vi "Tracker_Data_Analysis_tool.vi"(8 "error in (no error)":errorcluster, 11 "Settings file path":path=path "D:/Users/Dmitriy/CData/CloudStation/Tracker_repository/SubVi's/Tracker_settings.tcf") -> (0 "error out":errorcluster)   [LabVIEW 2016]
uses:
  <vilib>/Utility/config.llb/Config Data RefNum.ctl
  <vilib>/Utility/miscctls.llb/LVPoint32TypeDef.ctl
  <vilib>/Utility/miscctls.llb/LVPointTypeDef.ctl
  <vilib>/Utility/miscctls.llb/LVOffsetAndMultiplierTypeDef.ctl
  <vilib>/Utility/miscctls.llb/LVRangeTypeDef.ctl
  <vilib>/Platform/TimedLoop/XDataNode/timing_clust.ctl
  <vilib>/Platform/TimedLoop/XDataNode/nitl_modes.ctl
  <vilib>/Platform/TimedLoop/XDataNode/wakeup.ctl
  <vilib>/Utility/miscctls.llb/LVBoundsTypeDef.ctl
  <vilib>/Utility/miscctls.llb/LVStringsAndValuesArrayTypeDef_U16.ctl
  <vilib>/Instr/_visa.llb/VISA Flush IO Buffer Mask.ctl
  <extravilib>/ChannelInstances/Lossy Stream-a[.,.](str)/Write With Abort.vi
  <extravilib>/ChannelInstances/Lossy Stream-a[.,.](str)/Read With Abort.vi
  <extravilib>/ChannelInstances/Lossy Stream-a[.,.](str)/Endpoint.vi
  SubVi's/SW_Globals.vi
  <vilib>/Platform/TimedLoop/scheduler/LVUserAPI/_suppVIs/Create_1kHz_TSource.vi
  <extravilib>/ChannelInstances/Lossy Stream-a[.,.](str)/Instantiate.vi
  <vilib>/Utility/file.llb/Write Delimited Spreadsheet (string).vi
  <vilib>/Utility/file.llb/Read Delimited Spreadsheet (string).vi
  <extravilib>/ChannelInstances/Lossy Stream-a[.,.](str)/)Channel.vi
  <resource>/ChannelSupport/_ChannelSupport/WaitIfNeeded.vi
  <vilib>/platform/TimedLoop/XDataNode/XDataNode.xnode
  <vilib>/Utility/config.llb/NI_LVConfig.lvlib
  <extravilib>/ChannelInstances/Lossy Stream-a[.,.](str).lvlib
  <vilib>/Platform/TimedLoop/XDataNode/XDNodeRunTimeDep.lvlib
  <vilib>/Analysis/NI_AALBase.lvlib
panel:
  in  "Pause, s":sgl min=0 max=10000 step=0.1 format="%#_3g"
  in  "Stim., s":sgl min=0 max=10000 step=0.1
  in  "Running, s":sgl min=0 max=10000 step=0.1 format="%#_3g"
  in  "Save files First Call":bool=TRUE
  in  "Record start First Call":bool=TRUE
  out "mean 3":dbl format="%0.2f"
  out "standard deviation 3":dbl format="%0.2f"
  out "Save iteration duration":i64
  out "standard deviation":dbl format="%0.2f"
  out "mean":dbl format="%0.2f"
  in  "Type of histogram":u8
  out "TTL 4 counter":u32
  out "TTL 3 counter":u32
  out "TTL 2 counter":u32
  out "TTL 1 counter":u32
  out "Full track plotting":u32
  out "Full track preparation":u32
  out "Main queue":refnum<queue>
  out "Data flow controls":T1
  in  "Map index (analysis)":i32
  in  "Full trace color":u32(colorbox)=16711680
  out "Current TTL status":u8
  out "TTL inputs":u8[](array[numeric])
  out "TTL outputs":u8[](array[numeric])
  out "Start/Stop in config":u32
  out "Start/Stop out pulses config":u32
  out "Changed IO":bool
  out "Sync capability":u8
  in  "IO parameters string":string
  out "Reset STIM":bool
  out "Reset REG":bool
  out "Init plot":bool=TRUE
  out "Zones preference array (loaded)":dbl[][](array[numeric])
  out "Current zone":dbl[](array[numeric])
  out "Absolute timestamp (rec)":dbl[](array[numeric])
  in  "Colors for Stim. setup":T2(array[cluster])=[{"Not Selected"=1143775, "Not Selected"=1143775}, {"Not Selected"=14517504, "Not Selected"=14517504}, {"Not Selected"=1976113, "Not Selected"=1976113}, {"Not Selected"=2575993, "Not Selected"=2575993}]
  out "Record":bool
  out "Stopped":bool
  out "Reset starting pulse":bool
  out "TTL is long enough":bool
  out "Started":bool
  out "Coords":T3={"Horizontal"=316, "Vertical"=127}
  out "Button":u16=1
  out "Settings file path":path
  out "Track path":path
  out "Index of the last recorded timepoint":i32
  out "ceil(x): smallest int >= x":dbl
  out "Application Directory":path
  out "Path to the settings file":path=path "D:/Users/Dmitriy/CData/CloudStation/Tracker_repository/Tracker_settings.tcf"
  out "Eff. save interval":sgl=7.981
  out "Relative timestamp (rec)":dbl[](array[numeric])
  out "alpha rot. angle":dbl[](array[numeric])
  out "Y coord":dbl[](array[numeric])
  out "X coord":dbl[](array[numeric])
  out "Data column names":string[](array[string])
  out "Zones allocation array":i32[](array[numeric])
  out "Zones presence array":bool[](array[boolean])
  in  "Stop Button":bool
  out "Path to the latest saved temp file":path
  out "Temp file ready":bool
  out "Pixels per mm":dbl=1.1663076923076923
  out "Settings file refnum out":T4
  out "Current User":string="Researcher"
  in  "Main tab control":enum32{"Settings", "Recording", "Analysis"}(tab)
  in  "Set advanced stimulus":bool
  in  "Load zones":bool
  in  "Load stimuli":bool
  in  "Load settings":bool
  out "IO status indicator":T5
  in  "Set IO config":bool
  in  "Jump to Analysis":bool
  in  "Reset stimuli":bool
  in  "Stimulus presets":T6(array[cluster]) {"TTL out" items=["1"=1, "2"=2, "1 + 2"=3]; "Stimulus, s" min=0 max=10000 step=0.1; "Time, s" min=0 max=10000 step=0.1; "Event type" items=["Time spent in zone", "Future options"]}
  in  "Zone-based stimulus setup":T7(radio)=enum."Zone 13"
  out "Ready":bool=TRUE
  in  "Re-check HW connection":bool
  in  "Reset regions":bool
  in  "Start Tracking button":bool
  in  "Starting angle BORDER":i16
  in  "N segments BORDER":u8=5 max=8
  in  "N segments MIDFIELD":u8=3 min=1 max=4
  in  "Starting angle MIDFIELD":i16=30
  in  "Radius, mm MIDFIELD":u16=110
  in  "Radius, mm CENTER":u16=50 min=5 step=1
  out "Board size":string="Large"
  in  "Cage diameter, mm":u16(ring)=333 items=["180 mm"=180, "325 mm"=325, "327 mm"=327, "333 mm"=333]
  out "Segments diagram":picture
  out "HW info":string
  out "Port":string="Large"
  out "Run times distrib. indicator":bool
  out "IO pulses count":string
  in  "Bridge swap":bool
  in  "Reset barplot":bool
  out "Mouse speed digi":dbl=0.28949046360238656 caption="Mouse speed" format="%05.1f"
  out "Histograms (normalized)":dbl[](graph)=[0.0, 0.0, 0.0, 0.0, 0.0, 0.0, 1.0, 0.0, 0.0, 0.0, 0.0] caption="Run times dist. hist. (norm.)"
  in  "Multiplyer of chart RX":u8(slide)=1 min=1 max=10 step=1 scale=1.0..6.0
  in  "Zones presence indicator":T8={"01"=TRUE, "02"=TRUE, "03"=TRUE, "04"=TRUE, "05"=TRUE, "06"=TRUE, "07"=TRUE, "08"=TRUE, "09"=TRUE, "10"=TRUE, "11"=TRUE, "12"=TRUE, "13"=TRUE}
  in  "Zones":bool=TRUE
  in  "Record/Stop":bool
  out "Diagram at recording":picture caption="Mouse track"
  in  "Trace, s":u16(slide)=5 max=30 step=1 scale=0.0..30.0
  in  "Data filtering":u16(ring)=5 items=["None"=0, "Kalman 1/3"=2, "Kalman 1/8"=3, "SG 3/5"=4, "SG 3/11"=5, "SG 3/31"=6]
  out "Record timestamp":dbl format="%<%H:%M:%S%3u>t"
  out "Current Time":timestamp=timestamp(3610093053.229 s since 1904-01-01) format="%<%H:%M:%S %d.%m.%Y>T"
  in  "Exit (recording)":bool
  out "Mouse speed":waveform(dbl)(graph)={"t0"=timestamp(3610093053.229 s since 1904-01-01), "dt"=1.0, "Y"=[0.28949046360238656]}
  in  "Vertical offset":sgl caption="Bridge offset" min=-60 max=60 step=0.1 format="%#.1g"
  out "TTL IO 1 (recording)":bool caption="IO 1"
  out "TTL IO 2 (recording)":bool caption="IO 2"
  out "TTL IO 3 (recording)":bool caption="IO 3"
  out "TTL IO 4 (recording)":bool caption="IO 4"
  out "TTL REC":bool
  out "Mouse running, perc. of time":dbl=0.28949046360238656 caption="Run, %" format="%05.2f"
  out "Zones presense indicator":bool
  out "Speed distrib. indicator":bool
  out "Run lengts distrib. indicator":bool
  in  "Back to Settings":bool
  out "Data loading progress":dbl(slide) scale=0.0..100.0
  in  "Speed":u16(ring)=3 items=["25"=75, "10"=30, "6"=18, "4"=12, "2"=6, "1"=3, "2/3"=2, "1/3"=1]
  in  "Timeline":dbl(slide) min=0.0 step=1.0 scale=0.0..2699.993 scale format="%<%H:%M:%S>t"
  in  "Multiplyer of chart RX 2":u8(slide)=1 min=1 max=10 step=1 scale=1.0..6.0
  out "Diagram at analysis":picture caption="Mouse track"
  in  "Play/Pause":bool
  out "Recorded at time":timestamp format="%<%H:%M:%S %d.%m.%Y>T"
  out "Recorded timestamp":dbl format="%<%H:%M:%S%3u>t"
  in  "Zones (analysis)":bool=TRUE caption="Zones"
  out "Mouse speed 2":waveform(dbl)(graph) caption="Mouse speed"
  out "Mouse speed digi 2":dbl format="%05.1f"
  out "Zones allocation (normalized) in analysis":dbl[](graph) caption="Zone preference (normalized)"
  out "Recorded by":string
  in  "Trace in analysis, s":u16(slide)=2 caption="Trace, s" max=30 step=1 scale=0.0..30.0
  in  "Open File":bool
  out "Mouse snout orientation swap (analysis)":bool caption="Swapped"
  in  "Show heatmap (analysis)":bool caption="Heat map"
  in  "Show full track (analysis)":bool caption="Full track"
  out "Vertical offset (analysis)":sgl caption="Br. offset" min=-60 max=60 step=0.1 format="%#.1g"
  out "TTL IO 2 (analysis)":bool
  out "TTL IO 1 (analysis)":bool
  out "TTL IO 3 (analysis)":bool
  out "TTL IO 4 (analysis)":bool
  # "v.2.1.5"
  # "Cage segmentation"
  # "BORDER"
  # "CENTER"
  # "MIDFIELD"
  # "v.2.1.5"
  # "v.2.1.5"
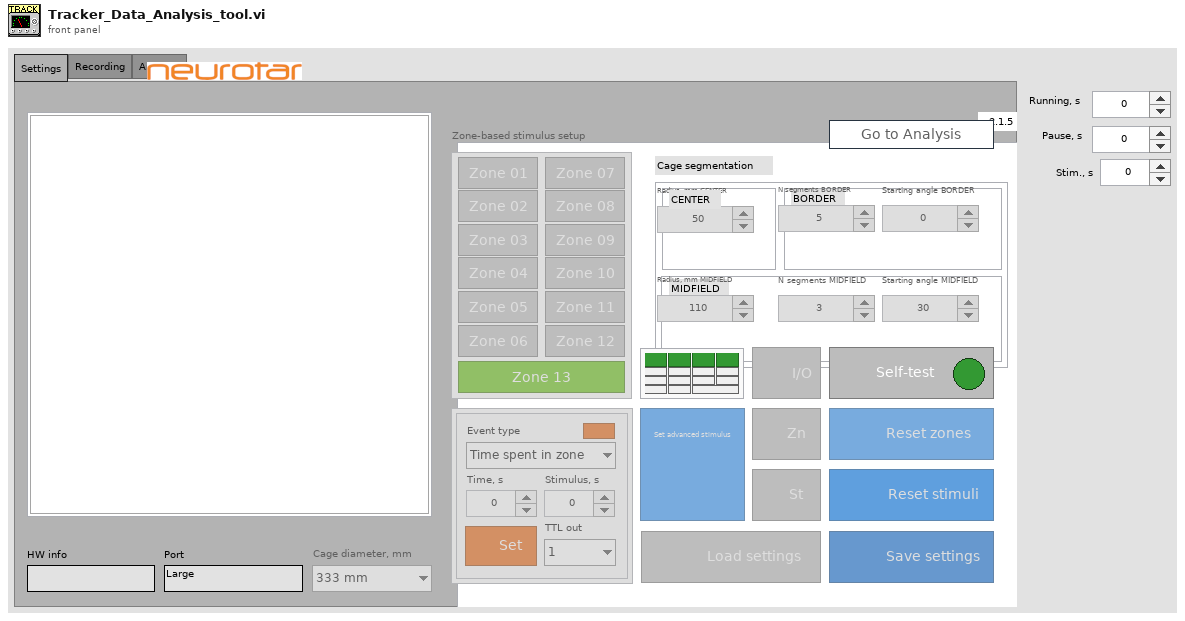
[diagram p1: front panel]
types:
  T1 = cluster{"Data acquisition status":refnum<notifier>, "Play/Pause status":refnum<notifier>, "Complete stop":refnum<notifier>, "Temp file ready for processing":refnum<notifier>, "Has been recorded":refnum<notifier>, "Recording now":refnum<notifier>, "Path to the latest complete temp file":refnum<notifier>, "Final CSV saved":refnum<notifier>, "Data loaded":refnum<notifier>}
  T2 = cluster{"Not Selected":u32, "Not Selected":u32}[]
  T3 = typedef "LVPoint32TypeDef.ctl" = cluster{"Horizontal":i32, "Vertical":i32}
  T4 = typedef "NI_LVConfig.lvlib/Config Data RefNum.ctl" = refnum<k1>
  T5 = cluster{"IO1":bool, "IO2":bool, "IO3":bool, "IO4":bool, "Z1":bool, "Z2":bool, "Z3":bool, "Z4":bool, "St1":bool, "St2":bool, "St3":bool, "St4":bool, "Syn1":bool, "Syn2":bool, "RS-232 ext. activated":bool}
  T6 = cluster{"Event type":u16, "Time, s":sgl, "Stimulus, s":sgl, "Set/Clear":bool, "TTL out":u16, "Stim. has been set":bool}[]
  T7 = enum32{"No Selection", "Zone 01", "Zone 02", "Zone 03", "Zone 04", "Zone 05", "Zone 06", "Zone 07", "Zone 08", "Zone 09", "Zone 10", "Zone 11", "Zone 12", "Zone 13"}
  T8 = cluster{"01":bool, "02":bool, "03":bool, "04":bool, "05":bool, "06":bool, "07":bool, "08":bool, "09":bool, "10":bool, "11":bool, "12":bool, "13":bool}
  T9 = cluster{"Numeric Control":u32, "Numeric Control":u32}[]
  T10 = enum8{"Enabled", "Disabled", "Disabled and Grayed Out"}
  T11 = typedef "XDNodeRunTimeDep.lvlib/timing_clust.ctl" = cluster{"Expected End [f-1]":u64, "Actual End [f-1]":u64, "Finished Late? [f-1]":bool, "Expected End [i-1]":u64, "Actual End [i-1]":u64, "Finished Late? [i-1]":bool, "Expected Start [i]":u64, "Actual Start [i]":u64, "Expected Start [f]":u64, "Actual Start [f]":u64, "Source Name":string, "Structure Name":string, "Period":i64, "Deadline":i64, "Offset":i64, "Start":i64, "Priority":i32, "Timeout":i32, "Mode":T12, "Wakeup Reason":T13, "Error":errorcluster, "Source Type":string, "Secondary Source Type":string, "Global End Time":u64, "Global Start Time":u64, "Frame Duration":u64, "Iteration Duration":u64, "Assigned CPU":i32, "I/O Scan Engine Mode":u32}
  T12 = typedef "XDNodeRunTimeDep.lvlib/nitl_modes.ctl" = enum32{"No Change", "Process missed periods, maintain original phase", "Discard missed periods, maintain original phase", "Process missed periods, ignore original phase", "Discard missed periods, ignore original phase"}
  T13 = typedef "XDNodeRunTimeDep.lvlib/wakeup.ctl" = enum32{"Normal", "Aborted", "Asynchronous wakeup", "Timing source error", "Timed loop error", "Timeout"}
  T14 = cluster{"Read buffer":string, "Timestamp":timestamp}
  T15 = typedef "VISA Flush IO Buffer Mask.ctl" = u16
  T16 = typedef "LVBoundsTypeDef.ctl" = cluster{"Width":u32, "Height":u32}
  T17 = cluster{"Amount of border segments":u8, "Border segments starting angle":i16, "Amount of midfield segments":u8, "Midfield segments starting angle":i16, "Midfield segments outer radius, mm":u16, "Amount of central segments":u8, "Center segment outer radius, mm":u16, "Diameter of the cage, mm":u16, "R-gap between segments, mm":u8}
  T18 = typedef "LVRangeTypeDef.ctl" = cluster{"Minimum":dbl, "Maximum":dbl, "Increment":dbl, "Minor Increment":dbl, "Start":dbl}
  T19 = cluster{"Temporary file output path":path, "Temporary csv output path":path, "Recording settings output path":path, "Final csv output path":path, "Background picture output path":path, "Path to the settings file":path, "Path to TDMS file":path, "TDMS file reference":refnum<k34>}
  T20 = cluster{"Zones preference array (loaded)":dbl[][], "TTL inputs":u8[], "TTL outputs":u8[], "Stimulus presets array (loaded)":cluster{"Event type":u16, "Time, s":sgl, "Stimulus, s":sgl, "Set/Clear":bool, "TTL out":u16, "Stim. has been set":bool}[], "Absolute timestamp":dbl[], "Relative timestamp":dbl[], "X coord":dbl[], "Y coord":dbl[], "alpha rot. angle":dbl[], "Current zone":dbl[], "Acquisition settings cluster out":cluster{"Researcher name":string, "Amount of midfield segments":u32, "Amount of border segments":u32, "Center segment outer radius, mm":u32, "Midfield segments outer radius, mm":u32, "Midfield segments starting angle":i32, "Border segments starting angle":i32, "Cage diameter, mm":u32, "Mouse snout orientation swap?":bool, "Vertical offset":dbl, "Settings loaded OK":bool}, "Data column names":string[]}
  T21 = cluster{"Researcher name":string, "Amount of midfield segments":u32, "Amount of border segments":u32, "Center segment outer radius, mm":u32, "Midfield segments outer radius, mm":u32, "Midfield segments starting angle":i32, "Border segments starting angle":i32, "Cage diameter, mm":u32, "Mouse snout orientation swap?":bool, "Vertical offset":dbl, "Settings loaded OK":bool}
  T22 = cluster{"Fonts scale factor":dbl, "Pixels per mm":dbl, "Radius of displayed outer segments, pix":dbl, "Radius of displayed midfield segments, pix":dbl, "Radius of displayed central segment, pix":dbl}
  T23 = typedef "imagedata.ctl" = cluster{"image type":i32, "image depth":i32, "image":u8[], "mask":u8[], "colors":u32[], "Rectangle":cluster{"left":i16, "top":i16, "right":i16, "bottom":i16}}
  T24 = cluster{"Width":u16, "Style":enum32{"Solid", "Dash", "Dot", "DashDot", "DashDotDot"}}
  T25 = cluster{"N segments BORDER":u8, "Starting angle BORDER":i16, "N segments MIDFIELD":u8, "Starting angle MIDFIELD":i16, "Radius, mm MIDFIELD":u16, "Amount of central segments":u8, "Radius, mm CENTER":u16}
  T26 = typedef "LVOffsetAndMultiplierTypeDef.ctl" = cluster{"Offset":dbl, "Multiplier":dbl}
  T27 = enum32{"No Selection", "Zone 01", "Zone 02", "Zone 03", "Zone 04", "Zone 05", "Zone 06", "Zone 07", "Zone 08", "Zone 09", "Zone 10", "Zone 11", "Zone 12", "Zone 13", "Zone 14"}
  T28 = enum32{"Page Enabled", "Page Disabled", "Page Disabled & Grayed"}
  T29 = typedef "LVPointTypeDef.ctl" = cluster{"Horizontal":i16, "Vertical":i16}
  T30 = enum32{"invalid app kind", "Development System", "Run Time System", "Student Edition", "Embedded LabVIEW", "Evaluation", "Custom"}
  T31 = cluster{"Event type":u16, "Dur., s":sgl, "Stim., s":sgl, "Set/Clear":bool, "TTL out N":u16, "Stim. has been set":bool}[]
  T32 = cluster{"SYNC configuration":u16, "IO 1 configuration":u16, "IO 2 configuration":u16, "IO 3 configuration":u16, "IO 4 configuration":u16, "Activate ext. RS-232":u16, "IO inversion config.":u16}
  T33 = typedef "Lossy Stream-a[.,.](str).lvlib/)Channel.ctl" = refnum<queue>
  T34 = cluster{"Read buffer":string, "Timestamp":timestamp}[]
  T35 = cluster{"Event type":u16, "Cond., s":sgl, "Stim., s":sgl, "Set/Clear":bool, "TTL out N":u16, "Stim. has been set":bool}
  T36 = cluster{"SYNC configuration":bool, "IO 1 configuration":bool, "IO 2 configuration":bool, "IO 3 configuration":bool, "IO 4 configuration":bool, "Activate ext. RS-232":bool, "IO inversion config.":bool}
  T37 = cluster{"Event type":u16, "Time, s":sgl, "Stimulus, s":sgl, "Set/Clear":bool, "TTL out":u16, "Stim. has been set":bool}
  T38 = typedef "LVStringsAndValuesArrayTypeDef_U16.ctl" = cluster{"String":string, "Value":u16}[]
  T39 = cluster{"N segments BORDER":u8, "Starting angle BORDER":i16, "N segments MIDFIELD":u8, "Starting angle MIDFIELD":i16, "Radius, mm MIDFIELD":u16, u8, "Radius, mm CENTER":u16, "Cage diameter, mm":u16, i32}
  T40 = cluster{"N segments BORDER":u8, "Starting angle BORDER":i16, "N segments MIDFIELD":u8, "Starting angle MIDFIELD":i16, "Radius, mm MIDFIELD":u16, "N segments CENTER":u8, "Radius, mm CENTER":u16, "Cage diameter, mm":u16, "R-gap":i32}
  T41 = cluster{"Zone[1]":bool, "Zone[2]":bool, "Zone[3]":bool, "Zone[4]":bool, "Zone[5]":bool, "Zone[6]":bool, "Zone[7]":bool, "Zone[8]":bool, "Zone[9]":bool, "Zone[10]":bool, "Zone[11]":bool, "Zone[12]":bool, "Zone[13]":bool}
  T42 = cluster{"Event type":u16, "Cond., s":sgl, "Stim., s":sgl, "Set/Clear":bool, "TTL out N":u16, "Stim. has been set":bool}[]
  T43 = cluster{"Temporary file output path":path, "Temporary csv output path":path, "Recording settings output path":path, "Final output path":path, "Background picture output path":path, "Path to the settings file":path, "Path to TDMS file":path, "TDMS file reference":refnum<k34>}
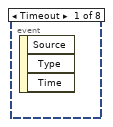
[diagram p5: hidden frame]
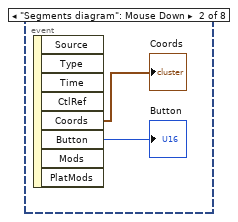
[diagram p6: hidden frame]
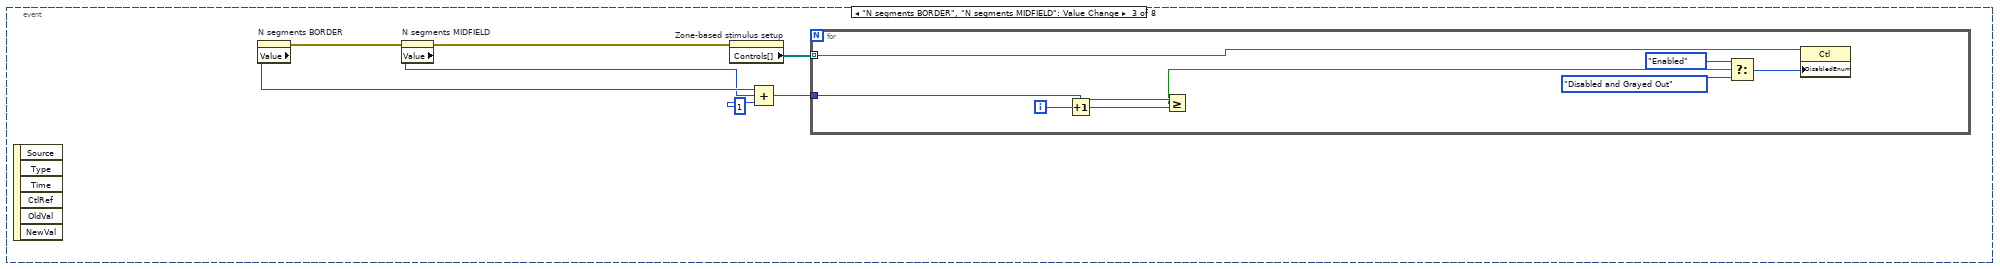
[diagram p7: hidden frame]
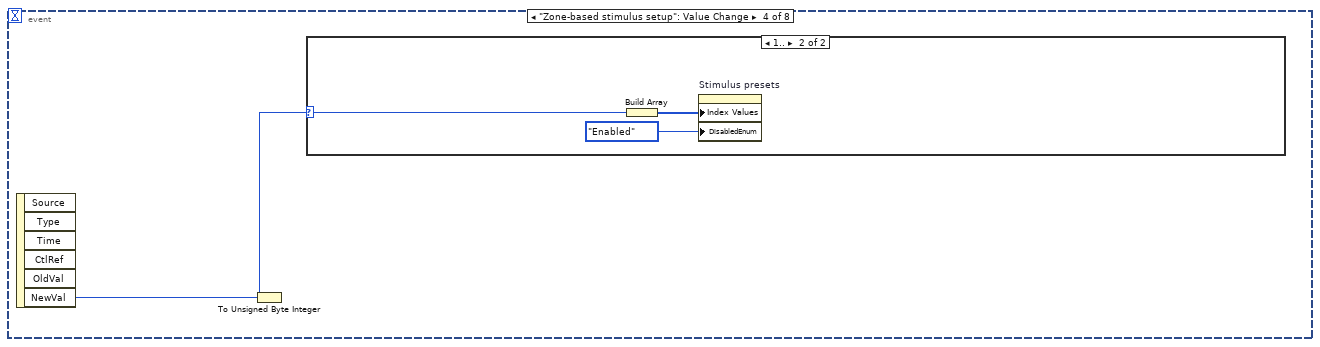
[diagram p8: hidden frame]
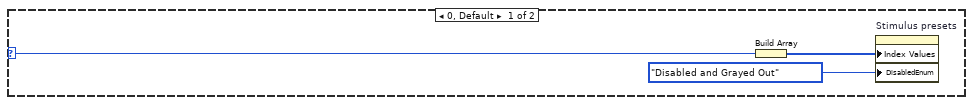
[diagram p9: hidden frame]
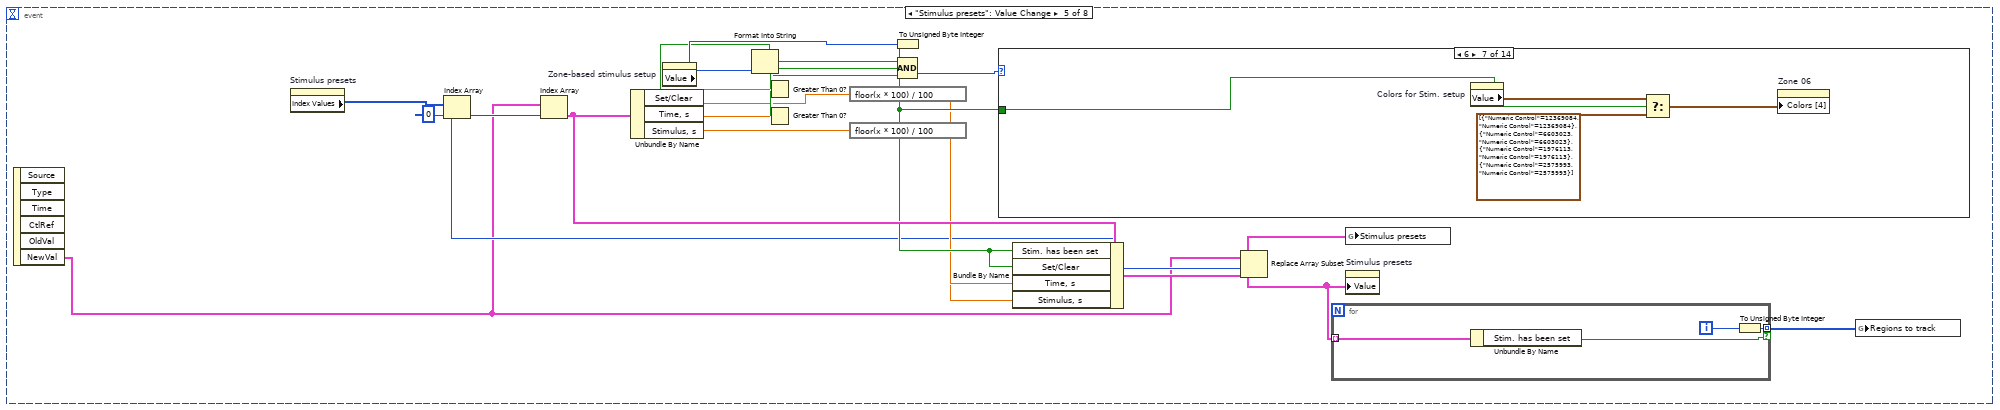
[diagram p10: hidden frame]
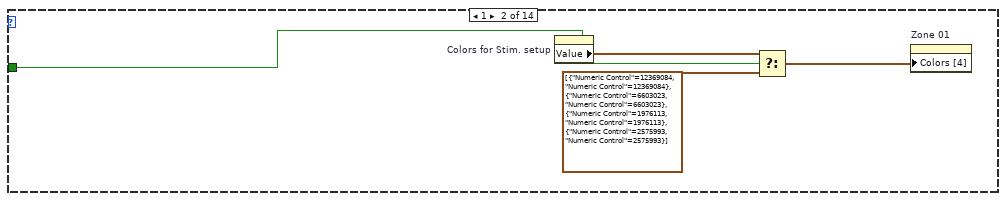
[diagram p12: hidden frame]
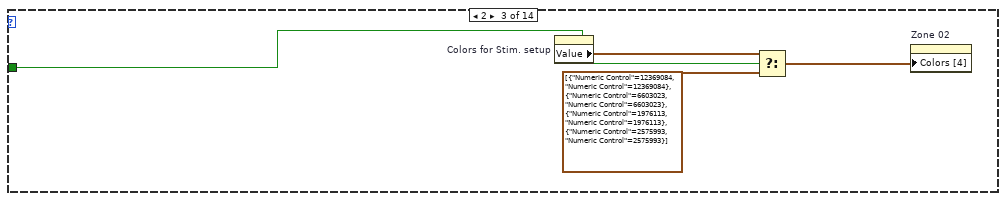
[diagram p13: hidden frame]
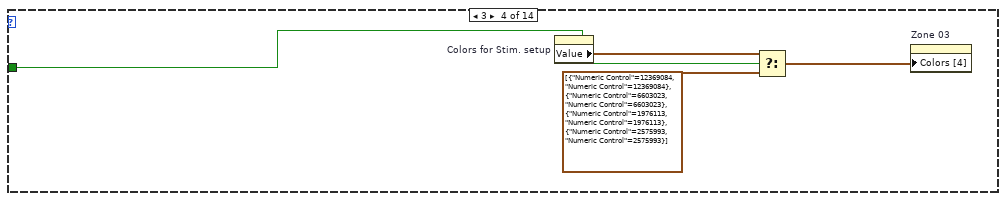
[diagram p14: hidden frame]
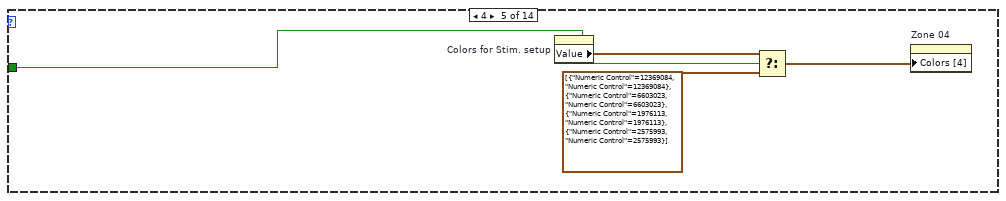
[diagram p15: hidden frame]
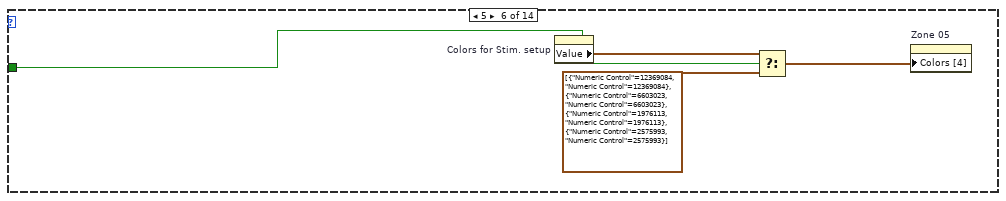
[diagram p16: hidden frame]
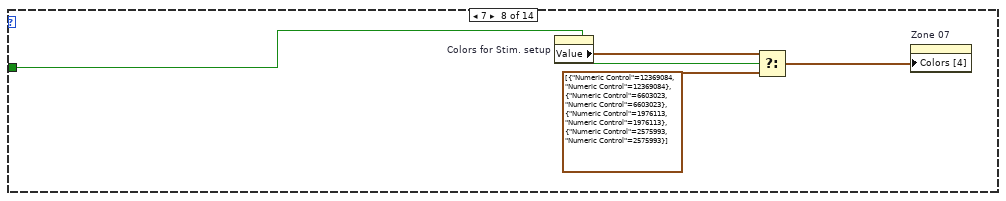
[diagram p17: hidden frame]
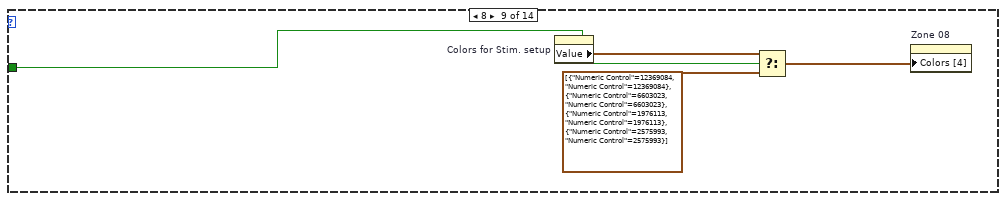
[diagram p18: hidden frame]
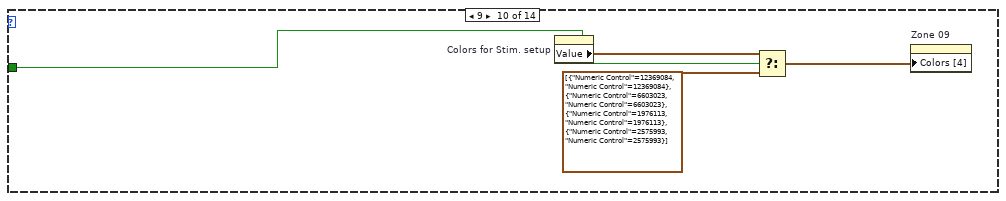
[diagram p19: hidden frame]
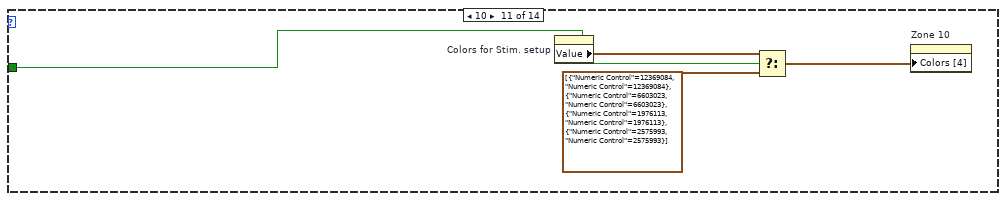
[diagram p20: hidden frame]
diagram:
  w10 = i64 37 ("Period")
  w23 = i64 23 ("Period")
  n1 = node-c288(w3, i64 1 ("Period"), 65000 ("Priority")) -> (w32:T11)
  n2 = disable-structure shown="Default" {
    disable-tunnel: [w45] -> w7
    frame Enabled {
      w44 = T10."Disabled and Grayed Out" ("Disabled")
      n3 = property on="Cage diameter, mm" class="Ring (strict)"("DisabledEnum"=w44) -> ()  [unwired: 2 in, 2 out]
      n4 = property on="Set IO config" class="Bool"("DisabledEnum"=w44) -> ()  [unwired: 2 in, 2 out]
      n5 = property on="Starting angle MIDFIELD" class="DigNum (strict)"("DisabledEnum"=w44) -> ()  [unwired: 2 in, 2 out]
      n6 = property on="N segments MIDFIELD" class="DigNum (strict)"("DisabledEnum"=w44) -> ()  [unwired: 2 in, 2 out]
      n7 = property on="Radius, mm MIDFIELD" class="DigNum (strict)"("DisabledEnum"=w44) -> ()  [unwired: 2 in, 2 out]
      n8 = property on="Starting angle BORDER" class="DigNum (strict)"("DisabledEnum"=w44) -> ()  [unwired: 2 in, 2 out]
      n9 = property on="N segments BORDER" class="DigNum (strict)"("DisabledEnum"=w44) -> ()  [unwired: 2 in, 2 out]
      n10 = property on="Radius, mm CENTER" class="DigNum (strict)"("DisabledEnum"=w44) -> ()  [unwired: 2 in, 2 out]
      n11 = property on="Start Tracking button" class="Bool"("DisabledEnum"=w44) -> ()  [unwired: 2 in, 2 out]
      n12 = property on="Reset stimuli" class="Bool (strict)"("DisabledEnum"=w44) -> ()  [unwired: 2 in, 2 out]
      n13 = property on="Reset regions" class="Bool (strict)"("DisabledEnum"=w44) -> (error out=w45:errorcluster)  [unwired: 2 in, 1 out]
      n14 = property on="Zone-based stimulus setup" class="RadioBtnsControl (strict)"("DisabledEnum"=w44) -> ()  [unwired: 2 in, 2 out]
      n15 = property on="Set advanced stimulus" class="Bool (strict)"("DisabledEnum"=w44) -> ()  [unwired: 2 in, 2 out]
    }
  }
  n16 = property on="Re-check HW connection" class="Bool"(error in=w7, "DisabledEnum"=T10."Disabled and Grayed Out" ("Disabled")) -> (error out=w37:errorcluster)  [unwired: 1 in, 1 out]
  n17 = property on="Ready" class="Bool (strict)"(error in=w37, "Value"=FALSE ("Ready"), "Colors [4]"=T9 [{"Numeric Control"=16749459, "Numeric Control"=16749459}, {"Numeric Control"=1988894, "Numeric Control"=3381555}, {"Numeric Control"=4934475, "Numeric Control"=7895160}, {"Numeric Control"=994319, "Numeric Control"=1657881}]) -> (error out=w2:errorcluster)  [unwired: 1 in, 1 out]
  n18 = node-c288(w3, i64 1201 ("Period"), 50 ("Priority")) -> (w21:T11)
  n19 = timed-loop {
    tunnel: w43 -> [w65]
    tunnel: [w48] -> w8
    tunnel: [w64] -> w5
    tunnel: [w49] -> w39
    tunnel: [w63] -> w6
    tunnel: w2 -> [w59]
    tunnel: [w52] -> w33
    timing: w21 -> [_]
    timing-out: [_] -> w20
    stop <- w47 stop-if-true
    n20 = node-c288() -> ()  [unwired: 1 in, 1 out]
    n21 = property on="Re-check HW connection" class="Bool"(error in=w59, "DisabledEnum"=T10."Enabled" ("Disabled")) -> (error out=w58:errorcluster)  [unwired: 1 in, 1 out]
    n22 = First Call?() -> (First Call?: T/F=w50:bool)
    n23 = property on="Ready" class="Bool (strict)"(error in=w58) -> (error out=w62:errorcluster, "Value"=w61:bool)  [unwired: 1 in, 1 out]
    n24 = Or(x=w50, y="Re-check HW connection") -> (x .or. y?=w51:bool)
    n25 = Not(x=w61) -> (.not. x?=w57:bool)
    n26 = And(x=w57, y=w51) -> (x .and. y?=w56:bool)
    n27 = case shown="True" w56 {
      tunnel: w65 -> [w71 w98]
      tunnel: [w68 w97] -> w64
      tunnel: [w71 w96] -> w49
      tunnel: [w69 w95] -> w63
      tunnel: [w72 w81] -> w53
      tunnel: [FALSE ("Instrument OK?") w85] -> w48
      tunnel: w62 -> [w72 w83]
      frame False {
        n28 = local read "Data flow controls"() -> (w69:T1)
        n29 = local read "Main queue"() -> (w68:refnum<queue>)
      }
      frame True {
        w94 = T14 {"Read buffer"="", "Timestamp"=timestamp(3605695211.9516535 s since 1904-01-01)}  # Data frame example
        n30 = property on="Ready" class="Bool (strict)"(error in=w83, "Colors [4]"=T9 [{"Numeric Control"=16749459, "Numeric Control"=16176658}, {"Numeric Control"=1988894, "Numeric Control"=3381555}, {"Numeric Control"=4934475, "Numeric Control"=7895160}, {"Numeric Control"=994319, "Numeric Control"=1657881}]) -> (error out=w82:errorcluster)  [unwired: 1 in, 1 out]
        n31 = Obtain Queue(name (unnamed)="Data flow", element data type=w94, error in (no error)=w82) -> (queue out=w97:refnum<queue>, error out=w92:errorcluster)  [unwired: 2 in, 1 out]
        "Main queue" <- w97
        n32 = call "HW_Setup.vi"("VISA resource name in"=w98, "Traget FPS"=80, "error in"=w92) -> ("error out"=w81:errorcluster, "Sensor board size"=w73:string, "VISA resource name out"=w96:refnum<visa-resource-name>, "Data flow controls"=w95:T1, "Version information"=w80:string, "Instrument OK?"=w85:bool)  [unwired: 1 in, 1 out]
        "Ready" <- w85
        "Board size" <- w73
        "Data flow controls" <- w95
        n33 = String Length(string=w80) -> (length=w89:i32)
        n34 = Equal?(x=w80, y="1.1.4") -> (x = y?=w77:bool)
        n35 = Greater Than 0?(x=w89) -> (x > 0?=w88:bool)
        n36 = Concatenate Strings(w73, ", FW: " ("string"), w80) -> (w87:string)
        n37 = Select(t=u8 0, s=w77, f=u8 1) -> (s? t:f=→"Sync capability":u8)
        n38 = Select(t=w87, s=w88, f="Not connected") -> (s? t:f=→"HW info":string)
      }
    }
    n39 = property on="Jump to Analysis" class="Bool (strict)"() -> ("Value"=w46:bool)  [unwired: 2 in, 2 out]
    n40 = Or(x=w48, y=w46) -> (x .or. y?=w47:bool)
    n41 = global write "SW_Globals.vi" "VISA resource name"(w49) -> ()
    n42 = property on="Ready" class="Bool (strict)"(error in=w53, "Colors [4]"=T9 [{"Numeric Control"=16749459, "Numeric Control"=16749459}, {"Numeric Control"=1988894, "Numeric Control"=3381555}, {"Numeric Control"=4934475, "Numeric Control"=7895160}, {"Numeric Control"=994319, "Numeric Control"=1657881}]) -> (error out=w52:errorcluster)  [unwired: 1 in, 1 out]
    n43 = node-c288() -> ()  [unwired: 1 in, 1 out]
  }
  n44 = node-c288(w20) -> ()  [unwired: 1 out]
  n45 = property on="Re-check HW connection" class="Bool"(error in=w33, "DisabledEnum"=T10."Disabled and Grayed Out" ("Disabled")) -> (error out=w1:errorcluster)  [unwired: 1 in, 1 out]
  n46 = timed-loop "In this loop raw data from the device is obtained and TTLs are fired" {
    tunnel: w39 -> [w121]
    tunnel: w1 -> [w120]
    tunnel: w6 -> [w101]
    tunnel: w5 -> [w125]
    timing: w32 -> [_]
    timing-out: [_] -> w31
    stop <- w102 stop-if-true
    # "In this loop raw data from the device is obtained and TTLs are fired"
    n47 = node-c288() -> (w119:i64)  [unwired: 1 in]
    n48 = Unbundle By Name(w101) -> ("Complete stop"=w109:refnum<notifier>, "Recording now"=w108:refnum<notifier>, "Has been recorded"=w107:refnum<notifier>)
    n49 = disable-structure shown="Disabled" {
      disable-tunnel: w119 -> [w152 _]
      frame Disabled {
        n50 = Build Array(w152) -> (w150:i64[])
        n51 = call "FL_Last_N_Samples_1D.vi"("BufferLengthSamples"=u32 500, "Input Array of strings"=w150) -> ("Output Array of strings"=w151:dbl[])
        n52 = call <vilib>:"Std Deviation and Variance.vi"("X"=w151) -> ("mean"=→"mean":dbl, "standard deviation"=→"standard deviation":dbl)  [unwired: 1 in, 1 out]
      }
      frame Enabled {
      }
    }
    n53 = property on="Start/Stop out pulses config" class="DigNum (strict)"() -> ("Value"=w122:u32)  [unwired: 2 in, 2 out]
    n54 = Get Notifier Status(notifier=w107) -> (current notification=w106:bool)  [unwired: 1 in, 4 out]
    n55 = Get Notifier Status(notifier=w109) -> (current notification=w102:bool)  [unwired: 1 in, 4 out]
    n56 = Get Notifier Status(notifier=w108) -> (current notification=w104:bool)  [unwired: 1 in, 4 out]
    n57 = Not(x=w104) -> (.not. x?=w103:bool)
    n58 = Greater Than 0?(x=w122) -> (x > 0?=w123:bool)
    n59 = And(x=w103, y=w106) -> (x .and. y?=w105:bool)
    n60 = Or(x=w105, y=w102) -> (x .or. y?=w129:bool)
    n61 = case "Inside this case structure TTL can be fired at the start of the recording" shown="True" w104 {
      tunnel: w123 -> [_ w165]
      tunnel: w120 -> [w155 w164]
      tunnel: [w155 w163] -> w126
      tunnel: w121 -> [w156 w162]
      tunnel: [w156 w161] -> w128
      tunnel: [w154 w160] -> w127
      tunnel: w125 -> [w154 w159]
      tunnel: w122 -> [_ w158]
      frame False {
        n62 = First Call?() -> (First Call?: T/F=w153:bool)
        n63 = case shown="True" w153 {
          frame False {
          }
          frame True {
            n64 = Get Date/Time In Seconds() -> (seconds since 1Jan1904=w157:timestamp)
            n65 = global write "SW_Globals.vi" "Recording start timestamp"(w157) -> ()
          }
        }
      }
      frame True {
        n66 = First Call?() -> (First Call?: T/F=w166:bool)
        n67 = case shown="True" w166 {
          tunnel: w165 -> [_ w185]
          tunnel: w164 -> [w169 w184]
          tunnel: [w169 w179] -> w163
          tunnel: w162 -> [w168 w183]
          tunnel: [w168 w182] -> w161
          tunnel: [w167 w180] -> w160
          tunnel: w159 -> [w167 w181]
          tunnel: w158 -> [_ w171]
          tunnel: w158 -> [_ w170]
          frame False {
          }
          frame True {
            n68 = flat-sequence {
              tunnel: w181 -> [w198]
              tunnel: w183 -> [w199]
              tunnel: w184 -> [w196]
              tunnel: w185 -> [w197]
              tunnel: [w197] -> w178
              tunnel: [w196] -> w177
              tunnel: [w199] -> w176
              tunnel: [w198] -> w175
              tunnel: w170 -> [w186]
              tunnel: [w204] -> w174
              tunnel: [w209] -> w173
              tunnel: [w208] -> w172
              tunnel: w178 -> [w201]
              tunnel: w177 -> [w207]
              tunnel: w176 -> [w206]
              tunnel: w175 -> [w210]
              tunnel: w171 -> [w200]
              tunnel: [w221] -> w179
              tunnel: [w223] -> w180
              tunnel: [w224] -> w182
              tunnel: w172 -> [w221]
              tunnel: w173 -> [w223]
              tunnel: w174 -> [w224]
              frame #0 {
                n69 = Number To Boolean Array(number=w186) -> (Boolean array=w190:bool[])
                n70 = Index Array(array=w190, index=3) -> (element=w192:bool)
                n71 = Index Array(array=w190, index=2) -> (element=w193:bool)
                n72 = Index Array(array=w190, index=1) -> (element=w194:bool)
                n73 = Index Array(array=w190, index=0) -> (element=w195:bool)
                n74 = property on="TTL IO 4 (recording)" class="Bool (strict)"("Value"=w192) -> ()  [unwired: 2 in, 2 out]
                n75 = property on="TTL IO 3 (recording)" class="Bool (strict)"("Value"=w193) -> ()  [unwired: 2 in, 2 out]
                n76 = property on="TTL IO 2 (recording)" class="Bool (strict)"("Value"=w194) -> ()  [unwired: 2 in, 2 out]
                n77 = property on="TTL IO 1 (recording)" class="Bool (strict)"("Value"=w195) -> ()  [unwired: 2 in, 2 out]
              }
              frame #1 {
                n78 = call "SW_Fire_TTL_at_start_universal.vi"("TTL port(s) config to fire"=w200, "TTL pulse length, ms"=100.0, "error in (no error)"=w207, "Serial Port In"=w206, "Close VISA (T)"=FALSE, "Start/stop signaling (F)"=w201) -> ("error out"=w205:errorcluster, "Serial Port Out"=w204:refnum<visa-resource-name>)  [unwired: 3 in, 1 out]
                n79 = Flush Queue(queue=w210, error in (no error)=w205) -> (queue out=w209:refnum<queue>, error out=w208:errorcluster)  [unwired: 1 out]
              }
              frame #2 {
                n80 = Get Date/Time In Seconds() -> (seconds since 1Jan1904=w222:timestamp)
                n81 = Number To Boolean Array(number=u32 0) -> (Boolean array=w217:bool[])
                n82 = global write "SW_Globals.vi" "Recording start timestamp"(w222) -> ()
                n83 = Index Array(array=w217, index=2) -> (element=w214:bool)
                n84 = Index Array(array=w217, index=1) -> (element=w213:bool)
                n85 = Index Array(array=w217, index=0) -> (element=w212:bool)
                n86 = Index Array(array=w217, index=3) -> (element=w215:bool)
                n87 = property on="TTL IO 3 (recording)" class="Bool (strict)"("Value"=w214) -> ()  [unwired: 2 in, 2 out]
                n88 = property on="TTL IO 2 (recording)" class="Bool (strict)"("Value"=w213) -> ()  [unwired: 2 in, 2 out]
                n89 = property on="TTL IO 1 (recording)" class="Bool (strict)"("Value"=w212) -> ()  [unwired: 2 in, 2 out]
                n90 = property on="TTL IO 4 (recording)" class="Bool (strict)"("Value"=w215) -> ()  [unwired: 2 in, 2 out]
              }
            }
          }
        }
      }
    }
    n91 = disable-structure shown="Disabled" {
      disable-tunnel: w111 -> [w146 _]
      disable-tunnel: w110 -> [w145 _]
      frame Disabled {
        n92 = Subtract(x=w146, y=w145) -> (x-y=w140:dbl)
        n93 = Multiply(x=1000.0, y=w140) -> (x*y=w138:dbl)
        n94 = Build Array(w138) -> (w139:dbl[])
        n95 = call "FL_Last_N_Samples_1D.vi"("BufferLengthSamples"=u32 500, "Input Array of strings"=w139) -> ("Output Array of strings"=w141:dbl[])
        n96 = call <vilib>:"Std Deviation and Variance.vi"("X"=w141) -> ("mean"=→"mean 3":dbl, "standard deviation"=→"standard deviation 3":dbl)  [unwired: 1 in, 1 out]
      }
      frame Enabled {
      }
    }
    n97 = flat-sequence {
      tunnel: w126 -> [w226]
      tunnel: w127 -> [w227]
      tunnel: w128 -> [w228]
      tunnel: w101 -> [w229]
      tunnel: [w229] -> w118
      tunnel: [w228] -> w117
      tunnel: [w227] -> w116
      tunnel: [w226] -> w115
      tunnel: [w225] -> w110
      tunnel: w118 -> [w235]
      tunnel: w117 -> [w232]
      tunnel: w116 -> [w231]
      tunnel: w115 -> [w230]
      tunnel: [w236] -> w114
      tunnel: [w234] -> w113
      tunnel: [w233] -> w112
      tunnel: [w238] -> w132
      tunnel: [w239] -> w133
      tunnel: [w240] -> _
      tunnel: w114 -> [w240]
      tunnel: w113 -> [w239]
      tunnel: w112 -> [w238]
      tunnel: [w237] -> w111
      frame #0 {
        n98 = call <vilib>:"High Resolution Relative Seconds.vi"() -> ("relative seconds"=w225:dbl)
      }
      frame #1 {
        n99 = call "HW_Stream_raw_data_enq.vi"("error in"=w230, "Queue in"=w231, "Data flow controls in"=w235, "VISA resource name in"=w232) -> ("error out"=w233:errorcluster, "Data flow controls out"=w236:T1, "VISA resource name out"=w234:refnum<visa-resource-name>)  [unwired: 4 in, 1 out]
      }
      frame #2 {
        n100 = call <vilib>:"High Resolution Relative Seconds.vi"() -> ("relative seconds"=w237:dbl)
      }
    }
    n101 = case "Inside this case structure TTL can be fired at the end of the recording" shown="True" w129 {
      selector: w129 -> [w265 w270]
      tunnel: w133 -> [w266 w274]
      tunnel: [w267 w276] -> w131
      tunnel: w132 -> [w267 w275]
      tunnel: [w266 w273] -> w130
      tunnel: w123 -> [_ w272]
      tunnel: [w265 w270] -> w124
      tunnel: w122 -> [_ w269]
      tunnel: w122 -> [_ w268]
      frame False {
      }
      frame True {
        n102 = First Call?() -> (First Call?: T/F=w271:bool)
        n103 = case shown="True" w271 {
          tunnel: [w278 w290] -> w276
          tunnel: w275 -> [w278 w289]
          tunnel: w274 -> [w277 w288]
          tunnel: [w277 w287] -> w273
          tunnel: w272 -> [_ w286]
          tunnel: w269 -> [_ w279]
          tunnel: w268 -> [_ w280]
          frame False {
          }
          frame True {
            n104 = flat-sequence {
              tunnel: w286 -> [w302]
              tunnel: w288 -> [w303]
              tunnel: w289 -> [w301]
              tunnel: [w301] -> w283
              tunnel: [w303] -> w282
              tunnel: [w302] -> w281
              tunnel: w280 -> [w291]
              tunnel: [w311] -> w285
              tunnel: [w310] -> w284
              tunnel: w283 -> [w308]
              tunnel: w282 -> [w305]
              tunnel: w281 -> [w306]
              tunnel: w279 -> [w304]
              tunnel: [w323] -> w287
              tunnel: [w322] -> w290
              tunnel: w285 -> [w322]
              tunnel: w284 -> [w323]
              frame #0 {
                n105 = Number To Boolean Array(number=w291) -> (Boolean array=w297:bool[])
                n106 = Index Array(array=w297, index=3) -> (element=w295:bool)
                n107 = Index Array(array=w297, index=2) -> (element=w294:bool)
                n108 = Index Array(array=w297, index=1) -> (element=w293:bool)
                n109 = Index Array(array=w297, index=0) -> (element=w292:bool)
                n110 = property on="TTL IO 4 (recording)" class="Bool (strict)"("Value"=w295) -> ()  [unwired: 2 in, 2 out]
                n111 = property on="TTL IO 3 (recording)" class="Bool (strict)"("Value"=w294) -> ()  [unwired: 2 in, 2 out]
                n112 = property on="TTL IO 2 (recording)" class="Bool (strict)"("Value"=w293) -> ()  [unwired: 2 in, 2 out]
                n113 = property on="TTL IO 1 (recording)" class="Bool (strict)"("Value"=w292) -> ()  [unwired: 2 in, 2 out]
              }
              frame #1 {
                n114 = call "SW_Fire_TTL_at_stop_universal.vi"("TTL port(s) config to fire"=w304, "TTL pulse length, ms"=200.0, "error in (no error)"=w308, "Serial Port In"=w305, "Close VISA (T)"=FALSE, "Start/stop signaling (F)"=w306) -> ("error out"=w311:errorcluster, "Serial Port Out"=w310:refnum<visa-resource-name>)  [unwired: 3 in, 1 out]
              }
              frame #2 {
                n115 = Number To Boolean Array(number=u32 0) -> (Boolean array=w315:bool[])
                n116 = Index Array(array=w315, index=2) -> (element=w318:bool)
                n117 = Index Array(array=w315, index=1) -> (element=w319:bool)
                n118 = Index Array(array=w315, index=0) -> (element=w320:bool)
                n119 = Index Array(array=w315, index=3) -> (element=w317:bool)
                n120 = property on="TTL IO 3 (recording)" class="Bool (strict)"("Value"=w318) -> ()  [unwired: 2 in, 2 out]
                n121 = property on="TTL IO 2 (recording)" class="Bool (strict)"("Value"=w319) -> ()  [unwired: 2 in, 2 out]
                n122 = property on="TTL IO 1 (recording)" class="Bool (strict)"("Value"=w320) -> ()  [unwired: 2 in, 2 out]
                n123 = property on="TTL IO 4 (recording)" class="Bool (strict)"("Value"=w317) -> ()  [unwired: 2 in, 2 out]
              }
            }
          }
        }
      }
    }
    n124 = case shown="True" w124 {
      tunnel: w130 -> [w247 w250]
      tunnel: w131 -> [w246 w251]
      tunnel: [w247 w248] -> w99
      tunnel: [w246 w249] -> w100
      frame False {
      }
      frame True {
        n125 = First Call?() -> (First Call?: T/F=w252:bool)
        n126 = case shown="True" w252 {
          tunnel: w251 -> [w253 w261]
          tunnel: w250 -> [w254 w260]
          tunnel: [w254 w256] -> w248
          tunnel: [w253 w258] -> w249
          frame False {
          }
          frame True {
            w255 = T15 16 items=["Flush Receive Buffer"=16, "Write Transmit Buffer to Device"=32, "Flush Receive Buffer (No I/O)"=64, "Flush Transmit Buffer"=128] ("Mask")
            n127 = Concatenate Strings("SYNC=0" ("string"), "\r") -> (w264:string)
            n128 = VISA Write(VISA resource name=w260, write buffer=w264, error in (no error)=w261) -> (VISA resource name out=w257:refnum<visa-resource-name>, error out=w259:errorcluster)  [unwired: 1 out]
            n129 = VISA Flush I/O Buffer(VISA resource name=w257, mask (16)=w255, error in (no error)=w259) -> (VISA resource name out=w256:refnum<visa-resource-name>, error out=w258:errorcluster)
          }
        }
      }
    }
    n130 = case shown="True" w102 {
      tunnel: w101 -> [_ w136]
      tunnel: w100 -> [_ w135]
      tunnel: w99 -> [_ w134]
      frame False {
      }
      frame True {
        n131 = call "HW_Stop_acq_and_close_VISA.vi"("error in"=w135, "Data flow controls in"=w136, "VISA resource name in"=w134) -> ()  [unwired: 2 out]
      }
    }
    n132 = node-c288(w100) -> ()  [unwired: 1 out]
  }
  n133 = case shown="False" w8 {
    frame True {
      w327 = T10."Enabled" ("Disabled")
      n134 = global read "SW_Globals.vi" "IO inversion config."() -> (w324:u16)
      n135 = global read "SW_Globals.vi" "VISA resource name"() -> (w326:refnum<visa-resource-name>)
      n136 = global read "SW_Globals.vi" "IO ports config"() -> (w325:bool[])
      n137 = call "HW_Set_IO_Dir_on_ECU.vi"("IO ports config"=w325, "VISA resource name"=w326, "IO inversion config."=w324) -> ()  [unwired: 1 in, 2 out]
      n138 = property on="Cage diameter, mm" class="Ring (strict)"("DisabledEnum"=w327) -> ()  [unwired: 2 in, 2 out]
      n139 = property on="Set IO config" class="Bool"("DisabledEnum"=w327) -> ()  [unwired: 2 in, 2 out]
      n140 = property on="Starting angle MIDFIELD" class="DigNum (strict)"("DisabledEnum"=w327) -> ()  [unwired: 2 in, 2 out]
      n141 = property on="N segments MIDFIELD" class="DigNum (strict)"("DisabledEnum"=w327) -> ()  [unwired: 2 in, 2 out]
      n142 = property on="Radius, mm MIDFIELD" class="DigNum (strict)"("DisabledEnum"=w327) -> ()  [unwired: 2 in, 2 out]
      n143 = property on="Starting angle BORDER" class="DigNum (strict)"("DisabledEnum"=w327) -> ()  [unwired: 2 in, 2 out]
      n144 = property on="N segments BORDER" class="DigNum (strict)"("DisabledEnum"=w327) -> ()  [unwired: 2 in, 2 out]
      n145 = property on="Radius, mm CENTER" class="DigNum (strict)"("DisabledEnum"=w327) -> ()  [unwired: 2 in, 2 out]
      n146 = property on="Start Tracking button" class="Bool"("DisabledEnum"=w327) -> ()  [unwired: 2 in, 2 out]
      n147 = property on="Reset stimuli" class="Bool (strict)"("DisabledEnum"=w327) -> ()  [unwired: 2 in, 2 out]
      n148 = property on="Reset regions" class="Bool (strict)"("DisabledEnum"=w327) -> ()  [unwired: 2 in, 2 out]
      n149 = property on="Zone-based stimulus setup" class="RadioBtnsControl (strict)"("DisabledEnum"=w327) -> ()  [unwired: 2 in, 2 out]
    }
    frame False {
      w328 = T10."Disabled and Grayed Out" ("Disabled")
      n150 = property on="Cage diameter, mm" class="Ring (strict)"("DisabledEnum"=w328) -> ()  [unwired: 2 in, 2 out]
      n151 = property on="Set IO config" class="Bool"("DisabledEnum"=w328) -> ()  [unwired: 2 in, 2 out]
      n152 = property on="Starting angle MIDFIELD" class="DigNum (strict)"("DisabledEnum"=w328) -> ()  [unwired: 2 in, 2 out]
      n153 = property on="N segments MIDFIELD" class="DigNum (strict)"("DisabledEnum"=w328) -> ()  [unwired: 2 in, 2 out]
      n154 = property on="Radius, mm MIDFIELD" class="DigNum (strict)"("DisabledEnum"=w328) -> ()  [unwired: 2 in, 2 out]
      n155 = property on="Starting angle BORDER" class="DigNum (strict)"("DisabledEnum"=w328) -> ()  [unwired: 2 in, 2 out]
      n156 = property on="N segments BORDER" class="DigNum (strict)"("DisabledEnum"=w328) -> ()  [unwired: 2 in, 2 out]
      n157 = property on="Radius, mm CENTER" class="DigNum (strict)"("DisabledEnum"=w328) -> ()  [unwired: 2 in, 2 out]
      n158 = property on="Start Tracking button" class="Bool"("DisabledEnum"=w328) -> ()  [unwired: 2 in, 2 out]
      n159 = property on="Reset stimuli" class="Bool (strict)"("DisabledEnum"=w328) -> ()  [unwired: 2 in, 2 out]
      n160 = property on="Reset regions" class="Bool (strict)"("DisabledEnum"=w328) -> ()  [unwired: 2 in, 2 out]
      n161 = property on="Zone-based stimulus setup" class="RadioBtnsControl (strict)"("DisabledEnum"=w328) -> ()  [unwired: 2 in, 2 out]
      n162 = property on="Set advanced stimulus" class="Bool (strict)"("DisabledEnum"=w328) -> ()  [unwired: 2 in, 2 out]
    }
  }
  n163 = node-c288(w31) -> ()  [unwired: 1 out]
  n164 = node-c288(w3, i64 139 ("Period"), 100 ("Priority")) -> (w29:T11)  [unwired: 1 in]
  n165 = timed-loop "This loop is used only for data loading purposes (that is why it is made relatively slow)" {
    tunnel: w6 -> [w333]
    timing: w29 -> [_]
    timing-out: [_] -> w28
    stop <- w330 stop-if-true
    n166 = node-c288() -> ()  [unwired: 1 in, 1 out]
    n167 = Unbundle By Name(w333) -> ("Has been recorded"=w332:refnum<notifier>, "Final CSV saved"=w339:refnum<notifier>, "Data loaded"=w338:refnum<notifier>, "Complete stop"=w331:refnum<notifier>)
    n168 = Get Notifier Status(notifier=w332) -> (current notification=w335:bool)  [unwired: 1 in, 4 out]
    n169 = Get Notifier Status(notifier=w339) -> (current notification=w337:bool)  [unwired: 1 in, 4 out]
    n170 = Get Notifier Status(notifier=w338) -> (current notification=w334:bool)  [unwired: 1 in, 4 out]
    n171 = Get Notifier Status(notifier=w331) -> (current notification=w330:bool)  [unwired: 1 in, 4 out]
    n172 = Not(x=w334) -> (.not. x?=w336:bool)
    n173 = Compound Arithmetic op=AND(w335, w337, w336) -> (w329:bool)
    n174 = case shown="True" w329 {
      tunnel: w333 -> [_ w445]
      frame False {
      }
      frame True {
        w356 = FALSE
        w362 = T10."Disabled and Grayed Out" ("Disabled")
        w385 = 7
        # "Y coord"
        # "X coord"
        # "Background color"
        # "Histogram"
        # "Diagram with zones"
        # "Diagram no zones"
        n175 = property on="Show heatmap (analysis)" class="Bool (strict)"("DisabledEnum"=w362, "Val(Sgnl)"=w356) -> (error out=w361:errorcluster)  [unwired: 2 in, 1 out]
        n176 = property on="Show full track (analysis)" class="Bool (strict)"("DisabledEnum"=w362, "Val(Sgnl)"=w356) -> (error out=w360:errorcluster)  [unwired: 2 in, 1 out]
        n177 = property on="Zones (analysis)" class="Bool (strict)"("DisabledEnum"=w362, "Val(Sgnl)"=w356) -> (error out=w359:errorcluster)  [unwired: 2 in, 1 out]
        n178 = property on="Play/Pause" class="Bool (strict)"("DisabledEnum"=w362) -> (error out=w358:errorcluster)  [unwired: 2 in, 1 out]
        n179 = Merge Errors(w361, w360, w359, w358) -> (w357:errorcluster)
        n180 = property on="Data loading progress" class="Slide (strict)"(error in=w357, "DisabledEnum"=T10."Disabled" ("Disabled"), "Value"=0.0 ("Data loading progress")) -> (error out=w443:errorcluster)  [unwired: 1 in, 1 out]
        n181 = control-ref of="Data loading progress"() -> (w447:refnum<vi>)
        n182 = global read "SW_Globals.vi" "Cluster of paths"() -> (w446:T19)
        n183 = property on="Play/Pause" class="Bool (strict)"(error in=w443, "DisabledEnum"=T10."Disabled and Grayed Out" ("Disabled")) -> (error out=w441:errorcluster)  [unwired: 1 in, 1 out]
        n184 = call "SW_Load_data_for_Analysis.vi"("Data flow controls"=w445, "Cluster of paths input"=w446, "Progress bar reference"=w447, "error in (no error)"=w441) -> ("Loaded data"=w355:T20, "error out"=w400:errorcluster)  [unwired: 2 in, 12 out]
        n185 = Unbundle By Name(w355) -> ("Zones preference array (loaded)"=→"Zones preference array (loaded)":dbl[][], "TTL inputs"=→"TTL inputs":u8[], "TTL outputs"=→"TTL outputs":u8[], "Stimulus presets array (loaded)"=w342:T6, "Absolute timestamp"=→"Absolute timestamp (rec)":dbl[], "Relative timestamp"=w349:dbl[], "X coord"=w348:dbl[], "Y coord"=w347:dbl[], "alpha rot. angle"=→"alpha rot. angle":dbl[], "Current zone"=→"Current zone":dbl[], "Acquisition settings cluster out"=w345:T21, "Data column names"=→"Data column names":string[])
        "Y coord" <- w347
        "X coord" <- w348
        "Relative timestamp (rec)" <- w349
        n186 = property on="Data loading progress" class="Slide (strict)"(error in=w400, "DisabledEnum"=T10."Disabled and Grayed Out" ("Disabled")) -> (error out=w366:errorcluster)  [unwired: 1 in, 1 out]
        n187 = for {
          tunnel: w342 -> [w505] mode=indexing
          tunnel: [w503] -> w401 mode=indexing if=w502
          i -> [w504]
          n188 = Unbundle By Name(w505) -> ("Stim. has been set"=w502:bool)
          n189 = To Unsigned Byte Integer(number=w504) -> (unsigned 8bit integer=w503:u8)
        }
        n190 = Unbundle By Name(w345) -> ("Vertical offset"=w343:dbl, "Mouse snout orientation swap?"=→"Mouse snout orientation swap (analysis)":bool, "Cage diameter, mm"=w411:u32, "Amount of border segments"=w410:u32, "Border segments starting angle"=w409:i32, "Amount of midfield segments"=w408:u32, "Midfield segments starting angle"=w407:i32, "Midfield segments outer radius, mm"=w405:u32, "Center segment outer radius, mm"=w404:u32, "Researcher name"=w431:string)
        "Vertical offset (analysis)" <- w343
        n191 = Array Max & Min(array=w349) -> (max value=w438:dbl, max index (indices)=→"Index of the last recorded timepoint":i32, min value=w437:dbl)  [unwired: 1 out]
        n192 = property on="Vertical offset" class="DigNum (strict)"("Value"=w343) -> ()  [unwired: 2 in, 2 out]
        n193 = Concatenate Strings("Recorded by " ("string"), w431) -> (→"Recorded by":string)
        n194 = Compound Arithmetic op=ADD(w410, w408, u32 1 ("value")) -> (w419:u32)
        n195 = Round To Nearest(number=w437) -> (nearest integer value=w435:dbl)
        n196 = Bundle By Name(cluster=T17 {"Amount of border segments"=8, "Border segments starting angle"=0, "Amount of midfield segments"=4, "Midfield segments starting angle"=0, "Midfield segments outer radius, mm"=60, "Amount of central segments"=1, "Center segment outer radius, mm"=30, "Diameter of the cage, mm"=180, "R-gap between segments, mm"=10} ("Input cluster of parameters"), "Diameter of the cage, mm"=w411, "Amount of border segments"=w410, "Border segments starting angle"=w409, "Amount of midfield segments"=w408, "Midfield segments starting angle"=w407, "Midfield segments outer radius, mm"=w405, "Center segment outer radius, mm"=w404) -> (w406:T17)
        n197 = global write "SW_Globals.vi" "Active segments amount"(w419) -> ()
        n198 = property on="Timeline" class="Slide (strict)"(error in=w366, "Scale.Maximum"=w438, "Scale.Minimum"=w435, "Value"=w435, "DisabledEnum"=T10."Disabled and Grayed Out" ("Disabled")) -> (error out=w432:errorcluster)  [unwired: 1 in, 1 out]
        n199 = Increment(x=w419) -> (x+1=w418:u32)
        n200 = flat-sequence "Full track preparation (array of clusters)" {
          tunnel: [w477] -> w373
          tunnel: w363 -> [w487]
          tunnel: w364 -> [w486]
          tunnel: w347 -> [w485]
          tunnel: w348 -> [w483]
          tunnel: [w481] -> w379
          tunnel: [w484] -> w378
          tunnel: w373 -> [w484]
          tunnel: [w501] -> w380
          tunnel: w379 -> [w501]
          tunnel: w378 -> [w500]
          tunnel: [w500] -> w376
          tunnel: [w499] -> w377
          frame #0 {
            n201 = Tick Count (ms)() -> (millisecond timer value=w477:u32)
          }
          frame #1 {
            n202 = Array Size(array=w483) -> (size(s)=w482:i32)
            n203 = for {
              N: w482 -> [_]
              tunnel: w483 -> [w498]
              tunnel: w485 -> [w497]
              tunnel: [w492] -> w479 mode=indexing
              tunnel: w486 -> [w495]
              tunnel: w487 -> [w491]
              i -> [w488]
              n204 = Index Array(array=w498, index=w488) -> (element=w489:dbl)
              n205 = Index Array(array=w497, index=w488) -> (element=w490:dbl)
              n206 = Multiply(x=w495, y=w489) -> (x*y=w494:dbl)
              n207 = Multiply(x=w495, y=w490) -> (x*y=w493:dbl)
              n208 = Bundle(w494, w493) -> (w496:cluster{dbl, dbl})  [unwired: 1 in]
              n209 = Add(x=w496, y=w491) -> (x+y=w492:cluster{dbl, dbl})
            }
            n210 = Delete From Array(array=w479, length=1, index=0) -> (array with subset deleted=w481:cluster{dbl, dbl}[])  [unwired: 1 out]
          }
          frame #2 {
            n211 = Tick Count (ms)() -> (millisecond timer value=w499:u32)
          }
        }
        n212 = property on="Diagram at analysis" class="Pict"(error in=w432) -> (error out=w403:errorcluster, "Bounds"=w413:T16)  [unwired: 1 in, 1 out]
        n213 = global write "SW_Globals.vi" "Regions to track"(w401) -> ()
        n214 = Bundle By Name(cluster=T18 {"Minimum"=0.0, "Maximum"=14.0, "Increment"=1.0, "Minor Increment"=1.0, "Start"=0.0} ("X Scale.Range"), "Maximum"=w418) -> (w417:T18)
        n215 = property on="Diagram at analysis" class="Pict"() -> ("Bounds"=w395:T16)  [unwired: 2 in, 2 out]
        n216 = control-ref of="Zones allocation array"() -> (w425:refnum<vi>)
        n217 = property on="Zones allocation (normalized) in analysis" class="WFGraph (strict)"("XScale.Range"=w417) -> ()  [unwired: 2 in, 2 out]
        n218 = call "SW_Generate_Segmented_Plot_v3.vi"("Draw Area Size"=w413, "Regions to mark set"=w401, "Input cluster of parameters"=w406, "Error In"=w403) -> ("Zones layout output"=w384:picture, "No zones image"=w382:picture, "Array of the pixel to color correspondences"=w415:u32[][], "Array of the segment to color correspondences"=w416:u32[][], "Cluster of image geometrical and scaling parameters"=w414:T22, "Error Out"=w402:errorcluster)  [unwired: 6 in]
        n219 = control-ref of="Diagram at analysis"() -> (w365:refnum<vi>)
        n220 = global write "SW_Globals.vi" "Diagram"(w384) -> ()
        n221 = global write "SW_Globals.vi" "Diagram no zones"(w382) -> ()
        n222 = Unbundle By Name(w414) -> ("Pixels per mm"=w364:dbl)
        n223 = global write "SW_Globals.vi" "Array of the pixel to color correspondences"(w415) -> ()
        n224 = global write "SW_Globals.vi" "Array of the segment to color correspondences"(w416) -> ()
        n225 = property class="Arr (strict)"(reference=w425, error in=w402) -> (reference out=w423:refnum<vi>, error out=w422:errorcluster, "Value"=w426:i32[])
        n226 = Quotient & Remainder(x=w395, y=T16 {"Width"=2, "Height"=2}) -> (floor(x/y)=w363:T16)  [unwired: 1 out]
        n227 = call <vilib>:"Picture to Pixmap.vi"("picture"=w382) -> ("image data"=w383:T23)  [unwired: 9 in, 1 out]
        n228 = call <vilib>:"Picture to Pixmap.vi"("picture"=w384) -> ("image data"=w399:T23)  [unwired: 9 in, 1 out]
        n229 = local write "Pixels per mm"(w364) -> ()
        n230 = call <vilib>:"Unflatten Pixmap.vi"("image data"=w383) -> ("24-bit pixmap"=w381:u32[][])  [unwired: 4 in, 6 out]
        n231 = call <vilib>:"Unflatten Pixmap.vi"("image data"=w399) -> ("24-bit pixmap"=w398:u32[][])  [unwired: 4 in, 6 out]
        n232 = Array Size(array=w426) -> (size(s)=w428:i32)
        n233 = call "SW_Gen_2D_Histogram.vi"("Picture reference in"=w365, "Pixels per mm"=w364, "Y coord array"=w347, "X coord array"=w348, "Bounds"=w363) -> ("24-bit pixmap"=w391:u32[][])  [unwired: 5 in, 1 out]
        n234 = Array Size(array=w391) -> (size(s)=w394:i32[])
        n235 = Initialize Array(0 ("element"), w428) -> (w424:i32[])
        n236 = property class="Arr (strict)"(reference=w423, error in=w422, "Value"=w424) -> ()  [unwired: 2 out]
        n237 = Index Array(array=w394, index=0) -> (element=w389:i32)
        n238 = Index Array(array=w394, index=1) -> (element=w387:i32)
        n239 = Subtract(x=w389, y=w385) -> (x-y=w388:i32)
        n240 = Subtract(x=w387, y=w385) -> (x-y=w386:i32)
        n241 = Index Array(array=w391, index (row)=w388, index (col)=w386) -> (element=w390:u32)
        n242 = Subtract(x=w377, y=w376) -> (x-y=→"Full track preparation":u32)
        n243 = flat-sequence {
          tunnel: w380 -> [w449]
          tunnel: w382 -> [w450]
          tunnel: w384 -> [w451]
          tunnel: [w451] -> w372
          tunnel: [w450] -> w371
          tunnel: [w449] -> w370
          tunnel: [w448] -> w368
          tunnel: w397 -> [w474]
          tunnel: w374 -> [w457]
          tunnel: w372 -> [w468]
          tunnel: w371 -> [w467]
          tunnel: w370 -> [w454]
          tunnel: [w476] -> w369
          frame #0 {
            n244 = Tick Count (ms)() -> (millisecond timer value=w448:u32)
          }
          frame #1 {
            w455 = T24 {"Width"=2, "Style"=enum."Solid"} ("pen")
            n245 = call <vilib>:"Flatten Pixmap.vi"("24-bit pixmap"=w457) -> ("image data"=w466:T23)  [unwired: 10 in]
            n246 = call <vilib>:"Flatten Pixmap.vi"("24-bit pixmap"=w474) -> ("image data"=w473:T23)  [unwired: 10 in]
            n247 = call <vilib>:"Draw Flattened Pixmap.vi"("image data"=w466) -> ("new picture"=w452:picture)  [unwired: 8 in]
            n248 = call <vilib>:"Draw Flattened Pixmap.vi"("image data"=w473) -> ("new picture"=w459:picture)  [unwired: 8 in]
            n249 = call "SW_Make_Track_overlay.vi"("Pen properties"=w455, "Full track array"=w454, "Full trace color"="Full trace color", "Picture in"=w468) -> ("Picture out"=w470:picture)  [unwired: 3 in]
            n250 = call "SW_Make_Track_overlay.vi"("Pen properties"=w455, "Full track array"=w454, "Full trace color"="Full trace color", "Picture in"=w452) -> ("Picture out"=w453:picture)  [unwired: 3 in]
            n251 = call "SW_Make_Track_overlay.vi"("Pen properties"=w455, "Full track array"=w454, "Full trace color"="Full trace color", "Picture in"=w459) -> ("Picture out"=w458:picture)  [unwired: 3 in]
            n252 = global write "SW_Globals.vi" "Density map no zones"(w452) -> ()
            n253 = call "SW_Make_Track_overlay.vi"("Pen properties"=w455, "Full track array"=w454, "Full trace color"="Full trace color", "Picture in"=w467) -> ("Picture out"=w471:picture)  [unwired: 3 in]
            n254 = global write "SW_Globals.vi" "Density map with zones"(w459) -> ()
            n255 = call <vilib>:"Picture to Pixmap.vi"("picture"=w470) -> ("image data"=w469:T23)  [unwired: 9 in, 1 out]
            n256 = call <vilib>:"Picture to Pixmap.vi"("picture"=w453) -> ("image data"=w463:T23)  [unwired: 9 in, 1 out]
            n257 = call <vilib>:"Picture to Pixmap.vi"("picture"=w458) -> ("image data"=w462:T23)  [unwired: 9 in, 1 out]
            n258 = call <vilib>:"Picture to Pixmap.vi"("picture"=w471) -> ("image data"=w472:T23)  [unwired: 9 in, 1 out]
            n259 = call <vilib>:"Draw Flattened Pixmap.vi"("image data"=w469) -> ("new picture"=w465:picture)  [unwired: 8 in]
            n260 = call <vilib>:"Draw Flattened Pixmap.vi"("image data"=w463) -> ("new picture"=w461:picture)  [unwired: 8 in]
            n261 = call <vilib>:"Draw Flattened Pixmap.vi"("image data"=w462) -> ("new picture"=w460:picture)  [unwired: 8 in]
            n262 = call <vilib>:"Draw Flattened Pixmap.vi"("image data"=w472) -> ("new picture"=w464:picture)  [unwired: 8 in]
            n263 = global write "SW_Globals.vi" "Full track with zones"(w465) -> ()
            n264 = global write "SW_Globals.vi" "Density map with no zones and with full track"(w461) -> ()
            n265 = global write "SW_Globals.vi" "Density map with zones and full track"(w460) -> ()
            n266 = global write "SW_Globals.vi" "Full track with no zones"(w464) -> ()
          }
          frame #2 {
            w475 = T10."Enabled" ("Disabled")
            n267 = property on="Show heatmap (analysis)" class="Bool (strict)"("DisabledEnum"=w475) -> ()  [unwired: 2 in, 2 out]
            n268 = property on="Show full track (analysis)" class="Bool (strict)"("DisabledEnum"=w475) -> ()  [unwired: 2 in, 2 out]
            n269 = property on="Zones (analysis)" class="Bool (strict)"("DisabledEnum"=w475) -> ()  [unwired: 2 in, 2 out]
            n270 = property on="Play/Pause" class="Bool (strict)"("DisabledEnum"=w475) -> ()  [unwired: 2 in, 2 out]
            n271 = Tick Count (ms)() -> (millisecond timer value=w476:u32)
          }
        }
        n272 = call "SW_Create_density_overlay.vi"("Background color"=w390, "Density histogram"=w391, "Diagram with zones"=w398, "Diagram no zones"=w381) -> ("Density map with zones"=w397:u32[][], "Density map no zones"=w374:u32[][])
        n273 = Subtract(x=w369, y=w368) -> (x-y=→"Full track plotting":u32)
      }
    }
    n274 = node-c288() -> ()  [unwired: 1 in, 1 out]
  }
  n275 = node-c288(w28) -> ()  [unwired: 1 out]
  n276 = node-c288(w3, i64 499 ("Period"), 800 ("Priority")) -> (w17:T11)
  n277 = timed-loop "Loop where temporary files are transferred to permanent location and data saved" {
    tunnel: w6 -> [w532]
    tunnel: [w517] -> w40
    timing: w17 -> [_]
    timing-out: [_] -> w16
    stop <- w518 stop-if-true
    n278 = node-c288() -> (→"Save iteration duration":i64)  [unwired: 1 in]
    n279 = flat-sequence {
      tunnel: w532 -> [w793]
      tunnel: [w793] -> w531
      tunnel: w531 -> [w794]
      tunnel: [w796] -> w529
      tunnel: [w795] -> w528
      tunnel: [w794] -> w530
      frame #0 {
        n280 = Wait (ms)(milliseconds to wait=u32 521) -> ()  [unwired: 1 out]
      }
      frame #1 {
        n281 = Unbundle By Name(w794) -> ("Path to the latest complete temp file"=w796:refnum<notifier>, "Temp file ready for processing"=w795:refnum<notifier>)
      }
    }
    n282 = Get Notifier Status(notifier=w528) -> (error out=w527:errorcluster)  [unwired: 1 in, 4 out]
    n283 = Get Notifier Status(notifier=w529, error in (no error)=w527) -> (current notification=w523:path)  [unwired: 4 out]
    n284 = feedback-in #1(w523) -> ()
    n285 = feedback #1(path "") -> (w525:path)
    n286 = local read "Starting angle MIDFIELD"() -> (w513:i16)
    n287 = local read "Starting angle BORDER"() -> (w515:i16)
    n288 = local read "N segments MIDFIELD"() -> (w514:u8)
    n289 = local read "Radius, mm MIDFIELD"() -> (w512:u16)
    n290 = local read "N segments BORDER"() -> (w516:u8)
    n291 = local read "Radius, mm CENTER"() -> (w510:u16)
    n292 = Not Equal?(x=w525, y=w523) -> (x != y?=w524:bool)
    n293 = Not Equal?(x=path "", y=w523) -> (x != y?=w522:bool)
    n294 = Bundle By Name(cluster=T25 {"N segments BORDER"=0, "Starting angle BORDER"=0, "N segments MIDFIELD"=0, "Starting angle MIDFIELD"=0, "Radius, mm MIDFIELD"=0, "Amount of central segments"=0, "Radius, mm CENTER"=0} ("output cluster 2"), "N segments BORDER"=w516, "Starting angle BORDER"=w515, "N segments MIDFIELD"=w514, "Starting angle MIDFIELD"=w513, "Radius, mm MIDFIELD"=w512, "Amount of central segments"=u8 1, "Radius, mm CENTER"=w510) -> (w509:T25)
    n295 = And(x=w522, y=w524) -> (x .and. y?=w519:bool)
    n296 = local read "Cage diameter, mm"() -> (w508:u16)
    n297 = global read "SW_Globals.vi" "Cluster of paths"() -> (w533:T19)
    n298 = case shown="True" w519 {
      tunnel: w533 -> [_ w557]
      tunnel: w530 -> [_ w556]
      tunnel: errorcluster {"status"=FALSE, "code"=0, "source"=""} ("error constant") -> [w538 w555]
      tunnel: w519 -> [_ w554]
      tunnel: w523 -> [_ w553]
      tunnel: [FALSE w544] -> w518
      tunnel: [w538 w545] -> w517
      tunnel: w509 -> [_ w548]
      tunnel: w508 -> [_ w547]
      frame False {
      }
      frame True {
        n299 = flat-sequence {
          tunnel: w553 -> [w627]
          tunnel: w554 -> [w626]
          tunnel: w557 -> [w612]
          tunnel: w555 -> [w625]
          tunnel: [w624] -> w561
          tunnel: w556 -> [w623]
          tunnel: [w623] -> w560
          tunnel: [w612] -> w551
          tunnel: w548 -> [w611]
          tunnel: w547 -> [w610]
          tunnel: w561 -> [w767]
          tunnel: [w767] -> w559
          tunnel: [w766] -> w558
          tunnel: w560 -> [w766]
          tunnel: w551 -> [w765]
          tunnel: [w765] -> w550
          tunnel: w559 -> [w775]
          tunnel: w558 -> [w774]
          tunnel: w550 -> [w771]
          tunnel: [w776] -> w542
          tunnel: [w779] -> w541
          tunnel: [w774] -> w540
          tunnel: [w771] -> w539
          tunnel: [w789] -> w549
          tunnel: [w790] -> w543
          tunnel: [w787] -> w546
          tunnel: [w791] -> w552
          tunnel: w542 -> [w791]
          tunnel: w541 -> [w787]
          tunnel: w540 -> [w790]
          tunnel: w539 -> [w789]
          frame #0 {
            n300 = Unbundle By Name(w612) -> ("Temporary csv output path"=w617:path, "Background picture output path"=w620:path, "Recording settings output path"=w619:path, "Final csv output path"=w618:path, "Path to the settings file"=w609:path)
            n301 = case shown="True" "Save files First Call" {
              selector: "Save files First Call" -> [w628 w641]
              tunnel: [w631 w744] -> w616
              tunnel: w627 -> [w631 w744]
              tunnel: w617 -> [w629 w731]
              tunnel: w620 -> [_ w729]
              tunnel: w619 -> [_ w727]
              tunnel: w618 -> [_ w699]
              tunnel: w625 -> [w630 w696]
              tunnel: [w630 w695] -> w615
              tunnel: [w629 w636] -> w613
              tunnel: w611 -> [_ w658]
              tunnel: w610 -> [_ w656]
              tunnel: w609 -> [_ w676]
              tunnel: [w628 w641] -> w608
              frame False {
              }
              frame True {
                w675 = "Vertical offset" ("key")
                w668 = "Mouse snout orientation swap?" ("key")
                w642 = "Recording settings" ("key")
                n302 = Unbundle By Name(w658) -> ("N segments BORDER"=w657:u8, "Starting angle BORDER"=w655:i16, "N segments MIDFIELD"=w654:u8, "Starting angle MIDFIELD"=w653:i16, "Radius, mm MIDFIELD"=w652:u16, "Radius, mm CENTER"=w650:u16)
                n303 = property on="Save files First Call" class="Bool (strict)"("Value"=FALSE ("Save files First Call")) -> ()  [unwired: 2 in, 2 out]
                n304 = Bundle By Name(cluster=T17 {"Amount of border segments"=8, "Border segments starting angle"=0, "Amount of midfield segments"=4, "Midfield segments starting angle"=0, "Midfield segments outer radius, mm"=60, "Amount of central segments"=1, "Center segment outer radius, mm"=30, "Diameter of the cage, mm"=180, "R-gap between segments, mm"=10} ("Input cluster of parameters"), "Diameter of the cage, mm"=w656, "Amount of border segments"=w657, "Border segments starting angle"=w655, "Amount of midfield segments"=w654, "Midfield segments starting angle"=w653, "Midfield segments outer radius, mm"=w652, "Center segment outer radius, mm"=w650) -> (w651:T17)
                n305 = global read "SW_Globals.vi" "Regions to track"() -> (w661:u8[])
                n306 = Build Array("X1_raw", "Y1_raw", "X2_raw", "Y2_raw", "Absolute_timestamp", "Relative_timestamp", "R", "phi", "alpha", "X", "Y", "w", "Current_zone", "Zones_preference", "TTL_inputs", "TTL_outputs", "Speed_mm_per_s", "Frame_OK") -> (w632:string[])
                n307 = call-poly <vilib>:"Write Delimited Spreadsheet.vi"("file path (dialog if empty)"=w731, "1D data"=w632, "append to file? (new file:F)"=FALSE, "error in (no error)"=w696) -> ("new file path (Not A Path if cancelled)"=w637:path, "error out"=w634:errorcluster)  [unwired: 10 in]
                n308 = Set Permissions(7:i16 384 ("permissions"), 8:w634, 11:w637) -> (0:w633:errorcluster, 3:w636:path)  [unwired: 2 in]
                n309 = call "SW_Generate_Segmented_Plot_v3.vi"("Draw Area Size"=cluster{"Width":dbl, "Height":dbl} {"Width"=1200.0, "Height"=1200.0}, "Regions to mark set"=w661, "Input cluster of parameters"=w651, "Error In"=w633) -> ("Zones layout output"=w662:picture, "Error Out"=w663:errorcluster)  [unwired: 6 in, 4 out]
                n310 = call <vilib>:"Picture to Pixmap.vi"("picture"=w662) -> ("image data"=w728:T23)  [unwired: 9 in, 1 out]
                n311 = local read "Current User"() -> (w702:string)
                n312 = call <vilib>:"Write PNG File.vi"("error in (no error)"=w663, "image data"=w728, "path to PNG file"=w729) -> ("error out"=w709:errorcluster)  [unwired: 7 in, 1 out]
                n313 = call <vilib>:"Open Config Data.vi"("error in (no error)"=w709, "configuration file path"=w727) -> ("refnum"=w707:T4)  [unwired: 7 in, 2 out]
                n314 = Strip Path(path=w699) -> (name=w698:string)  [unwired: 1 out]
                n315 = call <vilib>:"Write Key (String).vi"("section"=w642, "value"=w702, "key"="Researcher", "refnum"=w707) -> ("error out"=w704:errorcluster, "refnum out"=w706:T4)  [unwired: 5 in, 1 out]
                n316 = Unbundle By Name(w658) -> ("N segments MIDFIELD"=w694:u8, "N segments BORDER"=w693:u8, "Radius, mm CENTER"=w692:u16, "Radius, mm MIDFIELD"=w691:u16, "Starting angle MIDFIELD"=w690:i16, "Starting angle BORDER"=w689:i16)
                n317 = call <vilib>:"Write Key (String).vi"("section"=w642, "error in (no error)"=w704, "value"=w698, "key"="Track name", "refnum"=w706) -> ("error out"=w703:errorcluster, "refnum out"=w705:T4)  [unwired: 4 in, 1 out]
                n318 = call <vilib>:"Write Key (I32).vi"("section"=w642, "error in (no error)"=w703, "value"=w694, "key"="Amount of midfield segments", "refnum"=w705) -> ("error out"=w725:errorcluster, "refnum out"=w724:T4)  [unwired: 4 in, 1 out]
                n319 = call <vilib>:"Write Key (I32).vi"("section"=w642, "error in (no error)"=w725, "value"=w693, "key"="Amount of border segments", "refnum"=w724) -> ("error out"=w721:errorcluster, "refnum out"=w722:T4)  [unwired: 4 in, 1 out]
                n320 = call <vilib>:"Write Key (I32).vi"("section"=w642, "error in (no error)"=w721, "value"=w692, "key"="Center segment outer radius, mm", "refnum"=w722) -> ("error out"=w718:errorcluster, "refnum out"=w719:T4)  [unwired: 4 in, 1 out]
                n321 = call <vilib>:"Write Key (I32).vi"("section"=w642, "error in (no error)"=w718, "value"=w691, "key"="Midfield segments outer radius, mm", "refnum"=w719) -> ("error out"=w715:errorcluster, "refnum out"=w716:T4)  [unwired: 4 in, 1 out]
                n322 = call <vilib>:"Write Key (I32).vi"("section"=w642, "error in (no error)"=w715, "value"=w690, "key"="Midfield segments starting angle", "refnum"=w716) -> ("error out"=w713:errorcluster, "refnum out"=w712:T4)  [unwired: 4 in, 1 out]
                n323 = call <vilib>:"Write Key (I32).vi"("section"=w642, "error in (no error)"=w713, "value"=w689, "key"="Border segments starting angle", "refnum"=w712) -> ("error out"=w711:errorcluster, "refnum out"=w710:T4)  [unwired: 4 in, 1 out]
                n324 = local read "Current User"() -> (w667:string)
                n325 = property on="Vertical offset" class="DigNum (strict)"() -> ("Value"=w674:sgl)  [unwired: 2 in, 2 out]
                n326 = call <vilib>:"Write Key (I32).vi"("section"=w642, "error in (no error)"=w711, "value"=w656, "key"="Cage diameter, mm", "refnum"=w710) -> ("error out"=w681:errorcluster, "refnum out"=w678:T4)  [unwired: 4 in, 1 out]
                n327 = call <vilib>:"Open Config Data.vi"("configuration file path"=w676) -> ("error out"=w673:errorcluster, "refnum"=w671:T4)  [unwired: 8 in, 1 out]
                n328 = property on="Bridge swap" class="Bool (strict)"() -> ("Value"=w669:bool)  [unwired: 2 in, 2 out]
                n329 = call <vilib>:"Write Key (Double).vi"("use system decimal point (T)"=FALSE, "section"=w667, "error in (no error)"=w673, "value"=w674, "key"=w675, "refnum"=w671) -> ("error out"=w670:errorcluster, "refnum out"=w666:T4)  [unwired: 3 in, 1 out]
                n330 = call <vilib>:"Write Key (Double).vi"("use system decimal point (T)"=FALSE, "section"=w642, "error in (no error)"=w681, "value"=w674, "key"=w675, "refnum"=w678) -> ("error out"=w680:errorcluster, "refnum out"=w679:T4)  [unwired: 3 in, 1 out]
                n331 = call <vilib>:"Write Key (Boolean).vi"("section"=w667, "error in (no error)"=w670, "value"=w669, "key"=w668, "refnum"=w666) -> ("error out"=w665:errorcluster, "refnum out"=w664:T4)  [unwired: 4 in, 1 out]
                n332 = call <vilib>:"Write Key (Boolean).vi"("section"=w642, "error in (no error)"=w680, "value"=w669, "key"=w668, "refnum"=w679) -> ("error out"=w685:errorcluster, "refnum out"=w686:T4)  [unwired: 4 in, 1 out]
                n333 = call <vilib>:"Close Config Data.vi"("error in (no error)"=w665, "refnum"=w664) -> ()  [unwired: 8 in, 2 out]
                n334 = property on="Stimulus presets" class="Arr (strict)"(error in=w685) -> (error out=w645:errorcluster, "Value"=w687:T6)  [unwired: 1 in, 1 out]
                n335 = for {
                  tunnel: w687 -> [w757] mode=indexing
                  tunnel: w686 -> [w750]
                  tunnel: [w754] -> w646
                  tunnel: w642 -> [w745]
                  i -> [w753]
                  n336 = Unbundle By Name(w757) -> ("Stim. has been set"=w755:bool)
                  n337 = Flatten To JSON(anything=w757) -> (JSON string=w756:string, 11:w747:errorcluster)  [unwired: 2 in]
                  n338 = Format Value(string ("")="Zone " ("string"), format string="%02d", value (0)=w753) -> (output string=w748:string)
                  n339 = call <vilib>:"Remove Key.vi"("section"=w745, "error in (no error)"=w747, "key"=w748, "refnum"=w750) -> ("error out"=w746:errorcluster, "refnum out"=w749:T4)  [unwired: 5 in, 1 out]
                  n340 = case shown="True" w755 {
                    tunnel: w756 -> [_ w764]
                    tunnel: w746 -> [_ w763]
                    tunnel: [w758 w762] -> w754
                    tunnel: w748 -> [_ w761]
                    tunnel: w749 -> [w758 w760]
                    tunnel: w745 -> [_ w759]
                    frame False {
                    }
                    frame True {
                      n341 = call <vilib>:"Write Key (String).vi"("section"=w759, "error in (no error)"=w763, "value"=w764, "key"=w761, "refnum"=w760) -> ("refnum out"=w762:T4)  [unwired: 4 in, 2 out]
                    }
                  }
                }
                n342 = property on="IO parameters string" class="Str"(error in=w645) -> (error out=w647:errorcluster, "Value"=w648:string)  [unwired: 1 in, 1 out]
                n343 = call <vilib>:"Write Key (String).vi"("section"=w642, "error in (no error)"=w647, "value"=w648, "key"="IO ports configuration", "refnum"=w646) -> ("error out"=w644:errorcluster, "refnum out"=w643:T4)  [unwired: 4 in, 1 out]
                n344 = call <vilib>:"Close Config Data.vi"("error in (no error)"=w644, "refnum"=w643) -> ("error out"=w695:errorcluster)  [unwired: 8 in, 1 out]
              }
            }
            n345 = call-poly <vilib>:"Read Delimited Spreadsheet.vi"("file path (dialog if empty)"=w616, "error in (no error)"=w615) -> ("all rows"=w607:string[][], "error out"=w614:errorcluster)  [unwired: 8 in, 4 out]
            n346 = Array Subset(array=w607, index (row)=1 ("index")) -> (w606:string[][])  [unwired: 3 in]
            n347 = Select(t=w606, s=w608, f=w607) -> (s? t:f=w603:string[][])
            n348 = call-poly <vilib>:"Write Delimited Spreadsheet.vi"("file path (dialog if empty)"=w613, "format (%s)"="%s", "2D data"=w603, "append to file? (new file:F)"=TRUE, "error in (no error)"=w614) -> ("error out"=w624:errorcluster)  [unwired: 9 in, 1 out]
            "Path to the latest saved temp file" <- w627
            "Temp file ready" <- w626
          }
          frame #1 {
            n349 = Wait (ms)(milliseconds to wait=u32 257 ("millisecond multiple")) -> ()  [unwired: 1 out]
          }
          frame #2 {
            n350 = Unbundle By Name(w774) -> ("Recording now"=w770:refnum<notifier>, "Has been recorded"=w769:refnum<notifier>, "Path to the latest complete temp file"=w785:refnum<notifier>, "Temp file ready for processing"=w786:refnum<notifier>)
            n351 = Send Notification(notification=FALSE, notifier=w786, error in (no error)=w775) -> (error out=w784:errorcluster)  [unwired: 1 out]
            n352 = Get Notifier Status(notifier=w785, error in (no error)=w784) -> (current notification=w772:path, error out=w783:errorcluster)  [unwired: 3 out]
            n353 = Delete(path (use dialog)=w772, error in=w783) -> (error out=w778:errorcluster)  [unwired: 3 in, 2 out]
            n354 = Get Notifier Status(notifier=w769, error in (no error)=w778) -> (current notification=w780:bool, error out=w777:errorcluster)  [unwired: 3 out]
            n355 = Get Notifier Status(notifier=w770, error in (no error)=w777) -> (current notification=w782:bool, error out=w776:errorcluster)  [unwired: 3 out]
            n356 = Not(x=w782) -> (.not. x?=w781:bool)
            n357 = And(x=w781, y=w780) -> (x .and. y?=w779:bool)
          }
          frame #3 {
            n358 = Wait (ms)(milliseconds to wait=u32 257 ("millisecond multiple")) -> ()  [unwired: 1 out]
          }
        }
        n359 = case "Case Here data saving will be finalized" shown="True" w546 {
          selector: w546 -> [w563 w576]
          tunnel: w552 -> [w562 w565]
          tunnel: [w563 w576] -> w544
          tunnel: w549 -> [_ w577]
          tunnel: [w562 w573] -> w545
          tunnel: w543 -> [_ w570]
          frame False {
          }
          frame True {
            n360 = Unbundle By Name(w577) -> ("Final csv output path"=w571:path, "Temporary csv output path"=w567:path)
            n361 = Set Permissions(7:i16 438 ("permissions"), 8:w565, 11:w567) -> (0:w564:errorcluster, 3:w568:path)  [unwired: 2 in]
            n362 = while {
              tunnel: w568 -> [w586]
              tunnel: w571 -> [w584]
              tunnel: w564 -> [w588]
              tunnel: [w587] -> w574
              tunnel: w570 -> [w585]
              tunnel: [w585] -> w569
              i -> [w581]
              stop <- w578 stop-if-true
              n363 = flat-sequence {
                tunnel: w588 -> [w592]
                tunnel: w586 -> [w590]
                tunnel: w584 -> [w589]
                tunnel: [w591] -> w583
                tunnel: [w589] -> w580
                tunnel: w583 -> [w595]
                tunnel: [w595] -> w582
                tunnel: w580 -> [w593]
                tunnel: [w593] -> w579
                tunnel: [w602] -> w587
                tunnel: w582 -> [w602]
                tunnel: w581 -> [w598]
                tunnel: w579 -> [w597]
                tunnel: [w596] -> w578
                frame #0 {
                  n364 = Move(source path=w590, error in=w592, 10:w589) -> (error out=w591:errorcluster)  [unwired: 2 in, 2 out]
                }
                frame #1 {
                  n365 = Wait (ms)(milliseconds to wait=u32 500) -> ()  [unwired: 1 out]
                }
                frame #2 {
                  n366 = call <vilib>:"Check if File or Folder Exists.vi"("path"=w597) -> ("file or folder exists?"=w601:bool)  [unwired: 8 in, 2 out]
                  n367 = Greater?(x=w598, y=9) -> (0:w600:bool)
                  n368 = Or(x=w600, y=w601) -> (x .or. y?=w596:bool)
                }
              }
            }
            n369 = Unbundle By Name(w569) -> ("Final CSV saved"=w575:refnum<notifier>)
            n370 = Send Notification(notification=TRUE, notifier=w575, error in (no error)=w574) -> (error out=w573:errorcluster)  [unwired: 1 out]
          }
        }
      }
    }
    n371 = node-c288() -> ()  [unwired: 1 in, 1 out]
  }
  "error out" <- w40
  n372 = flat-sequence "Things to run at the very beginning of the program" {
    tunnel: [w887] -> w43
    tunnel: [w899] -> w4
    tunnel: [w801] -> w3
    frame #0 {
      w848 = T9 [{"Numeric Control"=9868950, "Numeric Control"=15790320}, {"Numeric Control"=8388608, "Numeric Control"=8388608}, {"Numeric Control"=4934475, "Numeric Control"=7895160}, {"Numeric Control"=994319, "Numeric Control"=1657881}]  # TTL IO In colors
      w849 = T9 [{"Numeric Control"=9868950, "Numeric Control"=15790320}, {"Numeric Control"=1988894, "Numeric Control"=3381555}, {"Numeric Control"=4934475, "Numeric Control"=7895160}, {"Numeric Control"=994319, "Numeric Control"=1657881}]  # TTL IO Out colors
      w874 = T10."Enabled" ("Disabled")
      w908 = FALSE ("Recording has been started with TTL")
      w925 = "Researcher"
      w946 = enum32{"Settings", "Recording", "Analysis"}."Settings" ("Main tab control")
      w953 = enum32{"Settings", "Recording", "Analysis"}."Analysis" ("Main tab control")
      w961 = enum32{"Settings", "Recording", "Analysis"}."Recording" ("Main tab control")
      n373 = call-poly <vilib>:"Create Timing Source.vi"("error in (no error)"="error in (no error)", "name (in)"="1 kHz") -> ("error out"=w800:errorcluster, "name (out)"=w801:string)  [unwired: 8 in]
      n374 = property on="Jump to Analysis" class="Bool (strict)"(error in=w800, "Value"=FALSE ("Jump to Analysis")) -> (error out=w842:errorcluster)  [unwired: 1 in, 1 out]
      n375 = property on="IO parameters string" class="Str"(error in=w842, "Value"="[12,1,1,0,0,0]" ("IO parameters string")) -> (error out=w872:errorcluster)  [unwired: 1 in, 1 out]
      n376 = property on="Pane" class="Pane"(error in=w872) -> (error out=w883:errorcluster, "Decos[]"=w884:refnum<vi>[])  [unwired: 1 in, 1 out]
      n377 = for {
        tunnel: w884 -> [w981] mode=indexing
        tunnel: w883 -> [w979]
        tunnel: [w978] -> w876
        n378 = property class="Decor"(reference=w981, error in=w979, "Visible"=FALSE) -> (error out=w978:errorcluster)  [unwired: 1 out]
      }
      n379 = property on="Vertical offset" class="DigNum (strict)"(error in=w876, "DisabledEnum"=w874) -> (error out=w875:errorcluster)  [unwired: 1 in, 1 out]
      n380 = property on="Back to Settings" class="Bool (strict)"(error in=w875, "DisabledEnum"=w874, "Visible"=FALSE) -> (error out=w886:errorcluster)  [unwired: 1 in, 1 out]
      n381 = call "FL_Gen_Bins_for_RunTimes.vi"("Min time, s"=0.5 ("Min run, m"), "N bins"=u16 11, "Max time, s"=10.0 ("Max run, m")) -> ("Bins array"=w809:dbl[])  [unwired: 1 in]
      n382 = Array Size(array=w809) -> (size(s)=w811:i32)
      n383 = Initialize Array(u32 0 ("element"), w811) -> (w813:u32[])
      n384 = global write "SW_Globals.vi" "Run Times distribution array"(w813) -> ()
      n385 = call "FL_Gen_Bins_for_RunLengths.vi"("Min run, m"=0.2, "N bins"=u16 11, "Max run, m"=2.0) -> ("Bins array"=w817:dbl[])  [unwired: 1 in]
      n386 = Array Size(array=w817) -> (size(s)=w819:i32)
      n387 = Initialize Array(u32 0 ("element"), w819) -> (w816:u32[])
      n388 = global write "SW_Globals.vi" "Run Lengts distribution array"(w816) -> ()
      n389 = global write "SW_Globals.vi" "Run Times bins array"(w809) -> ()
      n390 = global write "SW_Globals.vi" "Run Lengths bins array"(w817) -> ()
      n391 = property class="App"() -> ("App.Kind"=w923:T30)  [unwired: 2 in, 2 out]
      n392 = property on="Ready" class="Bool (strict)"(error in=w886, "Value"=FALSE ("Ready")) -> (error out=w841:errorcluster)  [unwired: 1 in, 1 out]
      n393 = global write "SW_Globals.vi" "Run time, s"(0.0 ("Run time, s")) -> ()
      n394 = case shown="\"invalid app kind\", Default" w923 {
        tunnel: [w1061 w1062] -> w916
        frame "invalid app kind", Default {
          n395 = call <vilib>:"Application Directory.vi"() -> ("Application Directory"=w1061:path)
          "Application Directory" <- w1061
        }
        frame "Development System" {
          n396 = Current VI's Path() -> (path=w1063:path)
          n397 = Strip Path(path=w1063) -> (stripped path=w1062:path)  [unwired: 1 out]
        }
      }
      n398 = property on="TTL 1 counter" class="DigNum (strict)"("Value"=0 ("TTL 1 counter")) -> ()  [unwired: 2 in, 2 out]
      n399 = property on="TTL 2 counter" class="DigNum (strict)"("Value"=0 ("TTL 1 counter")) -> ()  [unwired: 2 in, 2 out]
      n400 = property on="TTL 3 counter" class="DigNum (strict)"("Value"=0 ("TTL 1 counter")) -> ()  [unwired: 2 in, 2 out]
      n401 = property on="TTL 4 counter" class="DigNum (strict)"("Value"=0 ("TTL 1 counter")) -> ()  [unwired: 2 in, 2 out]
      n402 = call "SW_Generate_Color_Ramp.vi"() -> ("Colors array"=w930:u32[])  [unwired: 2 in]
      n403 = property on="Zone-based stimulus setup" class="RadioBtnsControl (strict)"(error in=w841, "Value"=T27."No Selection" ("Stimulus")) -> (error out=w907:errorcluster)  [unwired: 1 in, 1 out]
      n404 = property on="Pane" class="Pane"("Origin"=T29 {"Horizontal"=0, "Vertical"=0}) -> ()  [unwired: 2 in, 2 out]
      n405 = global write "SW_Globals.vi" "Color ramp array"(w930) -> ()
      n406 = Build Path(base path=w916, name or relative path=path "Tracker_settings.tcf") -> (appended path=w910:path)
      "Path to the settings file" <- w910
      n407 = call "FL_Gen_Bins_for_Speed.vi"("Speed min"=8.0, "N bins"=u16 10, "Speed max"=300.0) -> ("Bins array"=w835:dbl[])  [unwired: 1 in]
      n408 = global read "SW_Globals.vi" "Cluster of paths"() -> (w911:T19)
      n409 = global write "SW_Globals.vi" "Recording start timestamp"(timestamp(0 s since 1904-01-01) ("Recording start timestamp")) -> ()
      n410 = call <vilib>:"Open Config Data.vi"("error in (no error)"=w907, "create file if necessary (T)"=FALSE, "configuration file path"=w910) -> ("error out"=w971:errorcluster, "refnum"=w970:T4)  [unwired: 6 in, 1 out]
      n411 = Array Size(array=w835) -> (size(s)=w834:i32)
      n412 = Initialize Array(u32 0 ("element"), w834) -> (w833:u32[])
      n413 = global write "SW_Globals.vi" "Speed bins array"(w835) -> ()
      n414 = Bundle By Name(cluster=w911, "Path to the settings file"=w910) -> (w909:T19)
      n415 = call <vilib>:"Get Key Names.vi"("section"="Users", "error in (no error)"=w971, "refnum"=w970) -> ("error out"=w967:errorcluster, "key names"=w963:string[], "refnum out"=w968:T4)  [unwired: 5 in, 1 out]
      n416 = property on="Type of histogram" class="DigNum (strict)"("Value"=u8 0 ("Type of histogram")) -> (error out=w815:errorcluster)  [unwired: 2 in, 1 out]
      n417 = property on="Histograms (normalized)" class="WFGraph (strict)"(error in=w815, "XScale.Ofst&Mult"=T26 {"Offset"=1.0, "Multiplier"=0.0} ("X Scale.Offset and Multiplier"), "XScale.ScaleFit"=u8 0 ("X Scale.Scale Fit"), "YScale.Mapping Mode"=u8 0 ("Y Scale.Mapping Mode"), "Plot.Fill/Pt. Color"=u32 15790320 ("Plot.Fill/Point Color"), "XScale.Range"=T18 {"Minimum"=0.0, "Maximum"=14.0, "Increment"=1.0, "Minor Increment"=1.0, "Start"=0.0} ("X Scale.Range")) -> ()  [unwired: 1 in, 2 out]
      n418 = global write "SW_Globals.vi" "Speed distribution array"(w833) -> ()
      n419 = call <vilib>:"Read Key (U32).vi"("section"="Defaults", "error in (no error)"=w967, "key"="Default User", "refnum"=w968) -> ("error out"=w942:errorcluster, "value"=w964:u32, "refnum out"=w941:T4)  [unwired: 4 in, 1 out]
      n420 = global write "SW_Globals.vi" "Cluster of paths"(w909) -> ()
      n421 = Index Array(array=w963, index=w964) -> ()  [unwired: 1 out]
      n422 = call "SW_Load_settings_to_main_tab.vi"("Refnum in"=w941, "User Name"=w925, "error in (no error)"=w942) -> ("VISA resource name"=w887:string, "Vertical offset"=w877:dbl, "Midfield segments outer radius, mm"=w931:i32, "Cage diameter, mm"=w937:i32, "Midfield segments starting angle"=w932:i32, "Border segments starting angle"=w933:i32, "Stimulus presets array"=w867:T31, "IO parameters cluster"=w859:T32, "Refnum out"=→"Settings file refnum out":T4, "Amount of midfield segments"=w939:i32, "Mouse snout orientation swap?"=w914:bool, "Amount of border segments"=w938:i32, "Center segment outer radius, mm"=w804:i32, "error out"=w863:errorcluster)  [unwired: 11 in]
      "Port" <- w887
      n423 = local write "Vertical offset"(w877) -> ()
      n424 = Unbundle By Name(w859) -> ("SYNC configuration"=w866:u16, "IO 1 configuration"=w806:u16, "IO 2 configuration"=w805:u16)
      n425 = local write "Radius, mm CENTER"(w804) -> ()
      n426 = local write "Radius, mm MIDFIELD"(w931) -> ()
      n427 = local write "Cage diameter, mm"(w937) -> ()
      n428 = local write "Starting angle BORDER"(w933) -> ()
      n429 = local write "N segments MIDFIELD"(w939) -> ()
      n430 = local write "N segments BORDER"(w938) -> ()
      n431 = local write "Starting angle MIDFIELD"(w932) -> ()
      n432 = call "SW_get_config_of_Zones_and_IO.vi"("Sync parameters cluster input"=w859) -> ("Zones out config bin"=w858:bool[], "Ports IO config (OUT is FALSE)"=w840:bool[], "IO inversion config."=w799:u16)  [unwired: 1 out]
      n433 = global write "SW_Globals.vi" "IO inversion config."(w799) -> ()
      n434 = property on="Bridge swap" class="Bool (strict)"(error in=w863, "DisabledEnum"=T10."Enabled" ("Disabled"), "Value"=w914) -> (error out=w913:errorcluster)  [unwired: 1 in, 1 out]
      n435 = call "SW_get_config_for_Start_Stop_pulses.vi"("Sync parameters cluster input"=w859) -> ("Start/Stop out pulses config"=→"Start/Stop out pulses config":u32, "Start/Stop in config"=→"Start/Stop in config":u32, "Start/Stop in config bin"=w861:bool[], "Start/Stop out pulses config bin"=w860:bool[])
      n436 = call "SW_Gen_Available_TTL_outputs_array.vi"("IO 2 configuration"=w805, "IO 1 configuration"=w806, "SYNC configuration"=w866) -> ("Available TTL outputs array"=w865:cluster{"String":string, "Value":i32}[])
      n437 = case "Let's set flag for alternative magnets orintation" shown="327" w804 {
        frame 180, Default {
          n438 = global write "SW_Globals.vi" "Alternative magnets orientation"(FALSE ("Alternative magnets orientation")) -> ()
        }
        frame 325 {
          n439 = global write "SW_Globals.vi" "Alternative magnets orientation"(FALSE ("Alternative magnets orientation")) -> ()
        }
        frame 327 {
          n440 = global write "SW_Globals.vi" "Alternative magnets orientation"(TRUE ("Alternative magnets orientation")) -> ()
        }
        frame 333 {
          n441 = global write "SW_Globals.vi" "Alternative magnets orientation"(FALSE ("Alternative magnets orientation")) -> ()
        }
      }
      n442 = global write "SW_Globals.vi" "IO parameters cluster"(w859) -> ()
      n443 = global write "SW_Globals.vi" "Start/Stop out pulses config bin"(w860) -> ()
      n444 = property on="TTL out" class="Ring (strict)"("StringsAndValues[]"=w865) -> ()  [unwired: 2 in, 2 out]
      n445 = global write "SW_Globals.vi" "Zones out config bin"(w858) -> ()
      n446 = global write "SW_Globals.vi" "Start/Stop in config bin"(w861) -> ()
      n447 = global write "SW_Globals.vi" "IO ports config"(w840) -> ()
      n448 = call "SW_get_IO_ports_representation.vi"("Sync parameters cluster input"=w859) -> ("IO status indicator"=→"IO status indicator":T5)
      n449 = property on="Main tab control" class="TabCtl (strict)"(error in=w913, "Value"=w961) -> (error out=w958:errorcluster, "Pages"=w962:refnum<vi>[])  [unwired: 1 in, 1 out]
      n450 = Index Array(array=w840, index=0) -> (element=w853:bool)
      n451 = Index Array(array=w840, index=1) -> (element=w852:bool)
      n452 = Index Array(array=w840, index=2) -> (element=w851:bool)
      n453 = Index Array(array=w840, index=3) -> (element=w850:bool)
      n454 = To Long Integer(number=w961) -> (32bit integer=w960:i32)
      n455 = Select(t=w848, s=w853, f=w849) -> (s? t:f=w847:T9)
      n456 = Select(t=w848, s=w852, f=w849) -> (s? t:f=w846:T9)
      n457 = Select(t=w848, s=w850, f=w849) -> (s? t:f=w844:T9)
      n458 = Index Array(array=w962, index=w960) -> (element=w959:refnum<vi>)
      n459 = Select(t=w848, s=w851, f=w849) -> (s? t:f=w845:T9)
      n460 = property class="Page"(reference=w959, error in=w958, "PageEnb"=T28."Page Disabled & Grayed" ("Page Enabled State")) -> (error out=w956:errorcluster)  [unwired: 1 out]
      n461 = property on="TTL IO 1 (recording)" class="Bool (strict)"("Colors [4]"=w847) -> ()  [unwired: 2 in, 2 out]
      n462 = property on="TTL IO 3 (recording)" class="Bool (strict)"("Colors [4]"=w845) -> ()  [unwired: 2 in, 2 out]
      n463 = property on="TTL IO 2 (recording)" class="Bool (strict)"("Colors [4]"=w846) -> ()  [unwired: 2 in, 2 out]
      n464 = property on="TTL IO 1 (analysis)" class="Bool"("Colors [4]"=w847) -> ()  [unwired: 2 in, 2 out]
      n465 = property on="TTL IO 4 (recording)" class="Bool (strict)"("Colors [4]"=w844) -> ()  [unwired: 2 in, 2 out]
      n466 = property on="Main tab control" class="TabCtl (strict)"(error in=w956, "Value"=w953) -> (error out=w955:errorcluster, "Pages"=w954:refnum<vi>[])  [unwired: 1 in, 1 out]
      n467 = To Long Integer(number=w953) -> (32bit integer=w952:i32)
      n468 = property on="TTL IO 3 (analysis)" class="Bool"("Colors [4]"=w845) -> ()  [unwired: 2 in, 2 out]
      n469 = property on="TTL IO 2 (analysis)" class="Bool"("Colors [4]"=w846) -> ()  [unwired: 2 in, 2 out]
      n470 = Index Array(array=w954, index=w952) -> (element=w951:refnum<vi>)
      n471 = property on="TTL IO 4 (analysis)" class="Bool"("Colors [4]"=w844) -> ()  [unwired: 2 in, 2 out]
      n472 = global write "SW_Globals.vi" "TTL recording start signal has been successfully reset"(w908) -> ()
      n473 = property class="Page"(reference=w951, error in=w955, "PageEnb"=T28."Page Disabled & Grayed" ("Page Enabled State")) -> (error out=w943:errorcluster)  [unwired: 1 out]
      n474 = global write "SW_Globals.vi" "Recording has been stopped with TTL"(w908) -> ()
      n475 = global write "SW_Globals.vi" "Recording has been started with TTL"(w908) -> ()
      n476 = property on="Main tab control" class="TabCtl (strict)"(error in=w943, "Value"=w946) -> (error out=w944:errorcluster, "Pages"=w945:refnum<vi>[])  [unwired: 1 in, 1 out]
      n477 = To Long Integer(number=w946) -> (32bit integer=w947:i32)
      n478 = for {
        N: 14 -> [_]
        tunnel: w867 -> [w985] mode=indexing
        tunnel: [w983] -> w888 mode=indexing if=w982
        i -> [w984]
        n479 = Unbundle By Name(w985) -> ("Stim. has been set"=w982:bool)
        n480 = case shown="6" w984 {
          tunnel: w982 -> [_ w986 w991 w996 w1001 w1006 w1011 w1016 w1021 w1026 w1032 w1036 w1042 w1047]
          frame 0, Default {
          }
          frame 1 {
            n481 = property on="Colors for Stim. setup" class="Arr (strict)"() -> ("Value"=w989:T2)  [unwired: 2 in, 2 out]
            n482 = Select(t=w989, s=w986, f=T9 [{"Numeric Control"=12369084, "Numeric Control"=12369084}, {"Numeric Control"=6603023, "Numeric Control"=6603023}, {"Numeric Control"=1976113, "Numeric Control"=1976113}, {"Numeric Control"=2575993, "Numeric Control"=2575993}] ("Colors [4] 2")) -> (s? t:f=w987:T9)
            n483 = property on="Zone 01" class="Bool (strict)"("Colors [4]"=w987, "Value"=FALSE) -> ()  [unwired: 2 in, 2 out]
          }
          frame 2 {
            n484 = property on="Colors for Stim. setup" class="Arr (strict)"() -> ("Value"=w994:T2)  [unwired: 2 in, 2 out]
            n485 = Select(t=w994, s=w991, f=T9 [{"Numeric Control"=12369084, "Numeric Control"=12369084}, {"Numeric Control"=6603023, "Numeric Control"=6603023}, {"Numeric Control"=1976113, "Numeric Control"=1976113}, {"Numeric Control"=2575993, "Numeric Control"=2575993}] ("Colors [4] 2")) -> (s? t:f=w992:T9)
            n486 = property on="Zone 02" class="Bool (strict)"("Colors [4]"=w992, "Value"=FALSE) -> ()  [unwired: 2 in, 2 out]
          }
          frame 3 {
            n487 = property on="Colors for Stim. setup" class="Arr (strict)"() -> ("Value"=w999:T2)  [unwired: 2 in, 2 out]
            n488 = Select(t=w999, s=w996, f=T9 [{"Numeric Control"=12369084, "Numeric Control"=12369084}, {"Numeric Control"=6603023, "Numeric Control"=6603023}, {"Numeric Control"=1976113, "Numeric Control"=1976113}, {"Numeric Control"=2575993, "Numeric Control"=2575993}] ("Colors [4] 2")) -> (s? t:f=w997:T9)
            n489 = property on="Zone 03" class="Bool (strict)"("Colors [4]"=w997, "Value"=FALSE) -> ()  [unwired: 2 in, 2 out]
          }
          frame 4 {
            n490 = property on="Colors for Stim. setup" class="Arr (strict)"() -> ("Value"=w1004:T2)  [unwired: 2 in, 2 out]
            n491 = Select(t=w1004, s=w1001, f=T9 [{"Numeric Control"=12369084, "Numeric Control"=12369084}, {"Numeric Control"=6603023, "Numeric Control"=6603023}, {"Numeric Control"=1976113, "Numeric Control"=1976113}, {"Numeric Control"=2575993, "Numeric Control"=2575993}] ("Colors [4] 2")) -> (s? t:f=w1002:T9)
            n492 = property on="Zone 04" class="Bool (strict)"("Colors [4]"=w1002, "Value"=FALSE) -> ()  [unwired: 2 in, 2 out]
          }
          frame 5 {
            n493 = property on="Colors for Stim. setup" class="Arr (strict)"() -> ("Value"=w1009:T2)  [unwired: 2 in, 2 out]
            n494 = Select(t=w1009, s=w1006, f=T9 [{"Numeric Control"=12369084, "Numeric Control"=12369084}, {"Numeric Control"=6603023, "Numeric Control"=6603023}, {"Numeric Control"=1976113, "Numeric Control"=1976113}, {"Numeric Control"=2575993, "Numeric Control"=2575993}] ("Colors [4] 2")) -> (s? t:f=w1007:T9)
            n495 = property on="Zone 05" class="Bool (strict)"("Colors [4]"=w1007, "Value"=FALSE) -> ()  [unwired: 2 in, 2 out]
          }
          frame 6 {
            n496 = property on="Colors for Stim. setup" class="Arr (strict)"() -> ("Value"=w1014:T2)  [unwired: 2 in, 2 out]
            n497 = Select(t=w1014, s=w1011, f=T9 [{"Numeric Control"=12369084, "Numeric Control"=12369084}, {"Numeric Control"=6603023, "Numeric Control"=6603023}, {"Numeric Control"=1976113, "Numeric Control"=1976113}, {"Numeric Control"=2575993, "Numeric Control"=2575993}] ("Colors [4] 2")) -> (s? t:f=w1012:T9)
            n498 = property on="Zone 06" class="Bool (strict)"("Colors [4]"=w1012, "Value"=FALSE) -> ()  [unwired: 2 in, 2 out]
          }
          frame 7 {
            n499 = property on="Colors for Stim. setup" class="Arr (strict)"() -> ("Value"=w1019:T2)  [unwired: 2 in, 2 out]
            n500 = Select(t=w1019, s=w1016, f=T9 [{"Numeric Control"=12369084, "Numeric Control"=12369084}, {"Numeric Control"=6603023, "Numeric Control"=6603023}, {"Numeric Control"=1976113, "Numeric Control"=1976113}, {"Numeric Control"=2575993, "Numeric Control"=2575993}] ("Colors [4] 2")) -> (s? t:f=w1017:T9)
            n501 = property on="Zone 07" class="Bool (strict)"("Colors [4]"=w1017, "Value"=FALSE) -> ()  [unwired: 2 in, 2 out]
          }
          frame 8 {
            n502 = property on="Colors for Stim. setup" class="Arr (strict)"() -> ("Value"=w1024:T2)  [unwired: 2 in, 2 out]
            n503 = Select(t=w1024, s=w1021, f=T9 [{"Numeric Control"=12369084, "Numeric Control"=12369084}, {"Numeric Control"=6603023, "Numeric Control"=6603023}, {"Numeric Control"=1976113, "Numeric Control"=1976113}, {"Numeric Control"=2575993, "Numeric Control"=2575993}] ("Colors [4] 2")) -> (s? t:f=w1022:T9)
            n504 = property on="Zone 08" class="Bool (strict)"("Colors [4]"=w1022, "Value"=FALSE) -> ()  [unwired: 2 in, 2 out]
          }
          frame 9 {
            n505 = property on="Colors for Stim. setup" class="Arr (strict)"() -> ("Value"=w1029:T2)  [unwired: 2 in, 2 out]
            n506 = Select(t=w1029, s=w1026, f=T9 [{"Numeric Control"=12369084, "Numeric Control"=12369084}, {"Numeric Control"=6603023, "Numeric Control"=6603023}, {"Numeric Control"=1976113, "Numeric Control"=1976113}, {"Numeric Control"=2575993, "Numeric Control"=2575993}] ("Colors [4] 2")) -> (s? t:f=w1027:T9)
            n507 = property on="Zone 09" class="Bool (strict)"("Colors [4]"=w1027, "Value"=FALSE) -> ()  [unwired: 2 in, 2 out]
          }
          frame 10 {
            n508 = property on="Colors for Stim. setup" class="Arr (strict)"() -> ("Value"=w1034:T2)  [unwired: 2 in, 2 out]
            n509 = Select(t=w1034, s=w1032, f=T9 [{"Numeric Control"=12369084, "Numeric Control"=12369084}, {"Numeric Control"=6603023, "Numeric Control"=6603023}, {"Numeric Control"=1976113, "Numeric Control"=1976113}, {"Numeric Control"=2575993, "Numeric Control"=2575993}] ("Colors [4] 2")) -> (s? t:f=w1031:T9)
            n510 = property on="Zone 10" class="Bool (strict)"("Colors [4]"=w1031, "Value"=FALSE) -> ()  [unwired: 2 in, 2 out]
          }
          frame 11 {
            n511 = property on="Colors for Stim. setup" class="Arr (strict)"() -> ("Value"=w1039:T2)  [unwired: 2 in, 2 out]
            n512 = Select(t=w1039, s=w1036, f=T9 [{"Numeric Control"=12369084, "Numeric Control"=12369084}, {"Numeric Control"=6603023, "Numeric Control"=6603023}, {"Numeric Control"=1976113, "Numeric Control"=1976113}, {"Numeric Control"=2575993, "Numeric Control"=2575993}] ("Colors [4] 2")) -> (s? t:f=w1038:T9)
            n513 = property on="Zone 11" class="Bool (strict)"("Colors [4]"=w1038, "Value"=FALSE) -> ()  [unwired: 2 in, 2 out]
          }
          frame 12 {
            n514 = property on="Colors for Stim. setup" class="Arr (strict)"() -> ("Value"=w1044:T2)  [unwired: 2 in, 2 out]
            n515 = Select(t=w1044, s=w1042, f=T9 [{"Numeric Control"=12369084, "Numeric Control"=12369084}, {"Numeric Control"=6603023, "Numeric Control"=6603023}, {"Numeric Control"=1976113, "Numeric Control"=1976113}, {"Numeric Control"=2575993, "Numeric Control"=2575993}] ("Colors [4] 2")) -> (s? t:f=w1041:T9)
            n516 = property on="Zone 12" class="Bool (strict)"("Colors [4]"=w1041, "Value"=FALSE) -> ()  [unwired: 2 in, 2 out]
          }
          frame 13 {
            n517 = property on="Colors for Stim. setup" class="Arr (strict)"() -> ("Value"=w1049:T2)  [unwired: 2 in, 2 out]
            n518 = Select(t=w1049, s=w1047, f=T9 [{"Numeric Control"=12369084, "Numeric Control"=12369084}, {"Numeric Control"=6603023, "Numeric Control"=6603023}, {"Numeric Control"=1976113, "Numeric Control"=1976113}, {"Numeric Control"=2575993, "Numeric Control"=2575993}] ("Colors [4] 2")) -> (s? t:f=w1046:T9)
            n519 = property on="Zone 13" class="Bool (strict)"("Colors [4]"=w1046, "Value"=FALSE) -> ()  [unwired: 2 in, 2 out]
          }
        }
        n520 = To Unsigned Byte Integer(number=w984) -> (unsigned 8bit integer=w983:u8)
      }
      n521 = global write "SW_Globals.vi" "Regions to track"(u8[] [] ("Regions to track")) -> ()
      n522 = Index Array(array=w945, index=w947) -> (element=w948:refnum<vi>)
      n523 = property class="Page"(reference=w948, error in=w944, "PageEnb"=T28."Page Enabled" ("Page Enabled State")) -> (error out=w936:errorcluster)  [unwired: 1 out]
      n524 = property on="Record/Stop" class="Bool (strict)"(error in=w936, "Value"=FALSE ("Record/Stop")) -> (error out=w935:errorcluster)  [unwired: 1 in, 1 out]
      n525 = Flatten To String(anything="Zones presence indicator") -> (data string=w920:string)  [unwired: 3 in, 2 out]
      n526 = String Length(string=w920) -> (length=w919:i32)
      n527 = global write "SW_Globals.vi" "Regions to track"(w888) -> ()
      n528 = property on="Play/Pause" class="Bool (strict)"(error in=w935, "Value"=FALSE ("Play/Pause")) -> (error out=w915:errorcluster)  [unwired: 1 in, 1 out]
      n529 = property on="Stimulus presets" class="Arr (strict)"("Value"=w867) -> (error out=w894:errorcluster)  [unwired: 2 in, 1 out]
      n530 = global write "SW_Globals.vi" "Stimulus presets"(w867) -> ()
      n531 = Initialize Array(FALSE, w919) -> (w823:bool[])
      "Zones presence array" <- w823
      n532 = Initialize Array(0, w919) -> (→"Zones allocation array":i32[])
      n533 = global read "SW_Globals.vi" "Run time pause, s"() -> (w797:dbl)
      n534 = property on="Stimulus presets" class="Arr (strict)"(error in=w894, "Index Values"=u32[] [0], "DisabledEnum"=T10."Disabled and Grayed Out" ("Disabled")) -> (error out=w871:errorcluster)  [unwired: 1 in, 1 out]
      n535 = property on="Record timestamp" class="DigNum (strict)"(error in=w915, "DisabledEnum"=T10."Disabled and Grayed Out" ("Disabled"), "Value"=0.0 ("Record timestamp")) -> (error out=w899:errorcluster)  [unwired: 1 in, 1 out]
      n536 = global write "SW_Globals.vi" "Zones presence array"(w823) -> ()
      n537 = property on="Pause, s" class="DigNum (strict)"("Value"=w797) -> ()  [unwired: 2 in, 2 out]
      n538 = property on="Data filtering" class="Ring (strict)"(error in=w871, "DisabledEnum"=T10."Enabled" ("Disabled")) -> (error out=w870:errorcluster)  [unwired: 1 in, 1 out]
      n539 = property on="N segments BORDER" class="DigNum (strict)"(error in=w870) -> (error out=w900:errorcluster, "Value"=w904:u8)  [unwired: 1 in, 1 out]
      n540 = property on="N segments MIDFIELD" class="DigNum (strict)"(error in=w900) -> (error out=w891:errorcluster, "Value"=w903:u8)  [unwired: 1 in, 1 out]
      n541 = property on="Zone-based stimulus setup" class="RadioBtnsControl (strict)"(error in=w891) -> (error out=w897:errorcluster, "Controls[]"=w902:refnum<vi>[])  [unwired: 1 in, 1 out]
      n542 = Compound Arithmetic op=ADD(w904, w903, u8 1 ("value")) -> (w901:u8)
      n543 = for {
        tunnel: w902 -> [w1060] mode=indexing
        tunnel: w901 -> [w1056]
        tunnel: w897 -> [w1051]
        tunnel: [w1053] -> w896
        i -> [w1052]
        n544 = Increment(x=w1052) -> (x+1=w1055:i32)
        n545 = Greater Or Equal?(x=w1056, y=w1055) -> (x >= y?=w1054:bool)
        n546 = Select(t=T10."Enabled" ("Disabled"), s=w1054, f=T10."Disabled and Grayed Out") -> (s? t:f=w1058:T10)
        n547 = property class="Ctl"(reference=w1060, error in=w1051, "DisabledEnum"=w1058) -> (error out=w1053:errorcluster)  [unwired: 1 out]
      }
      n548 = property on="Zone-based stimulus setup" class="RadioBtnsControl (strict)"(error in=w896, "Value"=T7."No Selection" ("Stim. setup")) -> (error out=w882:errorcluster)  [unwired: 1 in, 1 out]
      n549 = property on="Pane" class="Pane"(error in=w882) -> ("Decos[]"=w881:refnum<vi>[])  [unwired: 1 in, 2 out]
      n550 = Index Array(array=w881, index=2) -> (element=w879:refnum<vi>)
      n551 = property class="Decor"(reference=w879, "Visible"=TRUE) -> ()  [unwired: 1 in, 2 out]
      "Current User" <- w925
    }
  }
  n552 = node-c288(w3, w23, 900 ("Priority")) -> (w25:T11)
  n553 = timed-loop "This loop is all about temporary data processing and streaming to the interface part" {
    tunnel: w6 -> [w1079]
    tunnel: w5 -> [w1078]
    tunnel: [w1065] -> w41
    timing: w25 -> [_]
    timing-out: [_] -> w24
    tunnel: w23 -> [w1064]
    i -> [w1077]
    stop <- w1074 stop-if-true
    n554 = node-c288() -> ()  [unwired: 1 in, 1 out]
    n555 = Unbundle By Name(w1079) -> ("Complete stop"=w1080:refnum<notifier>, "Play/Pause status"=w1072:refnum<notifier>)
    n556 = flat-sequence {
      tunnel: w1079 -> [w1092]
      tunnel: w1064 -> [w1091]
      tunnel: w1077 -> [w1090]
      tunnel: w1075 -> [w1089]
      tunnel: w1073 -> [w1088]
      tunnel: [w1087] -> w1071
      tunnel: w1069 -> [w1086]
      tunnel: w1068 -> [w1085]
      tunnel: w1066 -> [w1084]
      tunnel: [w1083] -> w1065
      tunnel: w1072 -> [w1192]
      tunnel: w1071 -> [w1191]
      tunnel: [w1190] -> w1070
      frame #0 {
        n557 = case shown="\"Play\"" w1086 {
          tunnel: w1092 -> [_ w1170]
          tunnel: w1091 -> [_ w1169]
          tunnel: w1090 -> [_ w1168]
          tunnel: w1089 -> [_ w1167]
          tunnel: w1088 -> [_ w1164]
          tunnel: [w1093 w1149] -> w1087
          tunnel: w1085 -> [w1093 w1160]
          tunnel: w1084 -> [_ w1163]
          tunnel: [_ w1157] -> w1083
          frame "Pause", Default {
          }
          frame "Play" {
            w1101 = "." ("string")
            n558 = property on="Bridge swap" class="Bool (strict)"(error in=w1160) -> (error out=w1159:errorcluster, "Value"=w1158:bool)  [unwired: 1 in, 1 out]
            n559 = local read "Pixels per mm"() -> (w1161:dbl)
            n560 = property on="Diagram at recording" class="Pict"() -> ("Bounds"=w1162:T16)  [unwired: 2 in, 2 out]
            n561 = call "FL_Preprocess_and_save_incrementally_TDMS.vi"("Temporary file output path"=w1164, "Loop iteration"=w1168, "Mouse face dir. swap"=w1158, "Loop speed in ms"=w1169, "Save every N seconds"=u32 8, "error in (no error)"=w1159, "Filter type"="Data filtering", "Sensor read input"=w1167, "Offset"="Vertical offset", "Pixels per mm"=w1161, "Data flow controls in"=w1170, "Diagram at recording bounds"=w1162, "Sensor board size"=w1163) -> ("Eff. save interval"=→"Eff. save interval":sgl, "Latest sensor output (decoded)"=w1142:string[][], "Fire TTL"=w1094:bool, "TTL out N"=w1095:u8, "Current TTL status"=w1140:u8, "error out"=w1150:errorcluster)  [unwired: 1 in]
            "Current TTL status" <- w1140
            n562 = Index Array "TTL inputs"(array=w1142, index (col)=14) -> (element=w1143:string[])  [unwired: 1 in]
            n563 = property on="Start/Stop in config" class="DigNum (strict)"() -> ("Value"=w1146:u32)  [unwired: 2 in, 2 out]
            n564 = Decimal String To Number(string=w1143, default (0L)=u8 0 ("default (0 I32)")) -> (number=w1147:u8[])  [unwired: 1 in, 1 out]
            n565 = call <extravilib>:"Write.vi"("size (1)"=5, "element"=w1142) -> ("channel"=w1157:T33)  [unwired: 7 in, 2 out]
            n566 = Greater Than 0?(x=w1146) -> (x > 0?=w1148:bool)
            n567 = Search 1D Array(1D array=w1147, element=w1146) -> (index of element=w1145:i32)  [unwired: 1 in]
            n568 = Greater Or Equal To 0?(x=w1145) -> (x >= 0?=w1144:bool)
            n569 = And(x=w1148, y=w1144) -> (x .and. y?=w1153:bool)
            n570 = case shown="True" w1153 {
              tunnel: w1143 -> [_ w1189]
              frame False {
              }
              frame True {
                n571 = call "FL_Get_TTL_in_pulse_length.vi"("Latest sensor input (decoded)"=w1189) -> ("TTL pulse length, ms"=w1188:u32)
                n572 = global read "SW_Globals.vi" "TTL recording start signal has been successfully reset"() -> (w1179:bool)
                n573 = global read "SW_Globals.vi" "Recording has been started with TTL"() -> (w1182:bool)
                n574 = global read "SW_Globals.vi" "Recording has been stopped with TTL"() -> (w1176:bool)
                n575 = feedback #2(FALSE) -> (w1185:bool)
                n576 = Not(x=w1185) -> (.not. x?=w1186:bool)
                n577 = Greater Or Equal?(x=w1188, y=u32 225) -> (x >= y?=w1178:bool)
                "TTL is long enough" <- w1178
                n578 = And(x=w1186, y=w1178) -> (x .and. y?=w1183:bool)
                n579 = Not(x=w1178) -> (.not. x?=w1181:bool)
                n580 = And(x=w1182, y=w1181) -> (x .and. y?=w1180:bool)
                n581 = Or(x=w1183, y=w1182) -> (x .or. y?=w1175:bool)
                "Started" <- w1175
                n582 = feedback-in #2(w1175) -> ()
                n583 = Or(x=w1179, y=w1180) -> (x .or. y?=w1174:bool)
                "Reset starting pulse" <- w1174
                n584 = global write "SW_Globals.vi" "TTL recording start signal has been successfully reset"(w1174) -> ()
                n585 = global write "SW_Globals.vi" "Recording has been started with TTL"(w1175) -> ()
                n586 = Compound Arithmetic op=AND(w1174, w1175, w1178) -> (w1177:bool)
                n587 = Or(x=w1177, y=w1176) -> (x .or. y?=w1173:bool)
                "Stopped" <- w1173
                n588 = Not(x=w1173) -> (.not. x?=w1172:bool)
                n589 = global write "SW_Globals.vi" "Recording has been stopped with TTL"(w1173) -> ()
                n590 = Compound Arithmetic op=AND(w1175, w1174, w1172) -> (w1171:bool)
                "Record" <- w1171
                n591 = property on="Record/Stop" class="Bool (strict)"("Value"=w1171) -> ()  [unwired: 2 in, 2 out]
                n592 = property on="TTL REC" class="Bool (strict)"("Value"=w1171) -> ()  [unwired: 2 in, 2 out]
              }
            }
            n593 = Number To Boolean Array(number=w1140) -> (Boolean array=w1136:bool[])
            n594 = Index Array(array=w1136, index=0) -> (element=w1128:bool)
            "TTL IO 1 (recording)" <- w1128
            n595 = Index Array(array=w1136, index=1) -> (element=w1108:bool)
            "TTL IO 2 (recording)" <- w1108
            n596 = Index Array(array=w1136, index=2) -> (element=w1107:bool)
            "TTL IO 3 (recording)" <- w1107
            n597 = Index Array(array=w1136, index=3) -> (element=w1109:bool)
            "TTL IO 4 (recording)" <- w1109
            n598 = feedback #3(TRUE) -> (w1111:bool)
            n599 = feedback-in #3(w1109) -> ()
            n600 = feedback #4(TRUE) -> (w1121:bool)
            n601 = feedback-in #4(w1107) -> ()
            n602 = feedback #5(TRUE) -> (w1133:bool)
            n603 = feedback-in #5(w1128) -> ()
            n604 = feedback #6(TRUE) -> (w1122:bool)
            n605 = feedback-in #6(w1108) -> ()
            n606 = Not(x=w1111) -> (.not. x?=w1112:bool)
            n607 = Not(x=w1121) -> (.not. x?=w1119:bool)
            n608 = Not(x=w1133) -> (.not. x?=w1132:bool)
            n609 = Not(x=w1122) -> (.not. x?=w1124:bool)
            n610 = local read "TTL 4 counter"() -> (w1114:u32)
            n611 = And(x=w1112, y=w1109) -> (x .and. y?=w1113:bool)
            n612 = local read "TTL 3 counter"() -> (w1117:u32)
            n613 = local read "TTL 1 counter"() -> (w1130:u32)
            n614 = local read "TTL 2 counter"() -> (w1126:u32)
            n615 = And(x=w1119, y=w1107) -> (x .and. y?=w1118:bool)
            n616 = And(x=w1132, y=w1128) -> (x .and. y?=w1131:bool)
            n617 = And(x=w1124, y=w1108) -> (x .and. y?=w1125:bool)
            n618 = Increment(x=w1114) -> (x+1=w1115:u32)
            n619 = Increment(x=w1117) -> (x+1=w1116:u32)
            n620 = Increment(x=w1130) -> (x+1=w1129:u32)
            n621 = Select(t=w1115, s=w1113, f=w1114) -> (s? t:f=w1103:u32)
            "TTL 4 counter" <- w1103
            n622 = Increment(x=w1126) -> (x+1=w1127:u32)
            n623 = Select(t=w1116, s=w1118, f=w1117) -> (s? t:f=w1104:u32)
            "TTL 3 counter" <- w1104
            n624 = Select(t=w1129, s=w1131, f=w1130) -> (s? t:f=w1106:u32)
            "TTL 1 counter" <- w1106
            n625 = Select(t=w1127, s=w1125, f=w1126) -> (s? t:f=w1105:u32)
            "TTL 2 counter" <- w1105
            n626 = Number To Decimal String(number=w1106) -> (decimal integer string=w1102:string)  [unwired: 1 in]
            n627 = Number To Decimal String(number=w1105) -> (decimal integer string=w1100:string)  [unwired: 1 in]
            n628 = Number To Decimal String(number=w1104) -> (decimal integer string=w1099:string)  [unwired: 1 in]
            n629 = Number To Decimal String(number=w1103) -> (decimal integer string=w1098:string)  [unwired: 1 in]
            n630 = global read "SW_Globals.vi" "IO inversion config."() -> (w1096:u16)
            n631 = global read "SW_Globals.vi" "VISA resource name"() -> (w1151:refnum<visa-resource-name>)
            n632 = call "SW_Fire_TTL_during_the_acquisition_universal.vi"("IO inversion config."=w1096, "error in (no error)"=w1150, "Serial Port In"=w1151, "TTL port(s) config to fire"=w1095, "Fire TTL"=w1094) -> ("error out"=w1149:errorcluster)  [unwired: 6 in]
            n633 = Concatenate Strings(w1102, w1101, w1100, w1101, w1099, w1101, w1098) -> (→"IO pulses count":string)
          }
        }
      }
      frame #1 {
        n634 = Get Notifier Status(notifier=w1192, error in (no error)=w1191) -> (current notification=w1190:string)  [unwired: 4 out]
      }
    }
    n635 = Flush Queue(queue=w1078) -> (remaining elements=w1075:T34, error out=w1068:errorcluster)  [unwired: 1 in, 1 out]
    n636 = local read "Board size"() -> (w1066:string)
    n637 = global read "SW_Globals.vi" "Cluster of paths"() -> (w1076:T19)
    n638 = Get Notifier Status(notifier=w1080) -> (current notification=w1074:bool)  [unwired: 1 in, 4 out]
    n639 = Unbundle By Name(w1076) -> ("Temporary file output path"=w1073:path)
    n640 = feedback-in #7(w1070) -> ()
    n641 = feedback #7("Pause" ("String")) -> (w1069:string)
    n642 = node-c288() -> ()  [unwired: 1 in, 1 out]
  }
  n643 = node-c288(w24) -> ()  [unwired: 1 out]
  n644 = node-c288(w3, w10, 200 ("Priority")) -> (w13:T11)  [unwired: 1 in]
  n645 = node-c288(w16) -> ()  [unwired: 1 out]
  n646 = Tick Count (ms)() -> (millisecond timer value=w42:u32)
  n647 = timed-loop {
    tunnel: w5 -> [w1207]
    tunnel: w6 -> [w1205]
    tunnel: w6 -> [w1204]
    tunnel: w4 -> [w1203]
    tunnel: w42 -> [w1202]
    tunnel: w41 -> [w1201]
    timing: w13 -> [_]
    timing-out: [_] -> w12
    tunnel: w10 -> [w1194]
    i -> [w1206]
    stop <- w1198 stop-if-true
    n648 = node-c288() -> ()  [unwired: 1 in, 1 out]
    n649 = property on="Main tab control" class="TabCtl (strict)"(error in=w1203) -> (error out=w1193:errorcluster, "Value"=w1208:enum32{"Settings", "Recording", "Analysis"})  [unwired: 1 in, 1 out]
    n650 = case shown="\"Settings\", Default" w1208 {
      tunnel: w1193 -> [w1216 _ _]
      tunnel: w1207 -> [_ w1782 _]
      tunnel: w1194 -> [_ w1784 w2063]
      tunnel: w1206 -> [_ _ _]
      tunnel: w1205 -> [w1213 w1770 w2065]
      tunnel: w1202 -> [_ w1779 _]
      tunnel: w1201 -> [_ w1772 _]
      frame "Settings", Default {
        n651 = flat-sequence {
          tunnel: w1216 -> [w1218]
          tunnel: [w1218] -> w1214
          tunnel: [w1252] -> w1215
          tunnel: w1214 -> [w1252]
          tunnel: [w1450] -> w1212
          tunnel: w1215 -> [w1450]
          tunnel: w1212 -> [w1486]
          tunnel: [w1486] -> w1211
          tunnel: w1211 -> [w1492]
          tunnel: w1213 -> [w1488]
          frame #0 {
            n652 = case shown="True" "Set IO config" {
              frame False {
              }
              frame True {
                w1227 = u16 4 ("y")
                n653 = global read "SW_Globals.vi" "VISA resource name"() -> (w1222:refnum<visa-resource-name>)
                n654 = global read "SW_Globals.vi" "IO parameters cluster"() -> (w1242:T32)
                n655 = local read "Sync capability"() -> (w1224:u8)
                n656 = Greater Than 0?(x=w1224) -> (x > 0?=w1230:bool)
                n657 = call "HW_set_IO_ports_3-pos.vi"("Sync capability"=w1224, "Sync parameters cluster input"=w1242) -> ("Sync parameters cluster output"=w1219:T32)
                n658 = Unbundle By Name(w1219) -> ("IO 1 configuration"=w1225:u16, "IO 2 configuration"=w1226:u16)
                n659 = call "SW_get_config_of_Zones_and_IO.vi"("Sync parameters cluster input"=w1219) -> ("Zones out config bin"=w1232:bool[], "Ports IO config (OUT is FALSE)"=w1231:bool[], "IO inversion config."=w1221:u16)  [unwired: 1 out]
                n660 = global write "SW_Globals.vi" "IO inversion config."(w1221) -> ()
                n661 = call "HW_Set_IO_Dir_on_ECU.vi"("IO ports config"=w1231, "VISA resource name"=w1222, "IO inversion config."=w1221) -> ("error out"=w1223:errorcluster)  [unwired: 1 in, 1 out]
                n662 = global write "SW_Globals.vi" "IO ports config"(w1231) -> ()
                n663 = Equal?(x=w1225, y=w1227) -> (x = y?=w1228:bool)
                n664 = Equal?(x=w1226, y=w1227) -> (x = y?=w1229:bool)
                n665 = global write "SW_Globals.vi" "Zones out config bin"(w1232) -> ()
                n666 = case shown="True" w1230 {
                  tunnel: w1222 -> [_ w1249]
                  tunnel: w1223 -> [_ w1250]
                  tunnel: w1228 -> [_ w1248]
                  tunnel: w1229 -> [_ w1247]
                  frame False {
                  }
                  frame True {
                    n667 = call "SW_Set_SYNC_Status.vi"("error in (no error)"=w1250, "SYNC 2"=w1248, "SYNC 1"=w1247, "VISA Resource name IN"=w1249) -> ()  [unwired: 6 in, 2 out]
                  }
                }
                n668 = global write "SW_Globals.vi" "IO parameters cluster"(w1219) -> ()
                n669 = call "SW_get_config_for_Start_Stop_pulses.vi"("Sync parameters cluster input"=w1219) -> ("Start/Stop out pulses config"=w1236:u32, "Start/Stop in config"=w1235:u32, "Start/Stop in config bin"=w1234:bool[], "Start/Stop out pulses config bin"=w1233:bool[])
                n670 = global write "SW_Globals.vi" "Start/Stop out pulses config bin"(w1233) -> ()
                n671 = global write "SW_Globals.vi" "Start/Stop in config bin"(w1234) -> ()
                n672 = Cluster To Array(cluster=w1219) -> (array=w1220:u16[])
                n673 = call "SW_get_IO_ports_representation.vi"("Sync parameters cluster input"=w1219) -> ("IO status indicator"=w1244:T5)
                n674 = property on="Start/Stop out pulses config" class="DigNum (strict)"("Value"=w1236) -> ()  [unwired: 2 in, 2 out]
                n675 = Equal?(x=w1242, y=w1219) -> (x = y?=w1241:T36)
                n676 = property on="Start/Stop in config" class="DigNum (strict)"("Value"=w1235) -> ()  [unwired: 2 in, 2 out]
                n677 = Cluster To Array(cluster=w1241) -> (array=w1240:bool[])
                n678 = Not(x=w1240) -> (.not. x?=w1239:bool[])
                n679 = Boolean Array To Number(Boolean array=w1239) -> (number=w1238:u32)
                n680 = To Variant(anything=w1244) -> (Variant=w1243:variant)
                n681 = Flatten To JSON(anything=w1220) -> (JSON string=w1246:string, 11:w1245:errorcluster)  [unwired: 2 in]
                n682 = Equal To 0?(x=w1238) -> (x = 0?=w1237:bool)
                n683 = case shown="False" w1237 {
                  frame False {
                    n684 = property on="Changed IO" class="Bool (strict)"("Val(Sgnl)"=TRUE ("Value (Signaling)")) -> ()  [unwired: 2 in, 2 out]
                  }
                  frame True {
                  }
                }
                n685 = property on="IO status indicator" class="Clust"("Value"=w1243) -> ()  [unwired: 2 in, 2 out]
                n686 = property on="IO parameters string" class="Str"(error in=w1245, "Value"=w1246) -> ()  [unwired: 1 in, 2 out]
              }
            }
          }
          frame #1 {
            n687 = event shown="[7] \"Set advanced stimulus\": Value Change" {
              selector: _ -> [_ _ _ _ _ _ _ _]
              dyn-events: _ -> [_ _ _ _ _ _ _ _]
              timeout: 1 -> [_ _ _ _ _ _ _ _]
              event Timeout {
                n688 = event-data() -> ()  [unwired: 1 in, 3 out]
              }
              event "Segments diagram": Mouse Down {
                n689 = event-data() -> ("Coords"=→"Coords":T3, "Button"=→"Button":u16)  [unwired: 1 in, 6 out]
              }
              event "N segments BORDER", "N segments MIDFIELD": Value Change {
                n690 = event-data() -> ()  [unwired: 1 in, 6 out]
                n691 = property on="N segments BORDER" class="DigNum (strict)"() -> (error out=w1258:errorcluster, "Value"=w1261:u8)  [unwired: 2 in, 1 out]
                n692 = property on="N segments MIDFIELD" class="DigNum (strict)"(error in=w1258) -> (error out=w1257:errorcluster, "Value"=w1260:u8)  [unwired: 1 in, 1 out]
                n693 = property on="Zone-based stimulus setup" class="RadioBtnsControl (strict)"(error in=w1257) -> ("Controls[]"=w1259:refnum<vi>[])  [unwired: 1 in, 2 out]
                n694 = Compound Arithmetic op=ADD(w1261, w1260, u8 1 ("value")) -> (w1256:u8)
                n695 = for {
                  tunnel: w1259 -> [w1270] mode=indexing
                  tunnel: w1256 -> [w1266]
                  i -> [w1265]
                  n696 = Increment(x=w1265) -> (x+1=w1264:i32)
                  n697 = Greater Or Equal?(x=w1266, y=w1264) -> (x >= y?=w1263:bool)
                  n698 = Select(t=T10."Enabled" ("Disabled"), s=w1263, f=T10."Disabled and Grayed Out") -> (s? t:f=w1268:T10)
                  n699 = property class="Ctl"(reference=w1270, "DisabledEnum"=w1268) -> ()  [unwired: 1 in, 2 out]
                }
              }
              event "Zone-based stimulus setup": Value Change {
                n700 = event-data() -> ("NewVal"=w1272:T7)  [unwired: 1 in, 5 out]
                n701 = To Unsigned Byte Integer(number=w1272) -> (unsigned 8bit integer=w1271:u8)
                n702 = case shown="1.." w1271 {
                  selector: w1271 -> [w1273 w1276]
                  frame 0, Default {
                    n703 = Build Array(w1273) -> (w1275:u8[])
                    n704 = property on="Stimulus presets" class="Arr (strict)"("Index Values"=w1275, "DisabledEnum"=T10."Disabled and Grayed Out" ("Disabled")) -> ()  [unwired: 2 in, 2 out]
                  }
                  frame 1.. {
                    n705 = Build Array(w1276) -> (w1278:u8[])
                    n706 = property on="Stimulus presets" class="Arr (strict)"("Index Values"=w1278, "DisabledEnum"=T10."Enabled" ("Disabled")) -> ()  [unwired: 2 in, 2 out]
                  }
                }
              }
              event "Stimulus presets": Value Change {
                n707 = event-data() -> ("NewVal"=w1279:T6)  [unwired: 1 in, 5 out]
                n708 = property on="Stimulus presets" class="Arr (strict)"() -> ("Index Values"=w1296:u32[])  [unwired: 2 in, 2 out]
                n709 = Index Array(array=w1296, index=0) -> (element=w1280:u32)
                n710 = Index Array(array=w1279, index=w1280) -> (element=w1289:T37)
                n711 = Unbundle By Name(w1289) -> ("Set/Clear"=w1290:bool, "Time, s"=w1284:sgl, "Stimulus, s"=w1282:sgl)
                n712 = property on="Zone-based stimulus setup" class="RadioBtnsControl (strict)"() -> ("Value"=w1294:T7)  [unwired: 2 in, 2 out]
                n713 = Format Into String(w1294) -> ()  [unwired: 3 in, 2 out]
                n714 = Greater Than 0?(x=w1284) -> (x > 0?=w1292:bool)
                n715 = Greater Than 0?(x=w1282) -> (x > 0?=w1291:bool)
                n716 = expression code="floor(x * 100) / 100"(w1284) -> (w1283:sgl)
                n717 = expression code="floor(x * 100) / 100"(w1282) -> (w1281:sgl)
                n718 = To Unsigned Byte Integer(number=w1294) -> (unsigned 8bit integer=w1293:u8)
                n719 = Compound Arithmetic op=AND(w1290, w1292, w1291) -> (w1287:bool)
                n720 = case shown="6" w1293 {
                  tunnel: w1287 -> [_ w1302 w1306 w1310 w1314 w1318 w1322 w1326 w1330 w1334 w1338 w1342 w1346 w1350]
                  frame 0, Default {
                  }
                  frame 1 {
                    n721 = property on="Colors for Stim. setup" class="Arr (strict)"() -> ("Value"=w1301:T2)  [unwired: 2 in, 2 out]
                    n722 = Select(t=w1301, s=w1302, f=T9 [{"Numeric Control"=12369084, "Numeric Control"=12369084}, {"Numeric Control"=6603023, "Numeric Control"=6603023}, {"Numeric Control"=1976113, "Numeric Control"=1976113}, {"Numeric Control"=2575993, "Numeric Control"=2575993}] ("Colors [4] 2")) -> (s? t:f=w1304:T9)
                    n723 = property on="Zone 01" class="Bool (strict)"("Colors [4]"=w1304) -> ()  [unwired: 2 in, 2 out]
                  }
                  frame 2 {
                    n724 = property on="Colors for Stim. setup" class="Arr (strict)"() -> ("Value"=w1305:T2)  [unwired: 2 in, 2 out]
                    n725 = Select(t=w1305, s=w1306, f=T9 [{"Numeric Control"=12369084, "Numeric Control"=12369084}, {"Numeric Control"=6603023, "Numeric Control"=6603023}, {"Numeric Control"=1976113, "Numeric Control"=1976113}, {"Numeric Control"=2575993, "Numeric Control"=2575993}] ("Colors [4] 2")) -> (s? t:f=w1308:T9)
                    n726 = property on="Zone 02" class="Bool (strict)"("Colors [4]"=w1308) -> ()  [unwired: 2 in, 2 out]
                  }
                  frame 3 {
                    n727 = property on="Colors for Stim. setup" class="Arr (strict)"() -> ("Value"=w1309:T2)  [unwired: 2 in, 2 out]
                    n728 = Select(t=w1309, s=w1310, f=T9 [{"Numeric Control"=12369084, "Numeric Control"=12369084}, {"Numeric Control"=6603023, "Numeric Control"=6603023}, {"Numeric Control"=1976113, "Numeric Control"=1976113}, {"Numeric Control"=2575993, "Numeric Control"=2575993}] ("Colors [4] 2")) -> (s? t:f=w1312:T9)
                    n729 = property on="Zone 03" class="Bool (strict)"("Colors [4]"=w1312) -> ()  [unwired: 2 in, 2 out]
                  }
                  frame 4 {
                    n730 = property on="Colors for Stim. setup" class="Arr (strict)"() -> ("Value"=w1313:T2)  [unwired: 2 in, 2 out]
                    n731 = Select(t=w1313, s=w1314, f=T9 [{"Numeric Control"=12369084, "Numeric Control"=12369084}, {"Numeric Control"=6603023, "Numeric Control"=6603023}, {"Numeric Control"=1976113, "Numeric Control"=1976113}, {"Numeric Control"=2575993, "Numeric Control"=2575993}] ("Colors [4] 2")) -> (s? t:f=w1316:T9)
                    n732 = property on="Zone 04" class="Bool (strict)"("Colors [4]"=w1316) -> ()  [unwired: 2 in, 2 out]
                  }
                  frame 5 {
                    n733 = property on="Colors for Stim. setup" class="Arr (strict)"() -> ("Value"=w1317:T2)  [unwired: 2 in, 2 out]
                    n734 = Select(t=w1317, s=w1318, f=T9 [{"Numeric Control"=12369084, "Numeric Control"=12369084}, {"Numeric Control"=6603023, "Numeric Control"=6603023}, {"Numeric Control"=1976113, "Numeric Control"=1976113}, {"Numeric Control"=2575993, "Numeric Control"=2575993}] ("Colors [4] 2")) -> (s? t:f=w1320:T9)
                    n735 = property on="Zone 05" class="Bool (strict)"("Colors [4]"=w1320) -> ()  [unwired: 2 in, 2 out]
                  }
                  frame 6 {
                    n736 = property on="Colors for Stim. setup" class="Arr (strict)"() -> ("Value"=w1321:T2)  [unwired: 2 in, 2 out]
                    n737 = Select(t=w1321, s=w1322, f=T9 [{"Numeric Control"=12369084, "Numeric Control"=12369084}, {"Numeric Control"=6603023, "Numeric Control"=6603023}, {"Numeric Control"=1976113, "Numeric Control"=1976113}, {"Numeric Control"=2575993, "Numeric Control"=2575993}] ("Colors [4] 2")) -> (s? t:f=w1324:T9)
                    n738 = property on="Zone 06" class="Bool (strict)"("Colors [4]"=w1324) -> ()  [unwired: 2 in, 2 out]
                  }
                  frame 7 {
                    n739 = property on="Colors for Stim. setup" class="Arr (strict)"() -> ("Value"=w1325:T2)  [unwired: 2 in, 2 out]
                    n740 = Select(t=w1325, s=w1326, f=T9 [{"Numeric Control"=12369084, "Numeric Control"=12369084}, {"Numeric Control"=6603023, "Numeric Control"=6603023}, {"Numeric Control"=1976113, "Numeric Control"=1976113}, {"Numeric Control"=2575993, "Numeric Control"=2575993}] ("Colors [4] 2")) -> (s? t:f=w1328:T9)
                    n741 = property on="Zone 07" class="Bool (strict)"("Colors [4]"=w1328) -> ()  [unwired: 2 in, 2 out]
                  }
                  frame 8 {
                    n742 = property on="Colors for Stim. setup" class="Arr (strict)"() -> ("Value"=w1329:T2)  [unwired: 2 in, 2 out]
                    n743 = Select(t=w1329, s=w1330, f=T9 [{"Numeric Control"=12369084, "Numeric Control"=12369084}, {"Numeric Control"=6603023, "Numeric Control"=6603023}, {"Numeric Control"=1976113, "Numeric Control"=1976113}, {"Numeric Control"=2575993, "Numeric Control"=2575993}] ("Colors [4] 2")) -> (s? t:f=w1332:T9)
                    n744 = property on="Zone 08" class="Bool (strict)"("Colors [4]"=w1332) -> ()  [unwired: 2 in, 2 out]
                  }
                  frame 9 {
                    n745 = property on="Colors for Stim. setup" class="Arr (strict)"() -> ("Value"=w1333:T2)  [unwired: 2 in, 2 out]
                    n746 = Select(t=w1333, s=w1334, f=T9 [{"Numeric Control"=12369084, "Numeric Control"=12369084}, {"Numeric Control"=6603023, "Numeric Control"=6603023}, {"Numeric Control"=1976113, "Numeric Control"=1976113}, {"Numeric Control"=2575993, "Numeric Control"=2575993}] ("Colors [4] 2")) -> (s? t:f=w1336:T9)
                    n747 = property on="Zone 09" class="Bool (strict)"("Colors [4]"=w1336) -> ()  [unwired: 2 in, 2 out]
                  }
                  frame 10 {
                    n748 = property on="Colors for Stim. setup" class="Arr (strict)"() -> ("Value"=w1337:T2)  [unwired: 2 in, 2 out]
                    n749 = Select(t=w1337, s=w1338, f=T9 [{"Numeric Control"=12369084, "Numeric Control"=12369084}, {"Numeric Control"=6603023, "Numeric Control"=6603023}, {"Numeric Control"=1976113, "Numeric Control"=1976113}, {"Numeric Control"=2575993, "Numeric Control"=2575993}] ("Colors [4] 2")) -> (s? t:f=w1340:T9)
                    n750 = property on="Zone 10" class="Bool (strict)"("Colors [4]"=w1340) -> ()  [unwired: 2 in, 2 out]
                  }
                  frame 11 {
                    n751 = property on="Colors for Stim. setup" class="Arr (strict)"() -> ("Value"=w1341:T2)  [unwired: 2 in, 2 out]
                    n752 = Select(t=w1341, s=w1342, f=T9 [{"Numeric Control"=12369084, "Numeric Control"=12369084}, {"Numeric Control"=6603023, "Numeric Control"=6603023}, {"Numeric Control"=1976113, "Numeric Control"=1976113}, {"Numeric Control"=2575993, "Numeric Control"=2575993}] ("Colors [4] 2")) -> (s? t:f=w1344:T9)
                    n753 = property on="Zone 11" class="Bool (strict)"("Colors [4]"=w1344) -> ()  [unwired: 2 in, 2 out]
                  }
                  frame 12 {
                    n754 = property on="Colors for Stim. setup" class="Arr (strict)"() -> ("Value"=w1345:T2)  [unwired: 2 in, 2 out]
                    n755 = Select(t=w1345, s=w1346, f=T9 [{"Numeric Control"=12369084, "Numeric Control"=12369084}, {"Numeric Control"=6603023, "Numeric Control"=6603023}, {"Numeric Control"=1976113, "Numeric Control"=1976113}, {"Numeric Control"=2575993, "Numeric Control"=2575993}] ("Colors [4] 2")) -> (s? t:f=w1348:T9)
                    n756 = property on="Zone 12" class="Bool (strict)"("Colors [4]"=w1348) -> ()  [unwired: 2 in, 2 out]
                  }
                  frame 13 {
                    n757 = property on="Colors for Stim. setup" class="Arr (strict)"() -> ("Value"=w1349:T2)  [unwired: 2 in, 2 out]
                    n758 = Select(t=w1349, s=w1350, f=T9 [{"Numeric Control"=12369084, "Numeric Control"=12369084}, {"Numeric Control"=6603023, "Numeric Control"=6603023}, {"Numeric Control"=1976113, "Numeric Control"=1976113}, {"Numeric Control"=2575993, "Numeric Control"=2575993}] ("Colors [4] 2")) -> (s? t:f=w1352:T9)
                    n759 = property on="Zone 13" class="Bool (strict)"("Colors [4]"=w1352) -> ()  [unwired: 2 in, 2 out]
                  }
                }
                n760 = Bundle By Name(cluster=w1289, "Stim. has been set"=w1287, "Set/Clear"=w1287, "Time, s"=w1283, "Stimulus, s"=w1281) -> (w1288:T37)
                n761 = Replace Array Subset(array=w1279, new element=w1288, index=w1280) -> (w1285:T6)
                n762 = for {
                  tunnel: w1285 -> [w1300] mode=indexing
                  tunnel: [w1297] -> w1286 mode=indexing if=w1298
                  i -> [w1299]
                  n763 = Unbundle By Name(w1300) -> ("Stim. has been set"=w1298:bool)
                  n764 = To Unsigned Byte Integer(number=w1299) -> (unsigned 8bit integer=w1297:u8)
                }
                n765 = global write "SW_Globals.vi" "Stimulus presets"(w1285) -> ()
                n766 = property on="Stimulus presets" class="Arr (strict)"("Value"=w1285) -> ()  [unwired: 2 in, 2 out]
                n767 = global write "SW_Globals.vi" "Regions to track"(w1286) -> ()
              }
              event "Reset stimuli", "Changed IO": Value Change {
                n768 = event-data() -> ("OldVal"=w1354:bool, "NewVal"=w1355:bool)  [unwired: 1 in, 4 out]
                n769 = property on="Reset stimuli" class="Bool (strict)"("Value"=w1354) -> ()  [unwired: 2 in, 2 out]
                n770 = property on="Changed IO" class="Bool (strict)"("Value"=FALSE ("Changed IO")) -> ()  [unwired: 2 in, 2 out]
                n771 = case shown="True" w1355 {
                  selector: w1355 -> [_ w1379]
                  frame False {
                  }
                  frame True {
                    w1367 = T9 [{"Numeric Control"=9868950, "Numeric Control"=15790320}, {"Numeric Control"=8388608, "Numeric Control"=8388608}, {"Numeric Control"=4934475, "Numeric Control"=7895160}, {"Numeric Control"=994319, "Numeric Control"=1657881}]  # TTL IO In colors
                    w1368 = T9 [{"Numeric Control"=9868950, "Numeric Control"=15790320}, {"Numeric Control"=1988894, "Numeric Control"=3381555}, {"Numeric Control"=4934475, "Numeric Control"=7895160}, {"Numeric Control"=994319, "Numeric Control"=1657881}]  # TTL IO Out colors
                    (unwired) T38 [{"String"="1", "Value"=1}, {"String"="2", "Value"=2}, {"String"="1+2", "Value"=3}, {"String"="5+6", "Value"=4}] ("Strings And Values")
                    n772 = global write "SW_Globals.vi" "Regions to track"(u8[] []) -> ()
                    n773 = global read "SW_Globals.vi" "IO ports config"() -> (w1366:bool[])
                    n774 = Index Array(array=w1366, index=0) -> (element=w1372:bool)
                    n775 = Index Array(array=w1366, index=1) -> (element=w1371:bool)
                    n776 = Index Array(array=w1366, index=2) -> (element=w1370:bool)
                    n777 = Index Array(array=w1366, index=3) -> (element=w1369:bool)
                    n778 = Select(t=w1367, s=w1372, f=w1368) -> (s? t:f=w1365:T9)
                    n779 = Select(t=w1367, s=w1371, f=w1368) -> (s? t:f=w1364:T9)
                    n780 = Select(t=w1367, s=w1369, f=w1368) -> (s? t:f=w1362:T9)
                    n781 = Select(t=w1367, s=w1370, f=w1368) -> (s? t:f=w1363:T9)
                    n782 = property on="TTL IO 1 (recording)" class="Bool (strict)"("Colors [4]"=w1365) -> ()  [unwired: 2 in, 2 out]
                    n783 = property on="TTL IO 3 (recording)" class="Bool (strict)"("Colors [4]"=w1363) -> ()  [unwired: 2 in, 2 out]
                    n784 = property on="TTL IO 2 (recording)" class="Bool (strict)"("Colors [4]"=w1364) -> ()  [unwired: 2 in, 2 out]
                    n785 = property on="TTL IO 4 (recording)" class="Bool (strict)"("Colors [4]"=w1362) -> ()  [unwired: 2 in, 2 out]
                    n786 = property on="TTL IO 1 (analysis)" class="Bool"("Colors [4]"=w1365) -> ()  [unwired: 2 in, 2 out]
                    n787 = property on="TTL IO 3 (analysis)" class="Bool"("Colors [4]"=w1363) -> ()  [unwired: 2 in, 2 out]
                    n788 = property on="TTL IO 2 (analysis)" class="Bool"("Colors [4]"=w1364) -> ()  [unwired: 2 in, 2 out]
                    n789 = property on="TTL IO 4 (analysis)" class="Bool"("Colors [4]"=w1362) -> ()  [unwired: 2 in, 2 out]
                    n790 = global read "SW_Globals.vi" "IO parameters cluster"() -> (w1378:T32)
                    n791 = Unbundle By Name(w1378) -> ("SYNC configuration"=w1377:u16, "IO 1 configuration"=w1357:u16, "IO 2 configuration"=w1356:u16)
                    n792 = call "SW_Gen_Available_TTL_outputs_array.vi"("IO 2 configuration"=w1356, "IO 1 configuration"=w1357, "SYNC configuration"=w1377) -> ("Available TTL outputs array"=w1361:cluster{"String":string, "Value":i32}[])
                    n793 = Index Array(array=w1361, index=0) -> (element=w1359:cluster{"String":string, "Value":i32})
                    n794 = property on="TTL out" class="Ring (strict)"("StringsAndValues[]"=w1361) -> ()  [unwired: 2 in, 2 out]
                    n795 = Unbundle By Name(w1359) -> ("Value"=w1358:i32)
                    n796 = for {
                      N: 14 -> [_]
                      tunnel: [w1387] -> w1384 mode=indexing
                      tunnel: [w1388] -> w1380
                      tunnel: w1379 -> [w1388]
                      tunnel: w1358 -> [w1385]
                      i -> [w1389]
                      n797 = case shown="6" w1389 {
                        frame 0, Default {
                        }
                        frame 1 {
                          n798 = property on="Zone 01" class="Bool (strict)"("Colors [4]"=T9 [{"Numeric Control"=12369084, "Numeric Control"=12369084}, {"Numeric Control"=6603023, "Numeric Control"=6603023}, {"Numeric Control"=1976113, "Numeric Control"=1976113}, {"Numeric Control"=2575993, "Numeric Control"=2575993}] ("Colors [4] 2"), "Value"=FALSE) -> ()  [unwired: 2 in, 2 out]
                        }
                        frame 2 {
                          n799 = property on="Zone 02" class="Bool (strict)"("Colors [4]"=T9 [{"Numeric Control"=12369084, "Numeric Control"=12369084}, {"Numeric Control"=6603023, "Numeric Control"=6603023}, {"Numeric Control"=1976113, "Numeric Control"=1976113}, {"Numeric Control"=2575993, "Numeric Control"=2575993}] ("Colors [4] 2"), "Value"=FALSE) -> ()  [unwired: 2 in, 2 out]
                        }
                        frame 3 {
                          n800 = property on="Zone 03" class="Bool (strict)"("Colors [4]"=T9 [{"Numeric Control"=12369084, "Numeric Control"=12369084}, {"Numeric Control"=6603023, "Numeric Control"=6603023}, {"Numeric Control"=1976113, "Numeric Control"=1976113}, {"Numeric Control"=2575993, "Numeric Control"=2575993}] ("Colors [4] 2"), "Value"=FALSE) -> ()  [unwired: 2 in, 2 out]
                        }
                        frame 4 {
                          n801 = property on="Zone 04" class="Bool (strict)"("Colors [4]"=T9 [{"Numeric Control"=12369084, "Numeric Control"=12369084}, {"Numeric Control"=6603023, "Numeric Control"=6603023}, {"Numeric Control"=1976113, "Numeric Control"=1976113}, {"Numeric Control"=2575993, "Numeric Control"=2575993}] ("Colors [4] 2"), "Value"=FALSE) -> ()  [unwired: 2 in, 2 out]
                        }
                        frame 5 {
                          n802 = property on="Zone 05" class="Bool (strict)"("Colors [4]"=T9 [{"Numeric Control"=12369084, "Numeric Control"=12369084}, {"Numeric Control"=6603023, "Numeric Control"=6603023}, {"Numeric Control"=1976113, "Numeric Control"=1976113}, {"Numeric Control"=2575993, "Numeric Control"=2575993}] ("Colors [4] 2"), "Value"=FALSE) -> ()  [unwired: 2 in, 2 out]
                        }
                        frame 6 {
                          n803 = property on="Zone 06" class="Bool (strict)"("Colors [4]"=T9 [{"Numeric Control"=12369084, "Numeric Control"=12369084}, {"Numeric Control"=6603023, "Numeric Control"=6603023}, {"Numeric Control"=1976113, "Numeric Control"=1976113}, {"Numeric Control"=2575993, "Numeric Control"=2575993}] ("Colors [4] 2"), "Value"=FALSE) -> ()  [unwired: 2 in, 2 out]
                        }
                        frame 7 {
                          n804 = property on="Zone 07" class="Bool (strict)"("Colors [4]"=T9 [{"Numeric Control"=12369084, "Numeric Control"=12369084}, {"Numeric Control"=6603023, "Numeric Control"=6603023}, {"Numeric Control"=1976113, "Numeric Control"=1976113}, {"Numeric Control"=2575993, "Numeric Control"=2575993}] ("Colors [4] 2"), "Value"=FALSE) -> ()  [unwired: 2 in, 2 out]
                        }
                        frame 8 {
                          n805 = property on="Zone 08" class="Bool (strict)"("Colors [4]"=T9 [{"Numeric Control"=12369084, "Numeric Control"=12369084}, {"Numeric Control"=6603023, "Numeric Control"=6603023}, {"Numeric Control"=1976113, "Numeric Control"=1976113}, {"Numeric Control"=2575993, "Numeric Control"=2575993}] ("Colors [4] 2"), "Value"=FALSE) -> ()  [unwired: 2 in, 2 out]
                        }
                        frame 9 {
                          n806 = property on="Zone 09" class="Bool (strict)"("Colors [4]"=T9 [{"Numeric Control"=12369084, "Numeric Control"=12369084}, {"Numeric Control"=6603023, "Numeric Control"=6603023}, {"Numeric Control"=1976113, "Numeric Control"=1976113}, {"Numeric Control"=2575993, "Numeric Control"=2575993}] ("Colors [4] 2"), "Value"=FALSE) -> ()  [unwired: 2 in, 2 out]
                        }
                        frame 10 {
                          n807 = property on="Zone 10" class="Bool (strict)"("Colors [4]"=T9 [{"Numeric Control"=12369084, "Numeric Control"=12369084}, {"Numeric Control"=6603023, "Numeric Control"=6603023}, {"Numeric Control"=1976113, "Numeric Control"=1976113}, {"Numeric Control"=2575993, "Numeric Control"=2575993}] ("Colors [4] 2"), "Value"=FALSE) -> ()  [unwired: 2 in, 2 out]
                        }
                        frame 11 {
                          n808 = property on="Zone 11" class="Bool (strict)"("Colors [4]"=T9 [{"Numeric Control"=12369084, "Numeric Control"=12369084}, {"Numeric Control"=6603023, "Numeric Control"=6603023}, {"Numeric Control"=1976113, "Numeric Control"=1976113}, {"Numeric Control"=2575993, "Numeric Control"=2575993}] ("Colors [4] 2"), "Value"=FALSE) -> ()  [unwired: 2 in, 2 out]
                        }
                        frame 12 {
                          n809 = property on="Zone 12" class="Bool (strict)"("Colors [4]"=T9 [{"Numeric Control"=12369084, "Numeric Control"=12369084}, {"Numeric Control"=6603023, "Numeric Control"=6603023}, {"Numeric Control"=1976113, "Numeric Control"=1976113}, {"Numeric Control"=2575993, "Numeric Control"=2575993}] ("Colors [4] 2"), "Value"=FALSE) -> ()  [unwired: 2 in, 2 out]
                        }
                        frame 13 {
                          n810 = property on="Zone 13" class="Bool (strict)"("Colors [4]"=T9 [{"Numeric Control"=12369084, "Numeric Control"=12369084}, {"Numeric Control"=6603023, "Numeric Control"=6603023}, {"Numeric Control"=1976113, "Numeric Control"=1976113}, {"Numeric Control"=2575993, "Numeric Control"=2575993}] ("Colors [4] 2"), "Value"=FALSE) -> ()  [unwired: 2 in, 2 out]
                        }
                      }
                      n811 = Bundle By Name(cluster=T35 {"Event type"=0, "Cond., s"=0.0, "Stim., s"=0.0, "Set/Clear"=FALSE, "TTL out N"=1, "Stim. has been set"=FALSE} ("Cluster of the stimuls settings"), "TTL out N"=w1385) -> (w1387:T35)
                    }
                    n812 = global write "SW_Globals.vi" "Stimulus presets"(w1384) -> ()
                    n813 = property on="Stimulus presets" class="Arr (strict)"("Value"=w1384) -> (error out=w1381:errorcluster)  [unwired: 2 in, 1 out]
                    n814 = property on="Reset STIM" class="Bool (strict)"(error in=w1381, "Val(Sgnl)"=w1380) -> ()  [unwired: 1 in, 2 out]
                  }
                }
              }
              event "Reset regions": Value Change {
                n815 = event-data() -> ("OldVal"=w1416:bool, "NewVal"=w1417:bool)  [unwired: 1 in, 4 out]
                n816 = property on="Reset regions" class="Bool (strict)"("Value"=w1416) -> ()  [unwired: 2 in, 2 out]
                n817 = case shown="True" w1417 {
                  selector: w1417 -> [_ w1419]
                  frame False {
                  }
                  frame True {
                    n818 = local read "Cage diameter, mm"() -> (w1420:u16)
                    n819 = case shown="327" w1420 {
                      tunnel: w1419 -> [w1421 w1428 w1435 w1442]
                      tunnel: [w1421 w1428 w1435 w1442] -> w1418
                      frame 180, Default {
                        n820 = local write "Starting angle BORDER"(i16 0 ("Starting angle")) -> ()
                        n821 = local write "Starting angle MIDFIELD"(i16 0 ("Starting angle")) -> ()
                        n822 = local write "N segments MIDFIELD"(u8 2 ("N segments")) -> ()
                        n823 = local write "N segments BORDER"(u8 4 ("N segments")) -> ()
                        n824 = local write "Radius, mm CENTER"(u16 30 ("Radius, mm")) -> ()
                        n825 = local write "Radius, mm MIDFIELD"(u16 75 ("Radius, mm")) -> ()
                      }
                      frame 325 {
                        n826 = local write "Starting angle BORDER"(i16 0 ("Starting angle")) -> ()
                        n827 = local write "Starting angle MIDFIELD"(i16 0 ("Starting angle")) -> ()
                        n828 = local write "N segments MIDFIELD"(u8 2 ("N segments")) -> ()
                        n829 = local write "N segments BORDER"(u8 4 ("N segments")) -> ()
                        n830 = local write "Radius, mm CENTER"(u16 50 ("Radius, mm")) -> ()
                        n831 = local write "Radius, mm MIDFIELD"(u16 148 ("Radius, mm")) -> ()
                      }
                      frame 327 {
                        n832 = local write "Starting angle BORDER"(i16 0 ("Starting angle")) -> ()
                        n833 = local write "Starting angle MIDFIELD"(i16 0 ("Starting angle")) -> ()
                        n834 = local write "N segments MIDFIELD"(u8 2 ("N segments")) -> ()
                        n835 = local write "N segments BORDER"(u8 4 ("N segments")) -> ()
                        n836 = local write "Radius, mm CENTER"(u16 50 ("Radius, mm")) -> ()
                        n837 = local write "Radius, mm MIDFIELD"(u16 150 ("Radius, mm")) -> ()
                      }
                      frame 333 {
                        n838 = local write "Starting angle BORDER"(i16 0 ("Starting angle")) -> ()
                        n839 = local write "Starting angle MIDFIELD"(i16 0 ("Starting angle")) -> ()
                        n840 = local write "N segments MIDFIELD"(u8 2 ("N segments")) -> ()
                        n841 = local write "N segments BORDER"(u8 4 ("N segments")) -> ()
                        n842 = local write "Radius, mm CENTER"(u16 50 ("Radius, mm")) -> ()
                        n843 = local write "Radius, mm MIDFIELD"(u16 152 ("Radius, mm")) -> ()
                      }
                    }
                    n844 = property on="Reset REG" class="Bool (strict)"("Val(Sgnl)"=w1418) -> ()  [unwired: 2 in, 2 out]
                  }
                }
              }
              event "Set advanced stimulus": Value Change {
                n845 = event-data() -> ("OldVal"=w1449:bool)  [unwired: 1 in, 5 out]
                n846 = property on="Set advanced stimulus" class="Bool (strict)"("Value"=w1449) -> ()  [unwired: 2 in, 2 out]
                n847 = call "SW_Set_Adv_Stimulus_interface.vi"() -> ()  [unwired: 6 in]
              }
            }
          }
          frame #2 {
            # "Segments scheme can be reset here"
            n848 = First Call?() -> (First Call?: T/F=w1452:bool)
            n849 = case shown="True" w1452 {
              selector: w1452 -> [_ w1455]
              tunnel: [_ w1454] -> w1453
              frame False {
              }
              frame True {
                n850 = property on="Init plot" class="Bool (strict)"("Val(Sgnl)"=w1455) -> (error out=w1454:errorcluster)  [unwired: 2 in, 1 out]
              }
            }
            n851 = event shown="[0] \"Init plot\", \"Zone-based stimulus setup\", \"N segments MIDFIELD\", \"N segments BORDER\", \"Starting angle MIDFIELD\", \"Starting angle BORDER\", \"Radius, mm MIDFIELD\", \"Radius, mm CENTER\", \"Cage diameter, mm\", \"Reset stimuli\", \"Reset regions\", \"Reset REG\", \"Reset STIM\": Value Change" {
              selector: _ -> [_ _]
              dyn-events: _ -> [_ _]
              timeout: 1 -> [_ _]
              tunnel: w1453 -> [_ _]
              event "Init plot", "Zone-based stimulus setup", "N segments MIDFIELD", "N segments BORDER", "Starting angle MIDFIELD", "Starting angle BORDER", "Radius, mm MIDFIELD", "Radius, mm CENTER", "Cage diameter, mm", "Reset stimuli", "Reset regions", "Reset REG", "Reset STIM": Value Change {
                n852 = event-data() -> ()  [unwired: 1 in, 6 out]
                n853 = local read "Cage diameter, mm"() -> (w1456:u16)
                n854 = global read "SW_Globals.vi" "Regions to track"() -> (w1478:u8[])
                n855 = To Unsigned Byte Integer(number="Zone-based stimulus setup") -> (unsigned 8bit integer=w1479:u8)
                n856 = case "Let's set flag for alternative magnets orintation" shown="180, Default" w1456 {
                  frame 180, Default {
                    n857 = global write "SW_Globals.vi" "Alternative magnets orientation"(FALSE ("Alternative magnets orientation")) -> ()
                  }
                  frame 325 {
                    n858 = global write "SW_Globals.vi" "Alternative magnets orientation"(FALSE ("Alternative magnets orientation")) -> ()
                  }
                  frame 327 {
                    n859 = global write "SW_Globals.vi" "Alternative magnets orientation"(TRUE ("Alternative magnets orientation")) -> ()
                  }
                  frame 333 {
                    n860 = global write "SW_Globals.vi" "Alternative magnets orientation"(FALSE ("Alternative magnets orientation")) -> ()
                  }
                }
                n861 = property on="Segments diagram" class="Pict"() -> ("Bounds"=w1476:T16)  [unwired: 2 in, 2 out]
                n862 = Bundle("N segments BORDER"="N segments BORDER", "Starting angle BORDER"="Starting angle BORDER", "N segments MIDFIELD"="N segments MIDFIELD", "Starting angle MIDFIELD"="Starting angle MIDFIELD", "Radius, mm MIDFIELD"="Radius, mm MIDFIELD", u8 1, "Radius, mm CENTER"="Radius, mm CENTER", "Cage diameter, mm"=w1456, 10) -> (w1466:T39)  [unwired: 1 in]
                n863 = Build Array(w1479) -> (w1475:u8[])
                n864 = Build Array (concatenate)(w1475, w1478) -> (w1477:u8[])
                n865 = call "SW_Gen_Check_segments_parameters.vi"("Image plotting parameters"=w1466) -> ("Corrected image plotting parameters"=w1465:T40)  [unwired: 2 in]
                n866 = Unbundle By Name(w1465) -> ("N segments BORDER"=w1464:u8, "N segments MIDFIELD"=w1462:u8, "Radius, mm MIDFIELD"=w1461:u16, "Radius, mm CENTER"=w1463:u16)
                n867 = call "SW_Generate_Segmented_Plot_v3.vi"("Draw Area Size"=w1476, "Regions to mark set"=w1477, "Regions to mark selected"=w1475, "Input cluster of parameters"=w1465) -> ("Zones layout output"=w1458:picture, "No zones image"=w1457:picture, "Array of the pixel to color correspondences"=w1459:u32[][], "Array of the segment to color correspondences"=w1460:u32[][])  [unwired: 6 in, 2 out]
                "Segments diagram" <- w1458
                n868 = global write "SW_Globals.vi" "Diagram"(w1458) -> ()
                n869 = global write "SW_Globals.vi" "Diagram no zones"(w1457) -> ()
                n870 = global write "SW_Globals.vi" "Array of the pixel to color correspondences"(w1459) -> ()
                n871 = global write "SW_Globals.vi" "Array of the segment to color correspondences"(w1460) -> ()
                n872 = property on="N segments BORDER" class="DigNum (strict)"("Value"=w1464) -> ()  [unwired: 2 in, 2 out]
                n873 = property on="N segments MIDFIELD" class="DigNum (strict)"("Value"=w1462) -> ()  [unwired: 2 in, 2 out]
                n874 = property on="Radius, mm MIDFIELD" class="DigNum (strict)"("Value"=w1461) -> ()  [unwired: 2 in, 2 out]
                n875 = property on="Radius, mm CENTER" class="DigNum (strict)"("Value"=w1463) -> ()  [unwired: 2 in, 2 out]
                n876 = global write "SW_Globals.vi" "Full track with zones"(w1458) -> ()
                n877 = global write "SW_Globals.vi" "Full track with no zones"(w1457) -> ()
              }
              event Timeout {
                n878 = event-data() -> ()  [unwired: 1 in, 3 out]
              }
            }
          }
          frame #3 {
            n879 = property on="Jump to Analysis" class="Bool (strict)"("Value"=TRUE ("Jump to Analysis")) -> ()  [unwired: 2 in, 2 out]
          }
          frame #4 {
            # "Save settings and set important variables befor actual start of the recording. Also initial \"Play\" command is sent from here."
            n880 = Build Array("Start Tracking button", "Jump to Analysis") -> (w1490:bool[])
            n881 = Boolean Array To Number(Boolean array=w1490) -> (number=w1487:u32)
            n882 = case shown="2" w1487 {
              tunnel: w1492 -> [_ w1560 w1690]
              tunnel: w1488 -> [_ w1502 _]
              frame 0, Default {
              }
              frame 1 {
                w1503 = T41 {"Zone[1]"=FALSE, "Zone[2]"=FALSE, "Zone[3]"=FALSE, "Zone[4]"=FALSE, "Zone[5]"=FALSE, "Zone[6]"=FALSE, "Zone[7]"=FALSE, "Zone[8]"=FALSE, "Zone[9]"=FALSE, "Zone[10]"=FALSE, "Zone[11]"=FALSE, "Zone[12]"=FALSE, "Zone[13]"=FALSE} ("Zones presence indicator")
                w1594 = enum32{"Settings", "Recording", "Analysis"}."Recording" ("Main tab control")
                w1598 = enum32{"Settings", "Recording", "Analysis"}."Analysis" ("Main tab control")
                w1607 = enum32{"Settings", "Recording", "Analysis"}."Settings" ("Main tab control")
                n883 = flat-sequence {
                  tunnel: w1560 -> [w1654]
                  tunnel: w1502 -> [w1648]
                  tunnel: [w1654] -> w1559
                  tunnel: w1559 -> [w1656]
                  tunnel: [w1656] -> w1512
                  tunnel: [w1659] -> w1537
                  tunnel: w1512 -> [w1666]
                  frame #0 {
                    n884 = Unbundle By Name(w1648) -> ("Play/Pause status"=w1652:refnum<notifier>, "Recording now"=w1647:refnum<notifier>, "Final CSV saved"=w1644:refnum<notifier>, "Data loaded"=w1642:refnum<notifier>, "Temp file ready for processing"=w1641:refnum<notifier>, "Has been recorded"=w1638:refnum<notifier>)  [unwired: 1 out]
                    n885 = Send Notification(notification=FALSE, notifier=w1638) -> ()  [unwired: 1 in, 2 out]
                    n886 = Select(t="Play", s=TRUE, f="Pause") -> (s? t:f=w1651:string)
                    n887 = Send Notification(notification=w1651, notifier=w1652) -> ()  [unwired: 1 in, 2 out]
                    n888 = Send Notification(notification=FALSE, notifier=w1647) -> ()  [unwired: 1 in, 2 out]
                    n889 = Send Notification(notification=FALSE, notifier=w1644) -> ()  [unwired: 1 in, 2 out]
                    n890 = Send Notification(notification=FALSE, notifier=w1642) -> ()  [unwired: 1 in, 2 out]
                    n891 = Send Notification(notification=FALSE, notifier=w1641) -> ()  [unwired: 1 in, 2 out]
                  }
                  frame #1 {
                    n892 = Wait (ms)(milliseconds to wait=u32 1500) -> ()  [unwired: 1 out]
                  }
                  frame #2 {
                    n893 = global read "SW_Globals.vi" "Zones allocation array"() -> (w1668:i32[])
                    n894 = global write "SW_Globals.vi" "Incrementally save First Call"(TRUE ("Incrementally save First Call")) -> ()
                    n895 = Array Size(array=w1668) -> (size(s)=w1667:i32)
                    n896 = property on="Jump to Analysis" class="Bool (strict)"(error in=w1666, "Value"=FALSE ("Jump to Analysis")) -> (error out=w1664:errorcluster)  [unwired: 1 in, 1 out]
                    n897 = Initialize Array(0 ("element"), w1667) -> (w1670:i32[])
                    n898 = global write "SW_Globals.vi" "Zones allocation array"(w1670) -> ()
                    n899 = property on="Record start First Call" class="Bool (strict)"(error in=w1664, "Value"=TRUE ("Record start First Call")) -> (error out=w1662:errorcluster)  [unwired: 1 in, 1 out]
                    n900 = property on="Temp file ready" class="Bool (strict)"(error in=w1662, "Value"=FALSE ("Temp file ready")) -> (error out=w1660:errorcluster)  [unwired: 1 in, 1 out]
                    n901 = property on="Save files First Call" class="Bool (strict)"(error in=w1660, "Value"=TRUE ("Save files First Call")) -> (error out=w1659:errorcluster)  [unwired: 1 in, 1 out]
                  }
                }
                n902 = property on="Pane" class="Pane"(error in=w1537) -> (error out=w1536:errorcluster, "Decos[]"=w1538:refnum<vi>[])  [unwired: 1 in, 1 out]
                n903 = Index Array(array=w1538, index=2) -> (element=w1543:refnum<vi>)
                n904 = property on="Running, s" class="DigNum (strict)"() -> ("Value"=w1495:sgl)  [unwired: 2 in, 2 out]
                n905 = property on="Pause, s" class="DigNum (strict)"() -> ("Value"=w1494:sgl)  [unwired: 2 in, 2 out]
                n906 = property on="Stim., s" class="DigNum (strict)"() -> ("Value"=w1493:sgl)  [unwired: 2 in, 2 out]
                n907 = property class="Decor"(reference=w1543, error in=w1536, "Visible"=FALSE) -> (error out=w1535:errorcluster)  [unwired: 1 out]
                n908 = global write "SW_Globals.vi" "Run time pause, s"(w1494) -> ()
                n909 = global write "SW_Globals.vi" "Run time stim, s"(w1493) -> ()
                n910 = global write "SW_Globals.vi" "Run time threshold, s"(w1495) -> ()
                n911 = Index Array(array=w1538, index=1) -> (element=w1540:refnum<vi>)
                n912 = property class="Decor"(reference=w1540, error in=w1535, "Visible"=TRUE) -> (error out=w1534:errorcluster)  [unwired: 1 out]
                n913 = property on="Main tab control" class="TabCtl (strict)"(error in=w1534, "Value"=w1607) -> (error out=w1603:errorcluster, "Pages"=w1608:refnum<vi>[])  [unwired: 1 in, 1 out]
                n914 = To Long Integer(number=w1607) -> (32bit integer=w1606:i32)
                n915 = Index Array(array=w1608, index=w1606) -> (element=w1605:refnum<vi>)
                n916 = property class="Page"(reference=w1605, error in=w1603, "PageEnb"=T28."Page Disabled & Grayed" ("Page Enabled State")) -> (error out=w1596:errorcluster)  [unwired: 1 out]
                n917 = property on="Main tab control" class="TabCtl (strict)"(error in=w1596, "Value"=w1598) -> (error out=w1602:errorcluster, "Pages"=w1597:refnum<vi>[])  [unwired: 1 in, 1 out]
                n918 = To Long Integer(number=w1598) -> (32bit integer=w1599:i32)
                n919 = Index Array(array=w1597, index=w1599) -> (element=w1600:refnum<vi>)
                n920 = property class="Page"(reference=w1600, error in=w1602, "PageEnb"=T28."Page Disabled & Grayed" ("Page Enabled State")) -> (error out=w1589:errorcluster)  [unwired: 1 out]
                n921 = property on="Main tab control" class="TabCtl (strict)"(error in=w1589, "Value"=w1594) -> (error out=w1590:errorcluster, "Pages"=w1595:refnum<vi>[])  [unwired: 1 in, 1 out]
                n922 = To Long Integer(number=w1594) -> (32bit integer=w1593:i32)
                n923 = local read "Settings file refnum out"() -> (w1588:T4)
                n924 = local read "N segments MIDFIELD"() -> (w1586:u8)
                n925 = Index Array(array=w1595, index=w1593) -> (element=w1592:refnum<vi>)
                n926 = local read "Current User"() -> (w1514:string)
                n927 = local read "N segments BORDER"() -> (w1581:u8)
                n928 = property class="Page"(reference=w1592, error in=w1590, "PageEnb"=T28."Page Enabled" ("Page Enabled State")) -> (error out=w1585:errorcluster)  [unwired: 1 out]
                n929 = local read "Radius, mm CENTER"() -> (w1580:u16)
                n930 = call <vilib>:"Write Key (I32).vi"("section"=w1514, "error in (no error)"=w1585, "value"=w1586, "key"="Amount of midfield segments", "refnum"=w1588) -> ("error out"=w1583:errorcluster, "refnum out"=w1582:T4)  [unwired: 4 in, 1 out]
                n931 = local read "Radius, mm MIDFIELD"() -> (w1573:u16)
                n932 = call <vilib>:"Write Key (I32).vi"("section"=w1514, "error in (no error)"=w1583, "value"=w1581, "key"="Amount of border segments", "refnum"=w1582) -> ("error out"=w1577:errorcluster, "refnum out"=w1578:T4)  [unwired: 4 in, 1 out]
                n933 = local read "Starting angle MIDFIELD"() -> (w1572:i16)
                n934 = call <vilib>:"Write Key (I32).vi"("section"=w1514, "error in (no error)"=w1577, "value"=w1580, "key"="Center segment outer radius, mm", "refnum"=w1578) -> ("error out"=w1574:errorcluster, "refnum out"=w1575:T4)  [unwired: 4 in, 1 out]
                n935 = local read "Starting angle BORDER"() -> (w1565:i16)
                n936 = call <vilib>:"Write Key (I32).vi"("section"=w1514, "error in (no error)"=w1574, "value"=w1573, "key"="Midfield segments outer radius, mm", "refnum"=w1575) -> ("error out"=w1569:errorcluster, "refnum out"=w1570:T4)  [unwired: 4 in, 1 out]
                n937 = local read "Cage diameter, mm"() -> (w1545:u16)
                n938 = call <vilib>:"Write Key (I32).vi"("section"=w1514, "error in (no error)"=w1569, "value"=w1572, "key"="Midfield segments starting angle", "refnum"=w1570) -> ("error out"=w1567:errorcluster, "refnum out"=w1566:T4)  [unwired: 4 in, 1 out]
                n939 = call <vilib>:"Write Key (I32).vi"("section"=w1514, "error in (no error)"=w1567, "value"=w1565, "key"="Border segments starting angle", "refnum"=w1566) -> ("error out"=w1564:errorcluster, "refnum out"=w1563:T4)  [unwired: 4 in, 1 out]
                n940 = call <vilib>:"Write Key (I32).vi"("section"=w1514, "error in (no error)"=w1564, "value"=w1545, "key"="Cage diameter, mm", "refnum"=w1563) -> ("error out"=w1498:errorcluster, "refnum out"=w1511:T4)  [unwired: 4 in, 1 out]
                n941 = global read "SW_Globals.vi" "Stimulus presets"() -> (w1501:T42)
                n942 = global read "SW_Globals.vi" "IO parameters cluster"() -> (w1500:T32)
                n943 = for {
                  tunnel: w1501 -> [w1621] mode=indexing
                  tunnel: w1511 -> [w1614]
                  tunnel: [w1618] -> w1517
                  tunnel: w1514 -> [w1612]
                  i -> [w1617]
                  n944 = Unbundle By Name(w1621) -> ("Stim. has been set"=w1619:bool)
                  n945 = Flatten To JSON(anything=w1621) -> (JSON string=w1620:string, 11:w1610:errorcluster)  [unwired: 2 in]
                  n946 = Format Value(string ("")="Zone " ("string"), format string="%02d", value (0)=w1617) -> (output string=w1611:string)
                  n947 = call <vilib>:"Remove Key.vi"("section"=w1612, "error in (no error)"=w1610, "key"=w1611, "refnum"=w1614) -> ("error out"=w1609:errorcluster, "refnum out"=w1613:T4)  [unwired: 5 in, 1 out]
                  n948 = case shown="True" w1619 {
                    tunnel: w1620 -> [_ w1628]
                    tunnel: w1609 -> [_ w1627]
                    tunnel: [w1622 w1626] -> w1618
                    tunnel: w1612 -> [_ w1625]
                    tunnel: w1611 -> [_ w1624]
                    tunnel: w1613 -> [w1622 w1623]
                    frame False {
                    }
                    frame True {
                      n949 = call <vilib>:"Write Key (String).vi"("section"=w1625, "error in (no error)"=w1627, "value"=w1628, "key"=w1624, "refnum"=w1623) -> ("refnum out"=w1626:T4)  [unwired: 4 in, 2 out]
                    }
                  }
                }
                n950 = Cluster To Array(cluster=w1500) -> (array=w1496:u16[])
                n951 = Flatten To JSON(anything=w1496, error in (no error)=w1498) -> (JSON string=w1499:string, 11:w1497:errorcluster)  [unwired: 1 in]
                n952 = local read "Starting angle MIDFIELD"() -> (w1524:i16)
                n953 = local read "Starting angle BORDER"() -> (w1525:i16)
                n954 = local read "N segments MIDFIELD"() -> (w1519:u8)
                n955 = local read "Radius, mm MIDFIELD"() -> (w1523:u16)
                n956 = local read "N segments BORDER"() -> (w1520:u8)
                n957 = local read "Radius, mm CENTER"() -> (w1521:u16)
                n958 = local read "Cage diameter, mm"() -> (w1518:u16)
                n959 = call <vilib>:"Write Key (String).vi"("section"=w1514, "error in (no error)"=w1497, "value"=w1499, "key"="IO ports configuration", "refnum"=w1517) -> ("error out"=w1516:errorcluster, "refnum out"=w1515:T4)  [unwired: 4 in, 1 out]
                n960 = call <vilib>:"Close Config Data.vi"("error in (no error)"=w1516, "refnum"=w1515) -> ("error out"=w1561:errorcluster)  [unwired: 8 in, 1 out]
                n961 = property on="Zones presence indicator" class="Clust"() -> ("Controls[]"=w1558:refnum<vi>[])  [unwired: 2 in, 2 out]
                n962 = property on="Diagram at recording" class="Pict"(error in=w1561) -> ("Bounds"=w1533:T16)  [unwired: 1 in, 2 out]
                n963 = Compound Arithmetic op=ADD(w1520, w1519, u8 1 ("value")) -> (w1554:u8)
                n964 = for {
                  tunnel: w1558 -> [w1637] mode=indexing
                  tunnel: w1554 -> [w1631]
                  tunnel: [w1629] -> w1504
                  i -> [w1636]
                  n965 = Increment(x=w1636) -> (x+1=w1630:i32)
                  n966 = Less Or Equal?(x=w1630, y=w1631) -> (x <= y?=w1635:bool)
                  n967 = Select(t=T10."Disabled" ("Disabled"), s=w1635, f=T10."Disabled and Grayed Out" ("Disabled")) -> (s? t:f=w1633:T10)
                  n968 = property class="Ctl"(reference=w1637, "DisabledEnum"=w1633) -> (error out=w1629:errorcluster)  [unwired: 1 in, 1 out]
                }
                n969 = Bundle By Name(cluster=T17 {"Amount of border segments"=8, "Border segments starting angle"=0, "Amount of midfield segments"=4, "Midfield segments starting angle"=0, "Midfield segments outer radius, mm"=60, "Amount of central segments"=1, "Center segment outer radius, mm"=30, "Diameter of the cage, mm"=180, "R-gap between segments, mm"=10} ("Input cluster of parameters"), "Amount of border segments"=w1520, "Border segments starting angle"=w1525, "Amount of midfield segments"=w1519, "Midfield segments starting angle"=w1524, "Midfield segments outer radius, mm"=w1523, "Amount of central segments"=u8 1, "Center segment outer radius, mm"=w1521, "Diameter of the cage, mm"=w1518) -> (w1526:T17)
                n970 = global write "SW_Globals.vi" "Active segments amount"(w1554) -> ()
                n971 = Increment(x=w1554) -> (x+1=w1553:u8)
                n972 = global read "SW_Globals.vi" "Regions to track"() -> (w1532:u8[])
                n973 = call "SW_Generate_Segmented_Plot_v3.vi"("Draw Area Size"=w1533, "Regions to mark set"=w1532, "Input cluster of parameters"=w1526) -> ("Zones layout output"=w1509:picture, "No zones image"=w1510:picture, "Array of the pixel to color correspondences"=w1528:u32[][], "Array of the segment to color correspondences"=w1531:u32[][], "Cluster of image geometrical and scaling parameters"=w1530:T22)  [unwired: 7 in, 1 out]
                n974 = global write "SW_Globals.vi" "Diagram"(w1509) -> ()
                n975 = local write "Diagram at recording"(w1509) -> ()
                n976 = global write "SW_Globals.vi" "Diagram no zones"(w1510) -> ()
                n977 = global write "SW_Globals.vi" "Array of the pixel to color correspondences"(w1528) -> ()
                n978 = global write "SW_Globals.vi" "Array of the segment to color correspondences"(w1531) -> ()
                n979 = Unbundle By Name(w1530) -> ("Pixels per mm"=→"Pixels per mm":dbl)
                n980 = Bundle By Name(cluster=T18 {"Minimum"=0.0, "Maximum"=14.0, "Increment"=1.0, "Minor Increment"=1.0, "Start"=0.0} ("X Scale.Range"), "Maximum"=w1553) -> (w1555:T18)
                n981 = Array Size(array=w1528) -> (size(s)=w1550:i32[])
                n982 = Index Array(array=w1550, index=0) -> (element=w1549:i32)
                n983 = Index Array(array=w1550, index=1) -> (element=w1548:i32)
                n984 = global write "SW_Globals.vi" "Full track with no zones"(w1510) -> ()
                n985 = global write "SW_Globals.vi" "Full track with zones"(w1509) -> ()
                n986 = Initialize Array(u32 0 ("element"), w1549, w1548) -> (w1546:u32[][])
                n987 = property on="Histograms (normalized)" class="WFGraph (strict)"("XScale.Range"=w1555, "Caption.Text"="Zone preference (normalized)" ("Label.Text"), "XScale.ScaleFit"=u8 2 ("X Scale.Scale Fit"), "XScale.Ofst&Mult"=T26 {"Offset"=1.0, "Multiplier"=0.0} ("X Scale.Offset and Multiplier"), "YScale.Mapping Mode"=u8 0 ("Y Scale.Mapping Mode")) -> ()  [unwired: 2 in, 2 out]
                n988 = global write "SW_Globals.vi" "Array of the presence count"(w1546) -> ()
                n989 = global write "SW_Globals.vi" "Zones presence indicator"(w1503) -> ()
                n990 = property on="Zones presence indicator" class="Clust"(error in=w1504, "Value"=w1503) -> ()  [unwired: 1 in, 2 out]
              }
              frame 2 {
                w1676 = T10."Disabled and Grayed Out" ("Disabled")
                w1677 = FALSE ("Zones an.")
                w1696 = enum32{"Settings", "Recording", "Analysis"}."Analysis" ("Main tab control")
                w1700 = enum32{"Settings", "Recording", "Analysis"}."Recording" ("Main tab control")
                w1709 = enum32{"Settings", "Recording", "Analysis"}."Settings" ("Main tab control")
                n991 = property on="Main tab control" class="TabCtl (strict)"(error in=w1690, "Value"=w1709) -> (error out=w1705:errorcluster, "Pages"=w1710:refnum<vi>[])  [unwired: 1 in, 1 out]
                n992 = To Long Integer(number=w1709) -> (32bit integer=w1708:i32)
                n993 = Index Array(array=w1710, index=w1708) -> (element=w1707:refnum<vi>)
                n994 = property class="Page"(reference=w1707, error in=w1705, "PageEnb"=T28."Page Disabled & Grayed" ("Page Enabled State")) -> (error out=w1698:errorcluster)  [unwired: 1 out]
                n995 = property on="Main tab control" class="TabCtl (strict)"(error in=w1698, "Value"=w1700) -> (error out=w1704:errorcluster, "Pages"=w1699:refnum<vi>[])  [unwired: 1 in, 1 out]
                n996 = To Long Integer(number=w1700) -> (32bit integer=w1701:i32)
                n997 = Index Array(array=w1699, index=w1701) -> (element=w1702:refnum<vi>)
                n998 = property class="Page"(reference=w1702, error in=w1704, "PageEnb"=T28."Page Disabled & Grayed" ("Page Enabled State")) -> (error out=w1691:errorcluster)  [unwired: 1 out]
                n999 = property on="Main tab control" class="TabCtl (strict)"(error in=w1691, "Value"=w1696) -> (error out=w1692:errorcluster, "Pages"=w1697:refnum<vi>[])  [unwired: 1 in, 1 out]
                n1000 = To Long Integer(number=w1696) -> (32bit integer=w1695:i32)
                n1001 = Index Array(array=w1697, index=w1695) -> (element=w1694:refnum<vi>)
                n1002 = property class="Page"(reference=w1694, error in=w1692, "PageEnb"=T28."Page Enabled" ("Page Enabled State")) -> (error out=w1689:errorcluster)  [unwired: 1 out]
                n1003 = property on="Zones (analysis)" class="Bool (strict)"(error in=w1689, "Value"=w1677, "DisabledEnum"=w1676) -> (error out=w1688:errorcluster)  [unwired: 1 in, 1 out]
                n1004 = property on="Play/Pause" class="Bool (strict)"(error in=w1688, "DisabledEnum"=w1676) -> (error out=w1687:errorcluster)  [unwired: 1 in, 1 out]
                n1005 = property on="Show heatmap (analysis)" class="Bool (strict)"("DisabledEnum"=w1676, "Value"=w1677) -> ()  [unwired: 2 in, 2 out]
                n1006 = property on="Show full track (analysis)" class="Bool (strict)"("DisabledEnum"=w1676, "Value"=w1677) -> ()  [unwired: 2 in, 2 out]
                n1007 = property on="Back to Settings" class="Bool (strict)"(error in=w1687, "Visible"=TRUE, "Value"=FALSE ("Back to Settings")) -> (error out=w1682:errorcluster)  [unwired: 1 in, 1 out]
                n1008 = property on="Pane" class="Pane"(error in=w1682) -> (error out=w1675:errorcluster, "Decos[]"=w1678:refnum<vi>[])  [unwired: 1 in, 1 out]
                n1009 = property on="Map index (analysis)" class="DigNum (strict)"(error in=w1675, "Value"=0 ("Map index (analysis)")) -> (error out=w1672:errorcluster)  [unwired: 1 in, 1 out]
                n1010 = Index Array(array=w1678, index=0) -> (element=w1680:refnum<vi>)
                n1011 = Index Array(array=w1678, index=2) -> (element=w1684:refnum<vi>)
                n1012 = property class="Decor"(reference=w1680, "Visible"=TRUE) -> ()  [unwired: 1 in, 2 out]
                n1013 = property class="Decor"(reference=w1684, "Visible"=FALSE) -> ()  [unwired: 1 in, 2 out]
                n1014 = property on="Jump to Analysis" class="Bool (strict)"(error in=w1672, "Value"=FALSE ("Jump to Analysis")) -> ()  [unwired: 1 in, 2 out]
              }
            }
          }
        }
      }
      frame "Recording" {
        w1748 = FALSE ("use system decimal point (T)")
        n1015 = call <extravilib>:"Read.vi"("channel"=w1772) -> ("element"=w1742:string[][])  [unwired: 5 in, 5 out]
        n1016 = Divide(x=u32 1000, y=w1784) -> (x/y=w1783:dbl)
        n1017 = call "FL_Last_N_Samples_2D_array_of_strings.vi"("BufferLengthSamples"=u32 5, "Input Array of strings"=w1742) -> ("Output Array of strings"=w1741:string[][])
        n1018 = Multiply(x=w1783, y="Trace, s") -> (x*y=w1787:dbl)
        n1019 = Array Size(array=w1741) -> (size(s)=w1764:i32[])
        n1020 = Index Array(array=w1764, index=0) -> (element=w1762:i32)
        n1021 = Decrement(x=w1762) -> (x-1=w1761:i32)
        n1022 = Round To Nearest(number=w1787) -> (nearest integer value=w1786:dbl)
        n1023 = First Call?() -> (First Call?: T/F=w1725:bool)
        n1024 = Index Array(array=w1741, index (row)=w1761) -> (element=w1753:string[])  [unwired: 1 in]
        n1025 = case shown="True" w1725 {
          frame False {
          }
          frame True {
            n1026 = property on="Type of histogram" class="DigNum (strict)"("Val(Sgnl)"=u8 2 ("Value (Signaling)")) -> ()  [unwired: 2 in, 2 out]
          }
        }
        n1027 = global read "SW_Globals.vi" "Diagram no zones"() -> (w1793:picture)
        n1028 = Index Array "w (mouse rot. angle)"(array=w1753, index=8) -> (element=w1749:string)
        n1029 = Index Array "X (filtered)"(array=w1753, index=9) -> (element=w1751:string)
        n1030 = Index Array "Y (filtered)"(array=w1753, index=10) -> (element=w1750:string)
        n1031 = Index Array "Timestamp"(array=w1753, index=4) -> (element=w1759:string)
        n1032 = global read "SW_Globals.vi" "Diagram"() -> (w1794:picture)
        n1033 = Select(t=w1794, s="Zones", f=w1793) -> (s? t:f=w1795:picture)
        n1034 = Not(x="Zones") -> (.not. x?=w1789:bool)
        n1035 = String Length(string=w1759) -> (length=w1758:i32)
        n1036 = Fract/Exp String To Number(use system decimal point (T)=w1748, string=w1749) -> (number=w1747:dbl)  [unwired: 2 in, 1 out]
        n1037 = Fract/Exp String To Number(use system decimal point (T)=w1748, string=w1751) -> (number=w1745:dbl)  [unwired: 2 in, 1 out]
        n1038 = Fract/Exp String To Number(use system decimal point (T)=w1748, string=w1750) -> (number=w1744:dbl)  [unwired: 2 in, 1 out]
        n1039 = property on="Diagram at recording" class="Pict"() -> ("Bounds"=w1791:T16)  [unwired: 2 in, 2 out]
        n1040 = local read "Pixels per mm"() -> (w1792:dbl)
        n1041 = Greater Than 0?(x=w1758) -> (x > 0?=w1757:bool)
        n1042 = event shown="[2] \"Histograms (normalized)\": Mouse Down;  \"Type of histogram\": Value Change" {
          selector: _ -> [_ _ _]
          dyn-events: _ -> [_ _ _]
          timeout: 0 -> [_ _ _]
          tunnel: "Type of histogram" -> [_ _ w1835]
          event Timeout {
            n1043 = event-data() -> ()  [unwired: 1 in, 3 out]
          }
          event "Multiplyer of chart RX": Value Change {
            n1044 = event-data() -> ("NewVal"=w1826:u8)  [unwired: 1 in, 5 out]
            n1045 = Multiply(x=w1826, y=10.0) -> (x*y=w1827:dbl)
            n1046 = property on="Mouse speed" class="WFChart (strict)"() -> (error out=w1828:errorcluster, "XScale.Maximum"=w1831:dbl)  [unwired: 2 in, 1 out]
            n1047 = Subtract(x=w1831, y=w1827) -> (x-y=w1829:dbl)
            n1048 = property on="Mouse speed" class="WFChart (strict)"(error in=w1828, "XScale.Minimum"=w1829) -> ()  [unwired: 1 in, 2 out]
          }
          event "Histograms (normalized)": Mouse Down; "Type of histogram": Value Change {
            n1049 = event-data() -> ()  [unwired: 1 in, 4 out]
            n1050 = Increment(x=w1835) -> (x+1=w1832:u8)
            n1051 = Quotient & Remainder(x=w1832, y=u8 4) -> (x-y*floor(x/y)=w1833:u8)  [unwired: 1 out]
            n1052 = property on="Type of histogram" class="DigNum (strict)"("Value"=w1833) -> ()  [unwired: 2 in, 2 out]
            n1053 = case shown="1" w1833 {
              frame 0, Default {
                w1836 = FALSE ("Speed distrib. indicator")
                # "Show zones preference"
                n1054 = global read "SW_Globals.vi" "Active segments amount"() -> (w1849:u8)
                n1055 = Wait (ms)(milliseconds to wait=u32 100) -> ()  [unwired: 1 out]
                n1056 = Increment(x=w1849) -> (x+1=w1848:u8)
                n1057 = global read "SW_Globals.vi" "Zones normalized allocation array"() -> (w1842:dbl[])
                n1058 = Bundle By Name(cluster=T18 {"Minimum"=0.0, "Maximum"=14.0, "Increment"=1.0, "Minor Increment"=1.0, "Start"=0.0} ("X Scale.Range"), "Maximum"=w1848) -> (w1850:T18)
                n1059 = property on="Histograms (normalized)" class="WFGraph (strict)"("XScale.Range"=w1850, "Caption.Text"="Zone preference (normalized)" ("Label.Text"), "XScale.Multiplier"=1.0 ("X Scale.Offset and Multiplier:Multiplier"), "XScale.Offset"=0.0 ("X Scale.Offset and Multiplier:Offset"), "XScale.ScaleFit"=u8 2 ("X Scale.Scale Fit"), "YScale.Mapping Mode"=u8 0 ("Y Scale.Mapping Mode"), "Value"=w1842, "Plot.Fill/Pt. Color"=u32 15790320 ("Plot.Fill/Point Color"), "XScale.ScaleFit"=u8 1 ("X Scale.Scale Fit"), "XScale.Precision"=u8 0 ("X Scale.Display Format:Precision")) -> ()  [unwired: 2 in, 2 out]
                n1060 = property on="Zones presense indicator" class="Bool (strict)"("Value"=TRUE ("Zones presense indicator")) -> ()  [unwired: 2 in, 2 out]
                n1061 = property on="Speed distrib. indicator" class="Bool (strict)"("Value"=w1836) -> ()  [unwired: 2 in, 2 out]
                n1062 = property on="Run lengts distrib. indicator" class="Bool (strict)"("Value"=w1836) -> ()  [unwired: 2 in, 2 out]
                n1063 = property on="Run times distrib. indicator" class="Bool (strict)"("Value"=w1836) -> ()  [unwired: 2 in, 2 out]
              }
              frame 1 {
                w1852 = FALSE ("Zones presense indicator")
                # "Speed distribution"
                n1064 = global read "SW_Globals.vi" "Speed bins array"() -> (w1865:dbl[])
                n1065 = Wait (ms)(milliseconds to wait=u32 100) -> ()  [unwired: 1 out]
                n1066 = Array Size(array=w1865) -> (size(s)=w1867:i32)
                n1067 = global read "SW_Globals.vi" "Speed distribution array"() -> (w1858:u32[])
                n1068 = Decrement(x=w1867) -> (x-1=w1861:i32)
                n1069 = property on="Histograms (normalized)" class="WFGraph (strict)"("XScale.ScaleFit"=u8 0 ("X Scale.Scale Fit")) -> (error out=w1860:errorcluster)  [unwired: 2 in, 1 out]
                n1070 = Bundle By Name(cluster=T18 {"Minimum"=0.0, "Maximum"=14.0, "Increment"=1.0, "Minor Increment"=1.0, "Start"=0.0} ("X Scale.Range"), "Maximum"=w1861) -> (w1868:T18)
                n1071 = call "SW_Get_1D_Array_normalize.vi"("1D array"=w1858) -> ("Normalized 1D array"=w1857:dbl[])  [unwired: 2 in, 1 out]
                n1072 = property on="Histograms (normalized)" class="WFGraph (strict)"(error in=w1860, "XScale.Range"=w1868, "Caption.Text"="Speed histogram (normalized)" ("Label.Text"), "XScale.Multiplier"=36.5 ("X Scale.Offset and Multiplier:Multiplier 2"), "XScale.Offset"=0 ("index"), "YScale.Mapping Mode"=u8 1 ("X Scale.Scale Fit"), "Value"=w1857, "Plot.Fill/Pt. Color"=u32 16777120 ("Plot.Fill/Point Color"), "XScale.ScaleFit"=u8 0 ("X Scale.Scale Fit")) -> ()  [unwired: 1 in, 2 out]
                n1073 = property on="Zones presense indicator" class="Bool (strict)"("Value"=w1852) -> ()  [unwired: 2 in, 2 out]
                n1074 = property on="Speed distrib. indicator" class="Bool (strict)"("Value"=TRUE ("Speed distrib. indicator")) -> ()  [unwired: 2 in, 2 out]
                n1075 = property on="Run lengts distrib. indicator" class="Bool (strict)"("Value"=w1852) -> ()  [unwired: 2 in, 2 out]
                n1076 = property on="Run times distrib. indicator" class="Bool (strict)"("Value"=w1852) -> ()  [unwired: 2 in, 2 out]
              }
              frame 2 {
                w1870 = FALSE ("Zones presense indicator")
                # "Runing bout distribution"
                n1077 = global read "SW_Globals.vi" "Run Lengths bins array"() -> (w1876:dbl[])
                n1078 = Wait (ms)(milliseconds to wait=u32 100) -> ()  [unwired: 1 out]
                n1079 = Array Size(array=w1876) -> (size(s)=w1890:i32)
                n1080 = global read "SW_Globals.vi" "Run Lengts distribution array"() -> (w1883:u32[])
                n1081 = Decrement(x=w1890) -> (x-1=w1871:i32)
                n1082 = Array Subset(array=w1876, index=0, length=w1871) -> ()  [unwired: 1 out]
                n1083 = property on="Histograms (normalized)" class="WFGraph (strict)"("XScale.ScaleFit"=u8 0 ("X Scale.Scale Fit")) -> (error out=w1885:errorcluster)  [unwired: 2 in, 1 out]
                n1084 = Bundle By Name(cluster=T18 {"Minimum"=0.0, "Maximum"=2.0, "Increment"=0.2, "Minor Increment"=0.2, "Start"=0.0} ("X Scale.Range"), "Maximum"=w1871) -> (w1872:T18)
                n1085 = call "SW_Get_1D_Array_normalize.vi"("1D array"=w1883) -> ("Normalized 1D array"=w1882:dbl[])  [unwired: 2 in, 1 out]
                n1086 = property on="Histograms (normalized)" class="WFGraph (strict)"(error in=w1885, "XScale.Range"=w1872, "Caption.Text"="Running bout dist. hist. (norm.)" ("Label.Text"), "XScale.Multiplier"=0.2 ("X Scale.Offset and Multiplier:Multiplier 2"), "XScale.Offset"=0.2 ("index"), "YScale.Mapping Mode"=u8 0 ("X Scale.Scale Fit"), "Value"=w1882, "Plot.Fill/Pt. Color"=u32 12320699 ("Plot.Fill/Point Color"), "XScale.ScaleFit"=u8 1 ("X Scale.Scale Fit"), "XScale.Format"=u8 0 ("X Scale.Display Format:Format"), "XScale.Precision"=u8 1 ("X Scale.Display Format:Precision")) -> ()  [unwired: 1 in, 2 out]
                n1087 = property on="Zones presense indicator" class="Bool (strict)"("Value"=w1870) -> ()  [unwired: 2 in, 2 out]
                n1088 = property on="Speed distrib. indicator" class="Bool (strict)"("Value"=w1870) -> ()  [unwired: 2 in, 2 out]
                n1089 = property on="Run lengts distrib. indicator" class="Bool (strict)"("Value"=TRUE ("Speed distrib. indicator")) -> ()  [unwired: 2 in, 2 out]
                n1090 = property on="Run times distrib. indicator" class="Bool (strict)"("Value"=w1870) -> ()  [unwired: 2 in, 2 out]
              }
              frame 3 {
                w1891 = FALSE ("Zones presense indicator")
                # "Running times distribution"
                n1091 = global read "SW_Globals.vi" "Run Times bins array"() -> (w1898:dbl[])
                n1092 = Wait (ms)(milliseconds to wait=u32 100) -> ()  [unwired: 1 out]
                n1093 = Array Size(array=w1898) -> (size(s)=w1911:i32)
                n1094 = global read "SW_Globals.vi" "Run Times distribution array"() -> (w1904:u32[])
                n1095 = Decrement(x=w1911) -> (x-1=w1893:i32)
                n1096 = Array Subset(array=w1898, index=0, length=w1893) -> ()  [unwired: 1 out]
                n1097 = property on="Histograms (normalized)" class="WFGraph (strict)"("XScale.ScaleFit"=u8 0 ("X Scale.Scale Fit")) -> (error out=w1906:errorcluster)  [unwired: 2 in, 1 out]
                n1098 = Bundle By Name(cluster=T18 {"Minimum"=0.0, "Maximum"=2.0, "Increment"=0.2, "Minor Increment"=0.2, "Start"=0.0} ("X Scale.Range"), "Maximum"=w1893) -> (w1894:T18)
                n1099 = call "SW_Get_1D_Array_normalize.vi"("1D array"=w1904) -> ("Normalized 1D array"=w1903:dbl[])  [unwired: 2 in, 1 out]
                n1100 = property on="Histograms (normalized)" class="WFGraph (strict)"(error in=w1906, "XScale.Range"=w1894, "Caption.Text"="Run times dist. hist. (norm.)" ("Label.Text"), "XScale.Multiplier"=1.0 ("X Scale.Offset and Multiplier:Multiplier 2"), "XScale.Offset"=0.5 ("index"), "YScale.Mapping Mode"=u8 0 ("X Scale.Scale Fit"), "Value"=w1903, "Plot.Fill/Pt. Color"=u32 16771022 ("Plot.Fill/Point Color"), "XScale.ScaleFit"=u8 1 ("X Scale.Scale Fit"), "XScale.Format"=u8 0 ("X Scale.Display Format:Format"), "XScale.Precision"=u8 1 ("X Scale.Display Format:Precision")) -> ()  [unwired: 1 in, 2 out]
                n1101 = property on="Zones presense indicator" class="Bool (strict)"("Value"=w1891) -> ()  [unwired: 2 in, 2 out]
                n1102 = property on="Speed distrib. indicator" class="Bool (strict)"("Value"=w1891) -> ()  [unwired: 2 in, 2 out]
                n1103 = property on="Run lengts distrib. indicator" class="Bool (strict)"("Value"=w1891) -> ()  [unwired: 2 in, 2 out]
                n1104 = property on="Run times distrib. indicator" class="Bool (strict)"("Value"=TRUE ("Run times distrib. indicator")) -> ()  [unwired: 2 in, 2 out]
              }
            }
          }
        }
        n1105 = call "SW_Draw_mouse_br.vi"("Input picture (background)"=w1795, "Size of the image"=w1791, "Pixels per mm"=w1792, "Mouse coord cartesian X, mm"=w1745, "Mouse coord cartesian Y, mm"=w1744, "Mouse angle of rotation, deg"=w1747, "Show mouse lineout"=w1789, "Trace length, samples"=w1786) -> ("Output picture (with mouse overlay)"=→"Diagram at recording":picture)  [unwired: 6 in, 1 out]
        n1106 = case shown="True" w1757 {
          tunnel: [w1804 w1807] -> w1756
          tunnel: w1759 -> [_ w1806]
          frame False {
            n1107 = Get Date/Time In Seconds() -> (seconds since 1Jan1904=w1804:timestamp)
          }
          frame True {
            (unwired) "%<%H:%M:%S%3u%p%d.%m.%Y>T" ("format string")
            n1108 = Get Date/Time In Seconds() -> (seconds since 1Jan1904=w1805:timestamp)
            n1109 = Scan From String(format string="%<%H:%M:%S%,;%3u %d.%m.%Y>T", input string=w1806, default 1=w1805) -> (output 1=w1807:timestamp)  [unwired: 2 in, 3 out]
          }
        }
        n1110 = Tick Count (ms)() -> (millisecond timer value=w1781:u32)
        n1111 = global read "SW_Globals.vi" "Run Lengts distribution array"() -> (w1718:u32[])
        n1112 = global read "SW_Globals.vi" "Run Times distribution array"() -> (w1715:u32[])
        n1113 = global read "SW_Globals.vi" "Run Lengths bins array"() -> (w1717:dbl[])
        n1114 = global read "SW_Globals.vi" "Speed distribution array"() -> (w1734:u32[])
        n1115 = global read "SW_Globals.vi" "Speed bins array"() -> (w1738:dbl[])
        n1116 = global read "SW_Globals.vi" "Run Times bins array"() -> (w1714:dbl[])
        n1117 = property on="Type of histogram" class="DigNum (strict)"() -> ("Value"=w1721:u8)  [unwired: 2 in, 2 out]
        n1118 = Not(x="Exit (recording)") -> (.not. x?=w1767:bool)
        n1119 = property on="Current Time" class="AbsTime (strict)"("Value"=w1756) -> ()  [unwired: 2 in, 2 out]
        n1120 = global read "SW_Globals.vi" "Zones presence indicator"() -> (w1740:T41)
        n1121 = And(x=w1767, y="Record/Stop") -> (x .and. y?=w1768:bool)
        n1122 = property on="Zones presence indicator" class="Clust"("Value"=w1740) -> ()  [unwired: 2 in, 2 out]
        n1123 = case shown="False" w1768 {
          tunnel: w1770 -> [w1914 w2009]
          tunnel: w1756 -> [_ w2007]
          tunnel: [w1917 w2008] -> _
          tunnel: w1782 -> [_ w2006]
          tunnel: [w1916 w2004] -> w1774
          tunnel: "Exit (recording)" -> [w1913 _]
          frame False {
            n1124 = Unbundle By Name(w1914) -> ("Has been recorded"=w1919:refnum<notifier>)
            n1125 = Get Notifier Status(notifier=w1919) -> (current notification=w1912:bool, error out=w1918:errorcluster)  [unwired: 1 in, 3 out]
            n1126 = Or(x=w1913, y=w1912) -> (x .or. y?=w1915:bool)
            n1127 = case shown="True" w1915 {
              tunnel: w1914 -> [_ w1992]
              tunnel: w1918 -> [_ w1971]
              tunnel: [w1930 w1965] -> w1917
              tunnel: [FALSE FALSE] -> w1916
              tunnel: w1912 -> [_ w1934]
              frame False {
                n1128 = global read "SW_Globals.vi" "Cluster of paths"() -> (w1931:T19)
                n1129 = Unbundle By Name(w1931) -> ("Temporary file output path"=w1930:path, "Path to the settings file"=w1921:path)
                n1130 = local read "Current User"() -> (w1920:string)
                n1131 = property on="Bridge swap" class="Bool (strict)" props=["Value"]() -> (error out=w1922:errorcluster)  [unwired: 2 in, 2 out]
                n1132 = call <vilib>:"Open Config Data.vi"("error in (no error)"=w1922, "create file if necessary (T)"=FALSE, "configuration file path"=w1921) -> ("error out"=w1926:errorcluster, "refnum"=w1928:T4)  [unwired: 6 in, 1 out]
                n1133 = call <vilib>:"Write Key (Boolean).vi"("section"=w1920, "error in (no error)"=w1926, "key"="Mouse snout orientation swap?", "refnum"=w1928) -> ("error out"=w1925:errorcluster, "refnum out"=w1927:T4)  [unwired: 5 in, 1 out]
                n1134 = call <vilib>:"Close Config Data.vi"("error in (no error)"=w1925, "refnum"=w1927) -> ()  [unwired: 8 in, 2 out]
              }
              frame True {
                w1936 = FALSE ("Show heatmap (analysis)")
                w1977 = enum32{"Settings", "Recording", "Analysis"}."Analysis" ("Main tab control")
                w1981 = enum32{"Settings", "Recording", "Analysis"}."Recording" ("Main tab control")
                w1990 = enum32{"Settings", "Recording", "Analysis"}."Settings" ("Main tab control")
                n1135 = flat-sequence {
                  tunnel: w1992 -> [w2000]
                  tunnel: w1971 -> [w1996]
                  tunnel: [w1993] -> w1970
                  tunnel: [w2002] -> w1969
                  tunnel: w1970 -> [w2002]
                  frame #0 {
                    n1136 = Unbundle By Name(w2000) -> ("Play/Pause status"=w2001:refnum<notifier>, "Recording now"=w1998:refnum<notifier>)
                    n1137 = Send Notification(notification=FALSE, notifier=w1998, error in (no error)=w1996) -> (error out=w1994:errorcluster)  [unwired: 1 out]
                    n1138 = Send Notification(notification="Pause" ("f"), notifier=w2001) -> (error out=w1995:errorcluster)  [unwired: 1 in, 1 out]
                    n1139 = Merge Errors(w1995, w1994) -> (w1993:errorcluster)
                  }
                  frame #1 {
                    n1140 = Wait (ms)(milliseconds to wait=u32 500) -> ()  [unwired: 1 out]
                  }
                }
                n1141 = property on="Exit (recording)" class="Bool"(error in=w1969, "DisabledEnum"=T10."Enabled" ("Disabled")) -> (error out=w1968:errorcluster)  [unwired: 1 in, 1 out]
                n1142 = property on="Main tab control" class="TabCtl (strict)"(error in=w1968, "Value"=w1990) -> (error out=w1986:errorcluster, "Pages"=w1991:refnum<vi>[])  [unwired: 1 in, 1 out]
                n1143 = To Long Integer(number=w1990) -> (32bit integer=w1989:i32)
                n1144 = Index Array(array=w1991, index=w1989) -> (element=w1988:refnum<vi>)
                n1145 = property class="Page"(reference=w1988, error in=w1986, "PageEnb"=T28."Page Disabled & Grayed" ("Page Enabled State")) -> (error out=w1979:errorcluster)  [unwired: 1 out]
                n1146 = property on="Main tab control" class="TabCtl (strict)"(error in=w1979, "Value"=w1981) -> (error out=w1985:errorcluster, "Pages"=w1980:refnum<vi>[])  [unwired: 1 in, 1 out]
                n1147 = To Long Integer(number=w1981) -> (32bit integer=w1982:i32)
                n1148 = Index Array(array=w1980, index=w1982) -> (element=w1983:refnum<vi>)
                n1149 = property class="Page"(reference=w1983, error in=w1985, "PageEnb"=T28."Page Disabled & Grayed" ("Page Enabled State")) -> (error out=w1972:errorcluster)  [unwired: 1 out]
                n1150 = property on="Main tab control" class="TabCtl (strict)"(error in=w1972, "Value"=w1977) -> (error out=w1973:errorcluster, "Pages"=w1978:refnum<vi>[])  [unwired: 1 in, 1 out]
                n1151 = To Long Integer(number=w1977) -> (32bit integer=w1976:i32)
                n1152 = Index Array(array=w1978, index=w1976) -> (element=w1975:refnum<vi>)
                n1153 = property class="Page"(reference=w1975, error in=w1973, "PageEnb"=T28."Page Enabled" ("Page Enabled State")) -> (error out=w1944:errorcluster)  [unwired: 1 out]
                n1154 = property on="Pane" class="Pane"(error in=w1944) -> (error out=w1943:errorcluster, "Decos[]"=w1945:refnum<vi>[])  [unwired: 1 in, 1 out]
                n1155 = Index Array(array=w1945, index=1) -> (element=w1950:refnum<vi>)
                n1156 = property class="Decor"(reference=w1950, error in=w1943, "Visible"=FALSE) -> (error out=w1942:errorcluster)  [unwired: 1 out]
                n1157 = Index Array(array=w1945, index=0) -> (element=w1947:refnum<vi>)
                n1158 = property class="Decor"(reference=w1947, error in=w1942, "Visible"=TRUE) -> (error out=w1941:errorcluster)  [unwired: 1 out]
                n1159 = Select(t=T10."Enabled" ("Disabled"), s=w1934, f=T10."Disabled and Grayed Out" ("Disabled")) -> (s? t:f=w1933:T10)
                n1160 = global read "SW_Globals.vi" "Cluster of paths"() -> (w1966:T19)
                n1161 = property on="Back to Settings" class="Bool (strict)"(error in=w1941, "Visible"=TRUE) -> (error out=w1953:errorcluster)  [unwired: 1 in, 1 out]
                n1162 = Unbundle By Name(w1966) -> ("Temporary file output path"=w1965:path, "Path to the settings file"=w1959:path)
                n1163 = property on="Bridge swap" class="Bool (strict)"(error in=w1953) -> (error out=w1956:errorcluster, "Value"=w1955:bool)  [unwired: 1 in, 1 out]
                n1164 = local read "Current User"() -> (w1954:string)
                n1165 = call <vilib>:"Open Config Data.vi"("error in (no error)"=w1956, "create file if necessary (T)"=FALSE, "configuration file path"=w1959) -> ("error out"=w1961:errorcluster, "refnum"=w1963:T4)  [unwired: 6 in, 1 out]
                n1166 = call <vilib>:"Write Key (Boolean).vi"("section"=w1954, "error in (no error)"=w1961, "value"=w1955, "key"="Mouse snout orientation swap?", "refnum"=w1963) -> ("error out"=w1960:errorcluster, "refnum out"=w1962:T4)  [unwired: 4 in, 1 out]
                n1167 = call <vilib>:"Close Config Data.vi"("error in (no error)"=w1960, "refnum"=w1962) -> ("error out"=w1939:errorcluster)  [unwired: 8 in, 1 out]
                n1168 = property on="Show heatmap (analysis)" class="Bool (strict)"(error in=w1939, "Value"=w1936, "DisabledEnum"=w1933) -> (error out=w1938:errorcluster)  [unwired: 1 in, 1 out]
                n1169 = property on="Show full track (analysis)" class="Bool (strict)"(error in=w1938, "Value"=w1936, "DisabledEnum"=w1933) -> (error out=w1937:errorcluster)  [unwired: 1 in, 1 out]
                n1170 = property on="Map index (analysis)" class="DigNum (strict)"(error in=w1937, "Value"=0 ("Map index (analysis)")) -> ()  [unwired: 1 in, 2 out]
              }
            }
          }
          frame True {
            n1171 = flat-sequence {
              tunnel: w2007 -> [w2014]
              tunnel: [w2022] -> w2010
              tunnel: w2009 -> [w2019]
              tunnel: [w2017] -> w2008
              tunnel: w2007 -> [w2016]
              tunnel: [w2016] -> w2005
              tunnel: w2006 -> [w2015]
              tunnel: [w2013] -> w2004
              frame #0 {
                n1172 = case shown="True" "Record start First Call" {
                  tunnel: w2014 -> [_ w2047]
                  tunnel: [w2030 w2047] -> w2022
                  tunnel: [w2028 w2045] -> w2017
                  tunnel: [_ w2036] -> w2018
                  tunnel: w2015 -> [_ w2044]
                  tunnel: [FALSE TRUE] -> w2013
                  frame False {
                    n1173 = global read "SW_Globals.vi" "Cluster of paths"() -> (w2029:T19)
                    n1174 = global read "SW_Globals.vi" "Recording start timestamp"() -> (w2030:timestamp)
                    n1175 = Unbundle By Name(w2029) -> ("Temporary file output path"=w2028:path)
                  }
                  frame True {
                    w2035 = T10."Disabled and Grayed Out" ("Disabled")
                    n1176 = property on="Record start First Call" class="Bool (strict)"("Value"=FALSE ("Record start First Call")) -> ()  [unwired: 2 in, 2 out]
                    n1177 = global read "SW_Globals.vi" "Cluster of paths"() -> (w2038:T19)
                    n1178 = Flush Queue(queue=w2044) -> (error out=w2042:errorcluster)  [unwired: 1 in, 2 out]
                    n1179 = call "SW_Get_save_paths.vi"("Input cluster of paths"=w2038) -> ("error out"=w2041:errorcluster, "Output cluster of paths"=w2046:T43)  [unwired: 3 in, 1 out]
                    n1180 = global write "SW_Globals.vi" "Cluster of paths"(w2046) -> ()
                    n1181 = Unbundle By Name(w2046) -> ("Temporary file output path"=w2045:path)
                    n1182 = Merge Errors(w2042, w2041) -> (w2034:errorcluster)
                    n1183 = property on="Data filtering" class="Ring (strict)"(error in=w2034, "DisabledEnum"=T10."Disabled and Grayed Out" ("Disabled")) -> (error out=w2033:errorcluster)  [unwired: 1 in, 1 out]
                    n1184 = property on="Exit (recording)" class="Bool"(error in=w2033, "DisabledEnum"=T10."Enabled" ("Disabled")) -> (error out=w2040:errorcluster)  [unwired: 1 in, 1 out]
                    n1185 = property on="Bridge swap" class="Bool (strict)"(error in=w2040, "DisabledEnum"=w2035) -> (error out=w2037:errorcluster)  [unwired: 1 in, 1 out]
                    n1186 = property on="Vertical offset" class="DigNum (strict)"(error in=w2037, "DisabledEnum"=w2035) -> (error out=w2036:errorcluster)  [unwired: 1 in, 1 out]
                  }
                }
                n1187 = Unbundle By Name(w2019) -> ("Recording now"=w2021:refnum<notifier>, "Has been recorded"=w2026:refnum<notifier>)
                n1188 = Send Notification(notification=TRUE, notifier=w2021, error in (no error)=w2018) -> ()  [unwired: 2 out]
                n1189 = Send Notification(notification=TRUE, notifier=w2026, error in (no error)=w2018) -> (error out=w2023:errorcluster)  [unwired: 1 out]
                n1190 = property on="Record timestamp" class="DigNum (strict)"(error in=w2023, "DisabledEnum"=T10."Enabled" ("Disabled")) -> ()  [unwired: 1 in, 2 out]
              }
            }
            n1191 = Subtract(x=w2005, y=w2010) -> (x-y=→"Record timestamp":dbl)
          }
        }
        n1192 = case shown="True" w1774 {
          frame False {
          }
          frame True {
            w1809 = waveform(dbl)[] [] ("History Data")
            n1193 = property on="Mouse speed" class="WFChart (strict)"("History Data"=w1809) -> ()  [unwired: 2 in, 2 out]
            n1194 = property on="Mouse speed 2" class="WFChart (strict)"("History Data"=w1809) -> ()  [unwired: 2 in, 2 out]
          }
        }
        n1195 = Or(x="Reset barplot", y=w1774) -> (x .or. y?=w1775:bool)
        n1196 = case shown="True" w1775 {
          frame False {
          }
          frame True {
            n1197 = global read "SW_Globals.vi" "Run Lengts distribution array"() -> (w1817:u32[])
            n1198 = global read "SW_Globals.vi" "Run Times distribution array"() -> (w1810:u32[])
            n1199 = global read "SW_Globals.vi" "Speed distribution array"() -> (w1820:u32[])
            n1200 = global read "SW_Globals.vi" "Zones allocation array"() -> (w1823:i32[])
            n1201 = Array Size(array=w1817) -> (size(s)=w1816:i32)
            n1202 = Array Size(array=w1820) -> (size(s)=w1818:i32)
            n1203 = Array Size(array=w1823) -> (size(s)=w1825:i32)
            n1204 = Array Size(array=w1810) -> (size(s)=w1811:i32)
            n1205 = Initialize Array(u32 0 ("element"), w1816) -> (w1814:u32[])
            n1206 = Initialize Array(u32 0 ("element"), w1818) -> (w1821:u32[])
            n1207 = Initialize Array(0 ("element"), w1825) -> (w1822:i32[])
            n1208 = Initialize Array(u32 0 ("element"), w1811) -> (w1813:u32[])
            n1209 = global write "SW_Globals.vi" "Run Lengts distribution array"(w1814) -> ()
            n1210 = global write "SW_Globals.vi" "Speed distribution array"(w1821) -> ()
            n1211 = global write "SW_Globals.vi" "Run Times distribution array"(w1813) -> ()
            n1212 = global write "SW_Globals.vi" "Zones allocation array"(w1822) -> ()
          }
        }
        n1213 = feedback-in #8(w1781) -> ()
        n1214 = feedback #8(w1779) -> (w1780:u32)
        n1215 = Subtract(x=w1781, y=w1780) -> (x-y=w1778:u32)
        n1216 = Divide(x=w1778, y=u32 1000) -> (x/y=w1773:dbl)
        n1217 = call "FL_Calc_speed_on_the_fly.vi"("Y coord, mm"=w1744, "X coord, mm"=w1745, "Time per frame, s"=w1773) -> ("Mouse speed, mm/s"=w1720:dbl)
        "Mouse speed digi" <- w1720
        n1218 = call "FL_Get_Histogram_Bin_number.vi"("Current value"=w1720, "Bins array"=w1738) -> ("Bin assignment"=w1737:i32)
        n1219 = Index Array(array=w1734, index=w1737) -> (element=w1736:u32)
        n1220 = Increment(x=w1736) -> (x+1=w1735:u32)
        n1221 = Replace Array Subset(array=w1734, new element=w1735, index=w1737) -> (w1733:u32[])
        n1222 = call "SW_Get_1D_Array_normalize.vi"("1D array"=w1733) -> ("Normalized 1D array"=w1723:dbl[])  [unwired: 2 in, 1 out]
        n1223 = call "FL_Get_Run_Bout_and_Time.vi"("Speed, mm/s"=w1720, "Run Lengts distribution array in"=w1718, "Run times distribution array in"=w1715, "Run Lengths bin array"=w1717, "Run times bin array"=w1714) -> ("Run Lengts distribution array out"=w1716:u32[], "Run time, s"=w1711:dbl, "Run times distribution array out"=w1713:u32[])  [unwired: 2 in]
        n1224 = Delete From Array(array=w1723, length=1, index=0) -> (array with subset deleted=w1730:dbl[])  [unwired: 1 out]
        n1225 = global write "SW_Globals.vi" "Run Lengts distribution array"(w1716) -> ()
        n1226 = global write "SW_Globals.vi" "Speed distribution array"(w1733) -> ()
        n1227 = global write "SW_Globals.vi" "Run time, s"(w1711) -> ()
        n1228 = global write "SW_Globals.vi" "Run Times distribution array"(w1713) -> ()
        n1229 = call "SW_Get_1D_Array_normalize.vi"("1D array"=w1713) -> ("Normalized 1D array"=w1712:dbl[])  [unwired: 2 in, 1 out]
        n1230 = call "SW_Get_1D_Array_normalize.vi"("1D array"=w1716) -> ("Normalized 1D array"=w1719:dbl[])  [unwired: 2 in, 1 out]
        n1231 = case shown="1" w1721 {
          tunnel: [w1796 w1797 w1798 w1799] -> w1724
          tunnel: w1723 -> [_ w1797 _ _]
          tunnel: w1719 -> [_ _ w1798 _]
          tunnel: w1712 -> [_ _ _ w1799]
          frame 0, Default {
            n1232 = global read "SW_Globals.vi" "Zones normalized allocation array"() -> (w1796:dbl[])
          }
          frame 1 {
          }
          frame 2 {
          }
          frame 3 {
          }
        }
        "Histograms (normalized)" <- w1724
        n1233 = for {
          tunnel: w1730 -> [w1803] mode=indexing
          shift-right: [w1802] -> w1728
          shift-left: 0.0 -> [w1801]
          n1234 = Add(x=w1801, y=w1803) -> (x+y=w1802:dbl)
        }
        n1235 = Build Array(w1720) -> (w1771:dbl[])
        n1236 = Multiply(x=w1728, y=100.0) -> (x*y=→"Mouse running, perc. of time":dbl)
        n1237 = Bundle By Name("t0"=w1756, "Y"=w1771) -> (→"Mouse speed":waveform(dbl))  [unwired: 1 in]
      }
      frame "Analysis" {
        n1238 = Unbundle By Name(w2065) -> ("Has been recorded"=w2067:refnum<notifier>)
        n1239 = Unbundle By Name(w2065) -> ("Data loaded"=w2074:refnum<notifier>)
        n1240 = global read "SW_Globals.vi" "Density map with no zones and with full track"() -> (w2049:picture)
        n1241 = global read "SW_Globals.vi" "Density map with zones and full track"() -> (w2048:picture)
        n1242 = global read "SW_Globals.vi" "Density map no zones"() -> (w2051:picture)
        n1243 = global read "SW_Globals.vi" "Density map with zones"() -> (w2050:picture)
        n1244 = event shown="[1] \"Zones (analysis)\", \"Show full track (analysis)\", \"Show heatmap (analysis)\": Value Change" {
          selector: _ -> [_ _]
          dyn-events: _ -> [_ _]
          timeout: 0 -> [_ _]
          tunnel: "Zones (analysis)" -> [_ w2080]
          tunnel: "Show full track (analysis)" -> [_ w2079]
          tunnel: "Show heatmap (analysis)" -> [_ w2077]
          event Timeout {
            n1245 = event-data() -> ()  [unwired: 1 in, 3 out]
          }
          event "Zones (analysis)", "Show full track (analysis)", "Show heatmap (analysis)": Value Change {
            n1246 = event-data() -> ()  [unwired: 1 in, 6 out]
            n1247 = Build Array(w2080, w2079, w2077) -> (w2078:bool[])
            n1248 = Boolean Array To Number(Boolean array=w2078) -> (number=w2076:u32)
            n1249 = property on="Map index (analysis)" class="DigNum (strict)"("Value"=w2076) -> ()  [unwired: 2 in, 2 out]
          }
        }
        n1250 = global read "SW_Globals.vi" "Full track with zones"() -> (w2052:picture)
        n1251 = global read "SW_Globals.vi" "Full track with no zones"() -> (w2053:picture)
        n1252 = global read "SW_Globals.vi" "Diagram"() -> (w2054:picture)
        n1253 = global read "SW_Globals.vi" "Diagram no zones"() -> (w2055:picture)
        n1254 = Get Notifier Status(notifier=w2074) -> (current notification=w2072:bool)  [unwired: 1 in, 4 out]
        n1255 = Get Notifier Status(notifier=w2067) -> (current notification=w2064:bool)  [unwired: 1 in, 4 out]
        n1256 = Build Array(w2055, w2054, w2053, w2052, w2051, w2050, w2049, w2048) -> (w2061:picture[])
        n1257 = Not(x=w2064) -> (.not. x?=w2066:bool)
        n1258 = Index Array(array=w2061, index="Map index (analysis)") -> (element=w2060:picture)
        n1259 = disable-structure shown="Enabled" {
          frame Enabled {
            n1260 = event shown="[2] \"Back to Settings\": Value Change" {
              selector: _ -> [_ _ _]
              dyn-events: _ -> [_ _ _]
              timeout: 0 -> [_ _ _]
              event Timeout {
                n1261 = event-data() -> ()  [unwired: 1 in, 3 out]
              }
              event "Play/Pause": Value Change {
                n1262 = event-data() -> ("NewVal"=w2082:bool)  [unwired: 1 in, 5 out]
                n1263 = case shown="True" w2082 {
                  frame False {
                    n1264 = property on="Back to Settings" class="Bool (strict)"("DisabledEnum"=T10."Enabled" ("Disabled")) -> ()  [unwired: 2 in, 2 out]
                  }
                  frame True {
                    n1265 = property on="Back to Settings" class="Bool (strict)"("DisabledEnum"=T10."Disabled and Grayed Out" ("Disabled")) -> ()  [unwired: 2 in, 2 out]
                  }
                }
              }
              event "Back to Settings": Value Change {
                n1266 = event-data() -> ("NewVal"=w2085:bool)  [unwired: 1 in, 5 out]
                n1267 = case shown="True" w2085 {
                  frame False {
                  }
                  frame True {
                    w2086 = FALSE ("Visible")
                    w2107 = enum32{"Settings", "Recording", "Analysis"}."Settings" ("Main tab control")
                    w2103 = enum32{"Settings", "Recording", "Analysis"}."Recording" ("Main tab control")
                    w2094 = enum32{"Settings", "Recording", "Analysis"}."Analysis" ("Main tab control")
                    n1268 = property on="Diagram at recording" class="Pict" props=["Bounds"]() -> (error out=w2091:errorcluster)  [unwired: 2 in, 2 out]
                    n1269 = property on="Main tab control" class="TabCtl (strict)"(error in=w2091, "Value"=w2094) -> (error out=w2098:errorcluster, "Pages"=w2093:refnum<vi>[])  [unwired: 1 in, 1 out]
                    n1270 = To Long Integer(number=w2094) -> (32bit integer=w2095:i32)
                    n1271 = Index Array(array=w2093, index=w2095) -> (element=w2096:refnum<vi>)
                    n1272 = property class="Page"(reference=w2096, error in=w2098, "PageEnb"=T28."Page Disabled & Grayed" ("Page Enabled State")) -> (error out=w2105:errorcluster)  [unwired: 1 out]
                    n1273 = property on="Main tab control" class="TabCtl (strict)"(error in=w2105, "Value"=w2103) -> (error out=w2099:errorcluster, "Pages"=w2104:refnum<vi>[])  [unwired: 1 in, 1 out]
                    n1274 = To Long Integer(number=w2103) -> (32bit integer=w2102:i32)
                    n1275 = Index Array(array=w2104, index=w2102) -> (element=w2101:refnum<vi>)
                    n1276 = property class="Page"(reference=w2101, error in=w2099, "PageEnb"=T28."Page Disabled & Grayed" ("Page Enabled State")) -> (error out=w2112:errorcluster)  [unwired: 1 out]
                    n1277 = property on="Main tab control" class="TabCtl (strict)"(error in=w2112, "Value"=w2107) -> (error out=w2111:errorcluster, "Pages"=w2106:refnum<vi>[])  [unwired: 1 in, 1 out]
                    n1278 = To Long Integer(number=w2107) -> (32bit integer=w2108:i32)
                    n1279 = Index Array(array=w2106, index=w2108) -> (element=w2109:refnum<vi>)
                    n1280 = property class="Page"(reference=w2109, error in=w2111, "PageEnb"=T28."Page Enabled" ("Page Enabled State")) -> (error out=w2092:errorcluster)  [unwired: 1 out]
                    n1281 = global read "SW_Globals.vi" "Cluster of paths"() -> (w2090:T19)
                    n1282 = property on="Back to Settings" class="Bool (strict)"(error in=w2092, "Visible"=w2086, "Value"=w2086) -> (error out=w2088:errorcluster)  [unwired: 1 in, 1 out]
                    n1283 = Unbundle By Name(w2090) -> ("Path to the settings file"=w2089:path)
                    n1284 = call <vilib>:"Open Config Data.vi"("error in (no error)"=w2088, "configuration file path"=w2089) -> ("refnum"=w2087:T4)  [unwired: 7 in, 2 out]
                    n1285 = local write "Settings file refnum out"(w2087) -> ()
                  }
                }
              }
            }
          }
          frame Disabled {
          }
        }
        n1286 = Or(x=w2066, y=w2072) -> (x .or. y?=w2068:bool)
        n1287 = And(x=w2072, y="Play/Pause") -> (x .and. y?=w2075:bool)
        n1288 = Not(x="Play/Pause") -> (.not. x?=w2070:bool)
        n1289 = And(x=w2068, y=w2070) -> (x .and. y?=w2069:bool)
        n1290 = case shown="True" w2075 {
          tunnel: w2060 -> [w2152 w2199]
          tunnel: "Zones (analysis)" -> [_ w2198]
          tunnel: [w2152 w2197] -> w2073
          tunnel: w2063 -> [_ w2177]
          frame False {
          }
          frame True {
            n1291 = disable-structure shown="Disabled" {
              frame Disabled {
                (unwired) "%<%H:%M:%S%3u%p%d.%m.%Y>T" ("format string")
                n1292 = Get Date/Time In Seconds() -> (seconds since 1Jan1904=w2219:timestamp)
                n1293 = Scan From String(default 1=w2219) -> ()  [unwired: 5 in, 3 out]
              }
              frame Enabled {
              }
            }
            n1294 = Divide(x=u32 1000, y=w2177) -> (x/y=w2179:dbl)
            n1295 = local read "TTL outputs"() -> (w2167:u8[])
            n1296 = local read "TTL inputs"() -> (w2168:u8[])
            n1297 = Multiply(x=w2179, y="Trace in analysis, s") -> (x*y=w2170:dbl)
            n1298 = local read "Absolute timestamp (rec)"() -> (w2186:dbl[])
            n1299 = local read "Relative timestamp (rec)"() -> (w2195:dbl[])
            n1300 = local read "alpha rot. angle"() -> (w2214:dbl[])
            n1301 = property on="Timeline" class="Slide (strict)"("DisabledEnum"=T10."Enabled" ("Disabled")) -> (error out=w2188:errorcluster)  [unwired: 2 in, 1 out]
            n1302 = local read "Index of the last recorded timepoint"() -> (w2191:i32)
            n1303 = local read "Zones preference array (loaded)"() -> (w2182:dbl[][])
            n1304 = local read "X coord"() -> (w2216:dbl[])
            n1305 = local read "Y coord"() -> (w2215:dbl[])
            n1306 = property on="Open File" class="Bool"(error in=w2188, "DisabledEnum"=T10."Disabled and Grayed Out" ("Disabled")) -> ()  [unwired: 1 in, 2 out]
            n1307 = feedback #9(0.0125 ("String")) -> (w2204:dbl)
            n1308 = Select(t=FALSE, s=w2198, f=TRUE) -> (s? t:f=w2209:bool)
            n1309 = feedback #10(u16 3 ("Value")) -> (w2175:u16)
            n1310 = feedback #11(0) -> (w2166:u32)
            n1311 = Index Array(array=w2168, index=w2166) -> (element=w2165:u8)
            n1312 = Index Array(array=w2167, index=w2166) -> (element=w2164:u8)
            n1313 = Number To Boolean Array(number=w2165) -> (Boolean array=w2163:bool[])
            n1314 = Number To Boolean Array(number=w2164) -> (Boolean array=w2162:bool[])
            n1315 = Or(x=w2163, y=w2162) -> (x .or. y?=w2154:bool[])
            n1316 = Index Array(array=w2154, index=0) -> (element=→"TTL IO 1 (analysis)":bool)
            n1317 = Index Array(array=w2154, index=1) -> (element=→"TTL IO 2 (analysis)":bool)
            n1318 = Index Array(array=w2154, index=2) -> (element=→"TTL IO 3 (analysis)":bool)
            n1319 = Index Array(array=w2154, index=3) -> (element=→"TTL IO 4 (analysis)":bool)
            n1320 = Index Array(array=w2186, index=w2166) -> (element=w2185:dbl)
            n1321 = Index Array(array=w2214, index=w2166) -> (element=w2213:dbl)
            n1322 = Index Array(array=w2195, index=w2166) -> (element=w2187:dbl)
            n1323 = feedback-in #9(w2187) -> ()
            n1324 = property on="Recorded timestamp" class="DigNum (strict)"("Value"=w2187) -> ()  [unwired: 2 in, 2 out]
            n1325 = Subtract(x=w2187, y=w2204) -> (x-y=w2203:dbl)
            n1326 = Index Array(array=w2182, index (row)=w2166) -> (element=→"Zones allocation (normalized) in analysis":dbl[])  [unwired: 1 in]
            n1327 = Index Array(array=w2216, index=w2166) -> (element=w2208:dbl)
            n1328 = Index Array(array=w2215, index=w2166) -> (element=w2207:dbl)
            n1329 = To Time Stamp(1:w2185) -> (0:w2184:timestamp)
            n1330 = property on="Recorded at time" class="AbsTime (strict)"("Value"=w2184) -> ()  [unwired: 2 in, 2 out]
            n1331 = event shown="[1] \"Timeline\": Value Change" {
              selector: _ -> [_ _ _]
              dyn-events: _ -> [_ _ _]
              timeout: 1 -> [_ _ _]
              tunnel: w2187 -> [w2228 _ _]
              tunnel: w2166 -> [w2227 _ w2240]
              tunnel: [w2226 w2238 w2240] -> w2194
              tunnel: w2195 -> [_ _ _]
              tunnel: w2191 -> [_ w2231 _]
              tunnel: [w2220 w2229 w2239] -> w2173
              tunnel: w2175 -> [_ w2229 w2239]
              event Timeout {
                n1332 = event-data() -> ()  [unwired: 1 in, 3 out]
                n1333 = property on="Timeline" class="Slide (strict)"("Value"=w2228) -> ()  [unwired: 2 in, 2 out]
                n1334 = property on="Speed" class="Ring (strict)"() -> ("RingText.Text"=w2224:string, "Strings []"=w2225:string[], "StringsAndValues[]"=w2222:T38)  [unwired: 2 in, 2 out]
                n1335 = Search 1D Array(1D array=w2225, element=w2224) -> (index of element=w2223:i32)  [unwired: 1 in]
                n1336 = Index Array(array=w2222, index=w2223) -> (element=w2221:cluster{"String":string, "Value":u16})
                n1337 = Unbundle(w2221) -> ("Value"=w2220:u16)  [unwired: 1 out]
                n1338 = Add(x=w2220, y=w2227) -> (x+y=w2226:u32)
              }
              event "Timeline": Value Change {
                n1339 = event-data() -> ("NewVal"=w2236:dbl)  [unwired: 1 in, 5 out]
                n1340 = property on="Timeline" class="Slide (strict)"() -> ("Scale.Maximum"=w2237:dbl, "Scale.Minimum"=w2235:dbl)  [unwired: 2 in, 2 out]
                n1341 = Subtract(x=w2236, y=w2235) -> (x-y=w2234:dbl)
                n1342 = Subtract(x=w2237, y=w2235) -> (x-y=w2233:dbl)
                n1343 = Divide(x=w2234, y=w2233) -> (x/y=w2232:dbl)
                "ceil(x): smallest int >= x" <- w2232
                n1344 = Multiply(x=w2232, y=w2231) -> (x*y=w2230:dbl)
                n1345 = To Unsigned Long Integer(number=w2230) -> (unsigned 32bit integer=w2238:u32)
              }
              event "Multiplyer of chart RX 2": Value Change {
                n1346 = event-data() -> ("NewVal"=w2241:u8)  [unwired: 1 in, 5 out]
                n1347 = Multiply(x=w2241, y=10.0) -> (x*y=w2242:dbl)
                n1348 = property on="Mouse speed 2" class="WFChart (strict)"() -> (error out=w2243:errorcluster, "XScale.Maximum"=w2246:dbl)  [unwired: 2 in, 1 out]
                n1349 = Subtract(x=w2246, y=w2242) -> (x-y=w2244:dbl)
                n1350 = property on="Mouse speed 2" class="WFChart (strict)"(error in=w2243, "XScale.Minimum"=w2244) -> ()  [unwired: 1 in, 2 out]
              }
            }
            n1351 = call "FL_Calc_speed_on_the_fly.vi"("Y coord, mm"=w2207, "X coord, mm"=w2208, "Time per frame, s"=w2203) -> ("Mouse speed, mm/s"=w2201:dbl)
            "Mouse speed digi 2" <- w2201
            n1352 = To Time Stamp(1:w2187) -> (0:w2205:timestamp)
            n1353 = Build Array(w2201) -> (w2206:dbl[])
            n1354 = Bundle By Name("t0"=w2205, "Y"=w2206) -> (→"Mouse speed 2":waveform(dbl))  [unwired: 1 in]
            n1355 = feedback-in #10(w2173) -> ()
            n1356 = Greater Or Equal?(x=w2194, y=w2191) -> (x >= y?=w2183:bool)
            n1357 = Divide(x=w2173, y=u16 3) -> (x/y=w2169:dbl)
            n1358 = Divide(x=w2170, y=w2169) -> (x/y=w2171:dbl)
            n1359 = Select(t=u32 0, s=w2183, f=w2194) -> (s? t:f=w2193:u32)
            n1360 = feedback-in #11(w2193) -> ()
            n1361 = property on="Diagram at analysis" class="Pict"() -> ("Bounds"=w2218:T16)  [unwired: 2 in, 2 out]
            n1362 = local read "Pixels per mm"() -> (w2217:dbl)
            n1363 = Round To Nearest(number=w2171) -> (nearest integer value=w2176:dbl)
            n1364 = call "SW_Draw_mouse_br.vi"("Input picture (background)"=w2199, "Size of the image"=w2218, "Pixels per mm"=w2217, "Mouse coord cartesian X, mm"=w2208, "Mouse coord cartesian Y, mm"=w2207, "Mouse angle of rotation, deg"=w2213, "Show mouse lineout"=w2209, "Trace length, samples"=w2176) -> ("Output picture (with mouse overlay)"=w2197:picture)  [unwired: 6 in, 1 out]
          }
        }
        "Diagram at analysis" <- w2073
        n1365 = case shown="True" w2069 {
          tunnel: w2065 -> [_ w2115]
          frame False {
          }
          frame True {
            n1366 = case "Open new file" shown="True" "Open File" {
              tunnel: w2115 -> [_ w2118]
              frame False {
              }
              frame True {
                n1367 = global read "SW_Globals.vi" "Cluster of paths"() -> (w2119:T19)
                n1368 = Unbundle By Name(w2119) -> ("Final csv output path"=w2129:path)
                n1369 = Strip Path(path=w2129) -> (stripped path=w2128:path)  [unwired: 1 out]
                n1370 = Strip Path(path=w2128) -> (stripped path=w2125:path)  [unwired: 1 out]
                n1371 = call "File Dialog"("start path"=w2125, "button label"="Open track", "pattern (all files)"="*.csv; *.tsv") -> ("selected path"=w2120:path, "exists"=w2124:bool, "cancelled"=w2122:bool)  [unwired: 9 in, 1 out]
                n1372 = Not(x=w2122) -> (.not. x?=w2123:bool)
                n1373 = And(x=w2124, y=w2123) -> (x .and. y?=w2121:bool)
                n1374 = case shown="True" w2121 {
                  tunnel: w2120 -> [_ w2134]
                  tunnel: w2119 -> [_ w2133]
                  tunnel: w2118 -> [_ w2130]
                  frame False {
                  }
                  frame True {
                    n1375 = flat-sequence {
                      tunnel: w2134 -> [w2136]
                      tunnel: [w2136] -> w2132
                      tunnel: [w2135] -> w2131
                      tunnel: w2133 -> [w2144]
                      tunnel: w2132 -> [w2143]
                      tunnel: w2131 -> [w2142]
                      tunnel: w2130 -> [w2151]
                      frame #0 {
                        n1376 = call <vilib>:"Get File Extension.vi"("file"=w2136) -> ("filename without extension"=w2140:string)  [unwired: 6 in, 4 out]
                        n1377 = Concatenate Strings(w2140, ".trset" ("string")) -> (w2137:string)
                        n1378 = Strip Path(path=w2136) -> (stripped path=w2138:path)  [unwired: 1 out]
                        n1379 = Build Path(base path=w2138, name or relative path=w2137) -> (appended path=w2135:path)
                        "Settings file path" <- w2135
                        "Track path" <- w2136
                      }
                      frame #1 {
                        n1380 = Bundle By Name(cluster=w2144, "Final csv output path"=w2143, "Recording settings output path"=w2142) -> (w2141:T19)
                        n1381 = global write "SW_Globals.vi" "Cluster of paths"(w2141) -> ()
                      }
                      frame #2 {
                        n1382 = Unbundle By Name(w2151) -> ("Final CSV saved"=w2147:refnum<notifier>, "Data loaded"=w2150:refnum<notifier>, "Has been recorded"=w2145:refnum<notifier>)
                        n1383 = Send Notification(notification=TRUE, notifier=w2147) -> ()  [unwired: 1 in, 2 out]
                        n1384 = Send Notification(notification=FALSE, notifier=w2150) -> ()  [unwired: 1 in, 2 out]
                        n1385 = Send Notification(notification=TRUE, notifier=w2145) -> ()  [unwired: 1 in, 2 out]
                      }
                    }
                  }
                }
              }
            }
            n1386 = property on="Open File" class="Bool"("DisabledEnum"=T10."Enabled" ("Disabled")) -> (error out=w2113:errorcluster)  [unwired: 2 in, 1 out]
            n1387 = property on="Timeline" class="Slide (strict)"(error in=w2113, "DisabledEnum"=T10."Disabled and Grayed Out" ("Disabled")) -> ()  [unwired: 1 in, 2 out]
          }
        }
      }
    }
    n1388 = Unbundle By Name(w1204) -> ("Complete stop"=w1199:refnum<notifier>)
    n1389 = Send Notification(notification="Stop Button", notifier=w1199) -> (notifier out=w1195:refnum<notifier>, error out=w1196:errorcluster)  [unwired: 1 in]
    n1390 = Get Notifier Status(notifier=w1195, error in (no error)=w1196) -> (current notification=w1197:bool)  [unwired: 4 out]
    n1391 = Or(x="Stop Button", y=w1197) -> (x .or. y?=w1198:bool)
    n1392 = node-c288() -> ()  [unwired: 1 in, 1 out]
  }
  n1393 = node-c288(w12) -> ()  [unwired: 1 out]
